vi "TLB Native Dynamic Events ver 0.26f.vi"() -> ()   [LabVIEW 2018]
uses:
  TLB Type Definitions/Intruction Type Definitions.ctl
  TLB Type Definitions/State Type Definitions, for 0.26g versions and later 2.ctl
  <vilib>/Studica/Studica Toolkit/NavX/TypeDefs/Flags/Z900_navX_Flags_OpStatusTypeDef.ctl
  <vilib>/Studica/Studica Toolkit/NavX/TypeDefs/Flags/Z900_navX_Flags_CalibrationStatusTypeDef.ctl
  TLB Type Definitions/Vision cluster.ctl
  TLB Type Definitions/PING CLUSTER.ctl
  TLB Type Definitions/Encoder cluster.ctl
  TLB Type Definitions/Stepper cluster.ctl
  TLB Type Definitions/Yaw Cluster.ctl
  TLB Type Definitions/IR Sensor Type Def.ctl
  TLB Type Definitions/Line Sensor Cluster.ctl
  TLB Type Definitions/Time cluster.ctl
  TLB Type Definitions/Box Colour Detection Cluster (0.26d and above).ctl
  Underlying VI's/FGV's/Box FGV/Box Colour FGV Colours.ctl
  <vilib>/Studica/Studica Toolkit/Background/DIO Channel.ctl
  TLB Type Definitions/Y Stepper cluster.ctl
  TLB Type Definitions/Motor Speed Cluster.ctl
  Labview Training Phase 2/Enum Controls/States for Action Engine.ctl
  Underlying VI's/NavX VI/navX type def.ctl
  <vilib>/Studica/Studica Toolkit/Background/I2C Channel.ctl
  Underlying VI's/I2C Master VI/Arduino_Interfacing.ctl
  Underlying VI's/Motor Control VI with PID/MOTOR CONTROL WITH PID AE DATA MODE TYPE DEF.ctl
  Underlying VI's/Motor Control VI with PID/MOTOR CONTROL WITH PID AE DIRECTION TYPE DEF.ctl
  Experimental VI's/Archived VI's/MOTOR CONTROL NO PID Type Def.ctl
  <vilib>/myRIO/Common/Instrument Driver Framework/myRIO v1.0/AI/typedefs/AI Channels List.ctl
  <vilib>/myRIO/Common/Instrument Driver Framework/myRIO v1.0/AI/typedefs/AI Channels Enum.ctl
  Underlying VI's/Line Sensor AE/Line Sensor AE Type Def.ctl
  Underlying VI's/I2C Master VI/I2C MASTER Type Def.ctl
  Underlying VI's/Elasped Timer/Elapsed timer control.ctl
  Underlying VI's/IMAQ Create Reference AE/IMAQ Reference AE.ctl
  Underlying VI's/FGV's/Box FGV/Box Colour FGV States.ctl
  Underlying VI's/I2C Master VI/I2C_MASTER_WRITE_NEW Type Def.ctl
  Underlying VI's/Modified webcam FGV/Webcam AE.ctl
  <vilib>/userdefined/High Color/IMAQdx.ctl
  <vilib>/Studica/Studica Toolkit/NavX/NavX.lvlib
  <vilib>/NI_Real-Time Target Support.lvlib
panel:
  out "Same colour?":bool
  out "Box Colour Detection":T1
  out "Errors detected":bool
  out "Robot ready":bool
  out "Time cluster":T3
  out "Table IR obstruct":bool
  out "Front IR obstruct":bool
  out "CPU 1 Usage":dbl
  out "CPU 0 Usage":dbl
  out "Line sensors":T4
  out "IR Sensors":T5
  out "NAVX Values":T6
  out "Stepper position values":T7
  out "Encoder values":T8
  out "Ultrasonic sensors":T9
  out "Selected Task":T10=enum."Start Task 9"
  out "Object recognition mode":enum16{"Ball", "Soap", "Gel", "Pipe", "None"}(ring)
  out "Image Processing Error":errorcluster
  out "Object Detection":T11
  out "Status":T14 {"OP Status" items=["INITIALIZING", "SELFTEST_IN_PROGRESS", "ERROR", "IMU_AUTOCAL_IN_PROGRESS", "NORMAL"]; "Calibration Status" items=["IMU_CAL_STATE_MASK"=3, "IMU_CAL_STATE_INPROGRESS"=0, "IMU_CAL_STATE_ACCUMULATE"=1, "IMU_CAL_STATE_COMPLETE"=2]}
  out "General Errors":errorcluster
  in  "Red LED":bool
  out "Front Ultrasonic obstruct":bool
  out "Speed & distance":T15
  out "Task selection":u8
  out "NavX Readings":T16
  out "Arduino Data":T17
  out "TASK ENABLE":bool
  out "Rising Edge":bool
  in  "Green LED":bool
  out "State Logic":T18=enum."Startup"
  out "elements":T10[](array[typedef])
  in  "STOP TASK":bool
  in  "OK Button":bool
  in  "STOP":bool
  out "Queue Errors":errorcluster
  out "Action Queue Items":i32
  out "State Logic Queue Items":i32
  out "Action Queues items":string[](array[string])=["Hardware reset", "Software reset", ""]
  out "Action State":string
  # "VISION"
  # "TLB FRAMEWORK STATUS"
  # "System Health Status Update"
  # "Test Programme written by Calvin Loke    Dated: 28 Aug 2019\nTest Programme revised by Dr Alex See   Dated 30 Aug 2019\n\nRevision date: 20/03/2020\nProgramme version:   TLB Native Dynamic Events ver 0.19a"
  # "0: Task 1\n1: Task 2\n2: Task 3\n3: Task 4\n4: Task 5\n5: Task 6\n6: Task 7\n7: Task 8 Ball\n8: Task 8 Soap\n9: Task 8 Gel\n10: Task 8 Pipe\n11: Task 9 Blue\n12: Task 9 Black\n13: Task 9 Green\n14: Task 9 Red\n15: Task 9 Yellow"
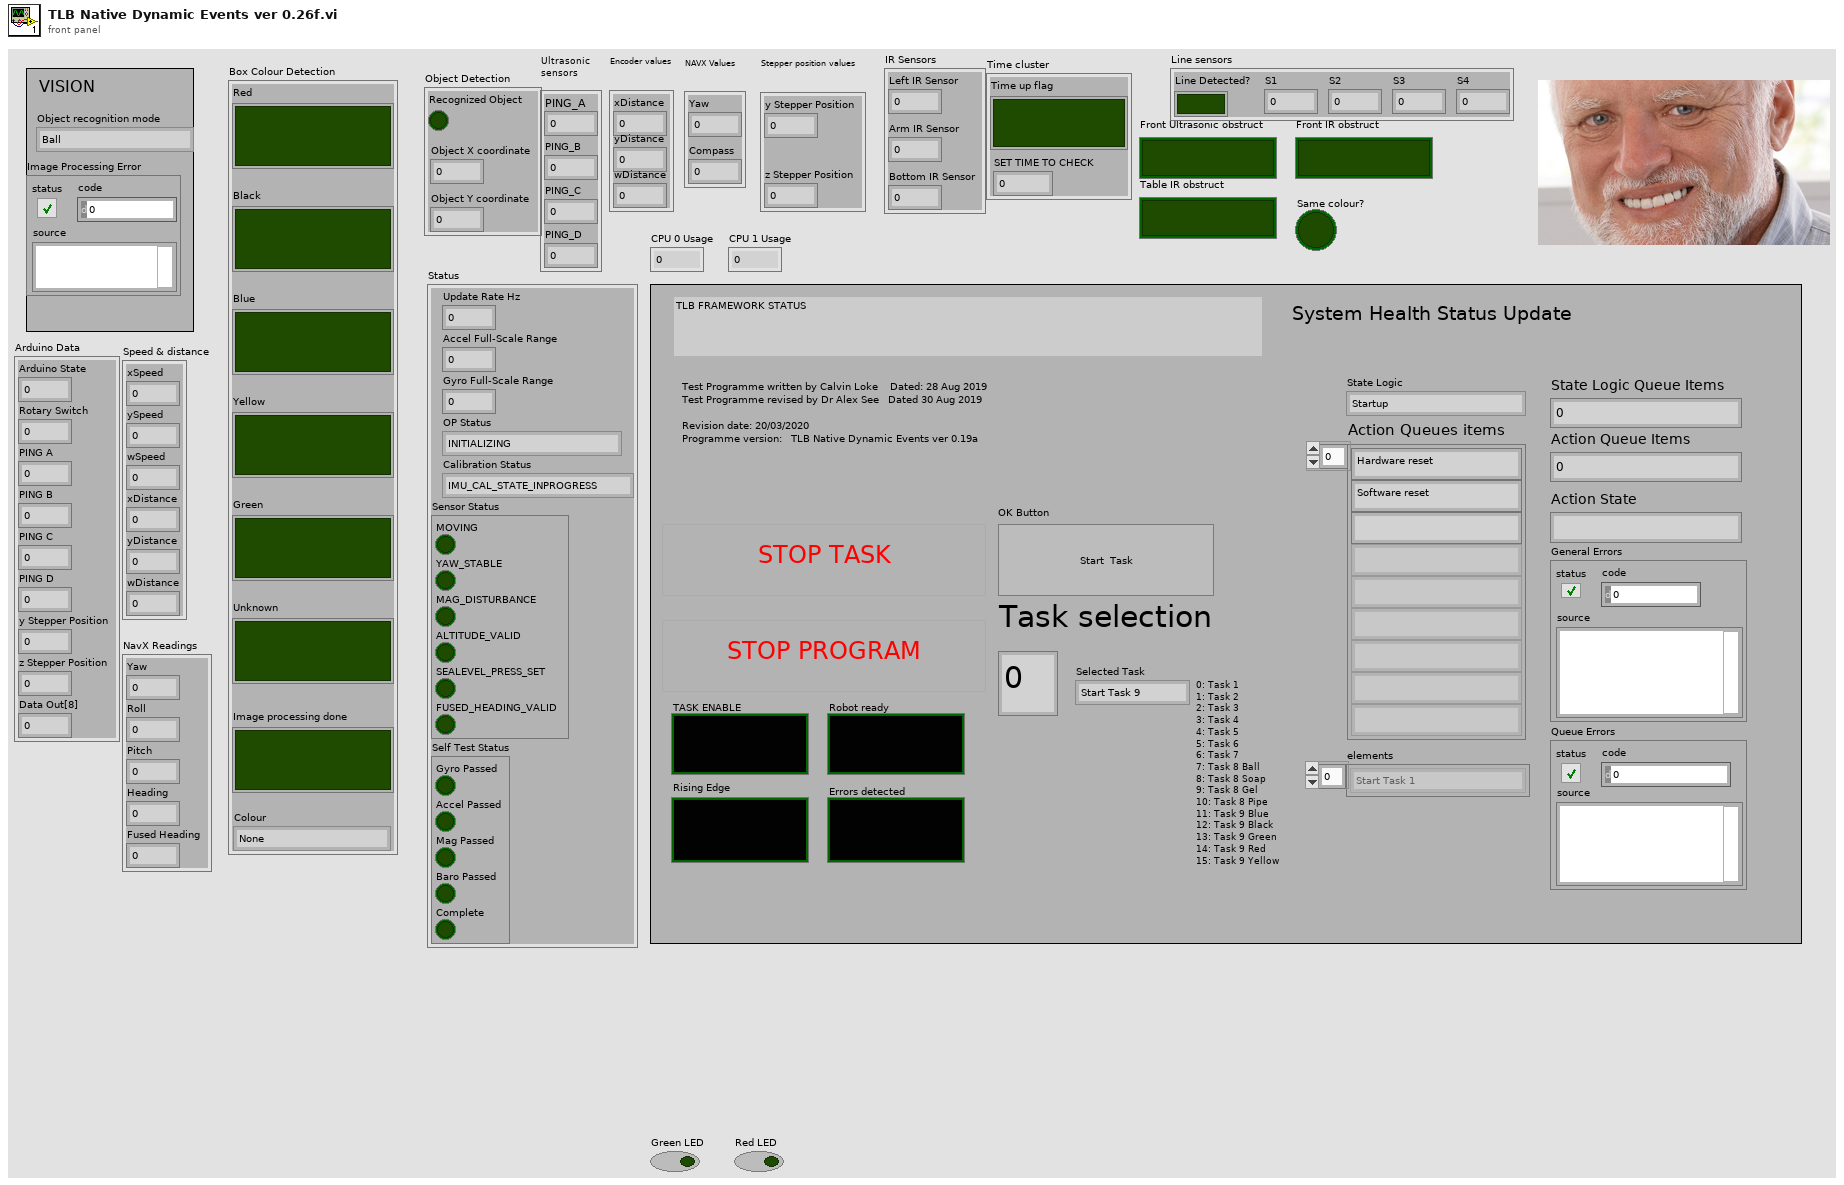
[diagram p1: front panel]
types:
  T1 = typedef "Box Colour Detection Cluster (0.26d and above).ctl" = cluster{"Red":bool, "Black":bool, "Blue":bool, "Yellow":bool, "Green":bool, "Unknown":bool, "Image processing done":bool, "Colour":T2}
  T2 = typedef "Box Colour FGV Colours.ctl" = enum16{"None", "Black", "Blue", "Green", "Red", "Yellow"}
  T3 = typedef "Time cluster.ctl" = cluster{"Time up flag":bool, "SET TIME TO CHECK":dbl}
  T4 = typedef "Line Sensor Cluster.ctl" = cluster{"Line Detected?":bool, "S1":dbl, "S2":dbl, "S3":dbl, "S4":dbl}
  T5 = typedef "IR Sensor Type Def.ctl" = cluster{"Left IR Sensor":dbl, "Arm IR Sensor":dbl, "Bottom IR Sensor":dbl}
  T6 = typedef "Yaw Cluster.ctl" = cluster{"Yaw":dbl, "Compass":dbl}
  T7 = typedef "Stepper cluster.ctl" = cluster{"y Stepper Position":u8, "z Stepper Position":u8}
  T8 = typedef "Encoder cluster.ctl" = cluster{"xDistance":dbl, "yDistance":dbl, "wDistance":dbl}
  T9 = typedef "PING CLUSTER.ctl" = cluster{"PING_A":u8, "PING_B":u8, "PING_C":u8, "PING_D":u8}
  T10 = typedef "Intruction Type Definitions.ctl" = enum16{"None", "Start Task 1", "Start Task 2", "Start Task 3", "Start Task 4", "Start Task 5", "Start Task 6", "Start Task 7", "Start Task 8 - BALL", "Start Task 8 - Gel", "Start Task 8 - Pipe", "Start Task 8 - Soap", "Start Task 9", "Start Task A", "Start Task B", "Exit"}
  T11 = typedef "Vision cluster.ctl" = cluster{"Recognized Object":bool, "Object X coordinate":dbl, "Object Y coordinate":dbl}
  T12 = typedef "NavX.lvlib/Z900_navX_Flags_OpStatusTypeDef.ctl" = u8
  T13 = typedef "NavX.lvlib/Z900_navX_Flags_CalibrationStatusTypeDef.ctl" = u8
  T14 = cluster{"Update Rate Hz":u8, "Accel Full-Scale Range":u8, "Gyro Full-Scale Range":u16, "OP Status":T12, "Calibration Status":T13, "Sensor Status":cluster{"MOVING":bool, "YAW_STABLE":bool, "MAG_DISTURBANCE":bool, "ALTITUDE_VALID":bool, "SEALEVEL_PRESS_SET":bool, "FUSED_HEADING_VALID":bool}, "Self Test Status":cluster{"Gyro Passed":bool, "Accel Passed":bool, "Mag Passed":bool, "Baro Passed":bool, "Complete":bool}}
  T15 = cluster{"xSpeed":dbl, "ySpeed":dbl, "wSpeed":dbl, "xDistance":dbl, "yDistance":dbl, "wDistance":dbl}
  T16 = cluster{"Yaw":dbl, "Roll":dbl, "Pitch":dbl, "Heading":dbl, "Fused Heading":dbl}
  T17 = cluster{"Arduino State":u8, "Rotary Switch":u8, "PING A":u8, "PING B":u8, "PING C":u8, "PING D":u8, "y Stepper Position":u8, "z Stepper Position":u8, "Data Out[8]":u8}
  T18 = typedef "State Type Definitions, for 0.26g versions and later 2.ctl" = enum16{"None", "Startup", "Move to Angle", "True Stop", "Idle", "Shutdown", "Task 1A", "Task 1B", "Task 2:Raise Arm", "Task 2:Sensor Mode", "Task 2:Reverse Mode", "Task 3", "Task 4_A", "Task 4_B", "Task 4_C", "Task 4_D", "Task 5A", "Task 5B", "Task 5C", "Task 5D", "Task 5E: POSITION ARM", "Task 5F: ARM GRAB HEIGHT", "Task 5G: CLOSE CLAW", "Task 5H: RAISE ARM", "Task 6_A", "Task 6_B", "Task 7", "Task 8A: RAISE ARM", "Task 8B: MOVE TO BOX", "Task 8C: CAM BURST", "Task 8D: PROCESS IMAGE", "Task 8E: ROBOT ADJUST", "Task 8F: CAM BURST 2", "Task 8G: PROCESS IMAGE 2", "Task 8H: ARM ADJUST", "Task 8I: ARM GRAB HEIGHT", "Task 8J: CLOSE CLAW", "Task 8K: RAISE MY SWORD", "Task 9A: Raise Arm", "Task 9B: Rotate to Angle", "Task 9C: Detect Box", "Task 9D: MOVE FORWARD", "Task 9E: MOVE LEFT", "Task 9F: SCAN BOX", "Task 9G: MOVE RIGHT", "Task 9H: SCAN BOX 2", "Task 9I: ROTATE 90 CW", "Task 9J: FORWARD", "Task 9K: MOVE RIGHT", "Task 9L: SCAN BOX 3", "Task 9M: MOVE RIGHT", "Task 9N: SCAN BOX 4", "PENIS", "PENIS 2", "PENIS 3", "Task 9R: PROCESS COLOUR", "Task A1: Task 9 Open cam", "Task A2: Task 9 Move Arm", "Task A3: Task 9 Set Timer", "Task A4: Tasl 9 Capture images", "Task A5: Task 9 Close camera", "Task A6: Process Colour", "Task A7: Dispose Camera Buffer"}
  T19 = typedef "Motor Speed Cluster.ctl" = cluster{"ySpeed":dbl, "xSpeed":dbl, "wSpeed":dbl}
  T20 = typedef "Y Stepper cluster.ctl" = cluster{"yStepper desired":u8}
  T21 = typedef "DIO Channel.ctl" = enum16{"Not Connected", "A/DIO1", "A/DIO2", "A/DIO3", "A/DIO4", "A/DIO5", "A/DIO6", "A/DIO7", "A/DIO13", "B/DIO1", "B/DIO2", "B/DIO3", "B/DIO4", "B/DIO5", "B/DIO6", "B/DIO7", "B/DIO13", "C/DIO0", "C/DIO1", "C/DIO2", "C/DIO3", "C/DIO4", "C/DIO5", "C/DIO6", "C/DIO7"}
  T22 = cluster{"DIO Channel":T21, "FPGA VI Reference Out":refnum<k20>}
  T23 = typedef "States for Action Engine.ctl" = enum16{"Initialize", "Write", "Read"}
  T24 = typedef "NI_Real-Time Target Support.lvlib/RT CPU Load.ctl" = cluster{"Total (%)":dbl, "Time Critical (%)":dbl, "Timed Structures (%)":dbl, "High (%)":dbl, "Above Normal (%)":dbl, "Normal (%)":dbl, "Background (%)":dbl, "Idle (%)":dbl, "ISR (%)":dbl}
  T25 = cluster{"CPU loads[0]":T24, "CPU loads[1]":T24, "CPU loads[2]":T24, "CPU loads[3]":T24, "CPU loads[4]":T24, "CPU loads[5]":T24, "CPU loads[6]":T24, "CPU loads[7]":T24, "CPU loads[8]":T24}
  T26 = typedef "navX type def.ctl" = enum16{"Get i2C reference", "Read Values", "Zero Yaw"}
  T27 = typedef "Arduino_Interfacing.ctl" = enum16{"Initialize", "Write to Arduino", "Read From Arduino"}
  T28 = typedef "I2C Channel.ctl" = enum16{"Not Connected", "A", "B"}
  T29 = cluster{"I2C Ref Out":cluster{"I2C Channel":T28, "FPGA VI Reference Out":refnum<k20>}, "Connected":bool, "Slave Address (7-bit)":u8, "Registry":u8[]}
  T30 = typedef "Box Colour FGV States.ctl" = enum16{"Initialize", "Read", "Write"}
  T31 = typedef "MOTOR CONTROL WITH PID AE DIRECTION TYPE DEF.ctl" = enum16{"y-axis movement", "x-axis movement", "rotation", "stop", "reset encoders"}
  T32 = typedef "MOTOR CONTROL WITH PID AE DATA MODE TYPE DEF.ctl" = enum16{"Init AE", "Write to AE", "Read from AE"}
  T33 = typedef "Line Sensor AE Type Def.ctl" = enum16{"INIT AE", "READ FROM LINE SENSORS"}
  T34 = typedef "IMAQ Reference AE.ctl" = enum16{"Initialize AE", "Get IMAQ Reference", "Dispose Processing Buffer"}
  T35 = typedef "Elapsed timer control.ctl" = enum16{"Start", "Pause", "Initialize"}
  T36 = typedef "I2C_MASTER_WRITE_NEW Type Def.ctl" = enum16{"Ultrasonic sensors", "Stepper origin", "zStepper 13.3k", "zStepper 13k", "zStepper 12k", "zStepper 11k", "zStepper 10k", "zStepper 9k", "zStepper 8k", "zStepper 7k", "zStepper 6k", "zStepper 5k", "zStepper 4k", "zStepper 3k", "zStepper 2k", "zStepper 1k", "zStepper 900", "zStepper 800", "zStepper 700", "zStepper 600", "zStepper 500", "zStepper 400", "zStepper 300", "zStepper 200", "zStepper 100", "zStepper 0", "yStepper control", "Open Claw", "Close Claw", "Soft Reset"}
  T37 = typedef "Webcam AE.ctl" = enum16{"Initialize Camera", "Open Camera", "Continuous Acquisition", "Close Camera", "Retrieve Image", "Dispose Camera Image Buffer"}
  T38 = typedef "IMAQdx.ctl" = refnum<k21>
  T39 = typedef "MOTOR CONTROL NO PID Type Def.ctl" = enum16{"Init", "Front Back", "Left Right", "Rotate", "Stop", "Latch"}
  T40 = typedef "AI Channels List.ctl" = T41[]
  T41 = typedef "AI Channels Enum.ctl" = enum16{"Not Connected", "AudioIn/Left", "AudioIn/Right", "C/AI0", "C/AI1", "A/AI0", "A/AI1", "A/AI2", "A/AI3", "A/AI4", "A/AI5", "A/AI6", "A/AI7", "B/AI0", "B/AI1", "B/AI2", "B/AI3", "B/AI4", "B/AI5", "B/AI6", "B/AI7", "AI/AI0", "AI/AI1", "AI/AI2", "AI/AI3", "A/AI0 (DIFF)", "A/AI1 (DIFF)", "A/AI2 (DIFF)", "A/AI3 (DIFF)", "B/AI0 (DIFF)", "B/AI1 (DIFF)", "B/AI2 (DIFF)", "B/AI3 (DIFF)"}
  T42 = cluster{"S1":dbl, "S2":dbl, "S3":dbl, "S4":dbl, "Array[4]":dbl, "Array[5]":dbl, "Array[6]":dbl, "Array[7]":dbl, "Array[8]":dbl}
  T43 = typedef "I2C MASTER Type Def.ctl" = enum16{"Last State", "Mode 0", "Mode 1", "Mode 2", "Mode 3", "Mode 4", "Mode 5", "Mode 6", "Mode 7", "Mode 8", "Mode 9", "Mode 10"}
  T44 = typedef "IMAQ Image.ctl" = refnum<image>
  T45 = cluster{"Number of Matches":i32, "Object detected?":bool}
  T46 = cluster{"Red":bool, "Black":bool, "Blue":bool, "Yellow":bool, "Green":bool, "No recognizable coolour":bool}
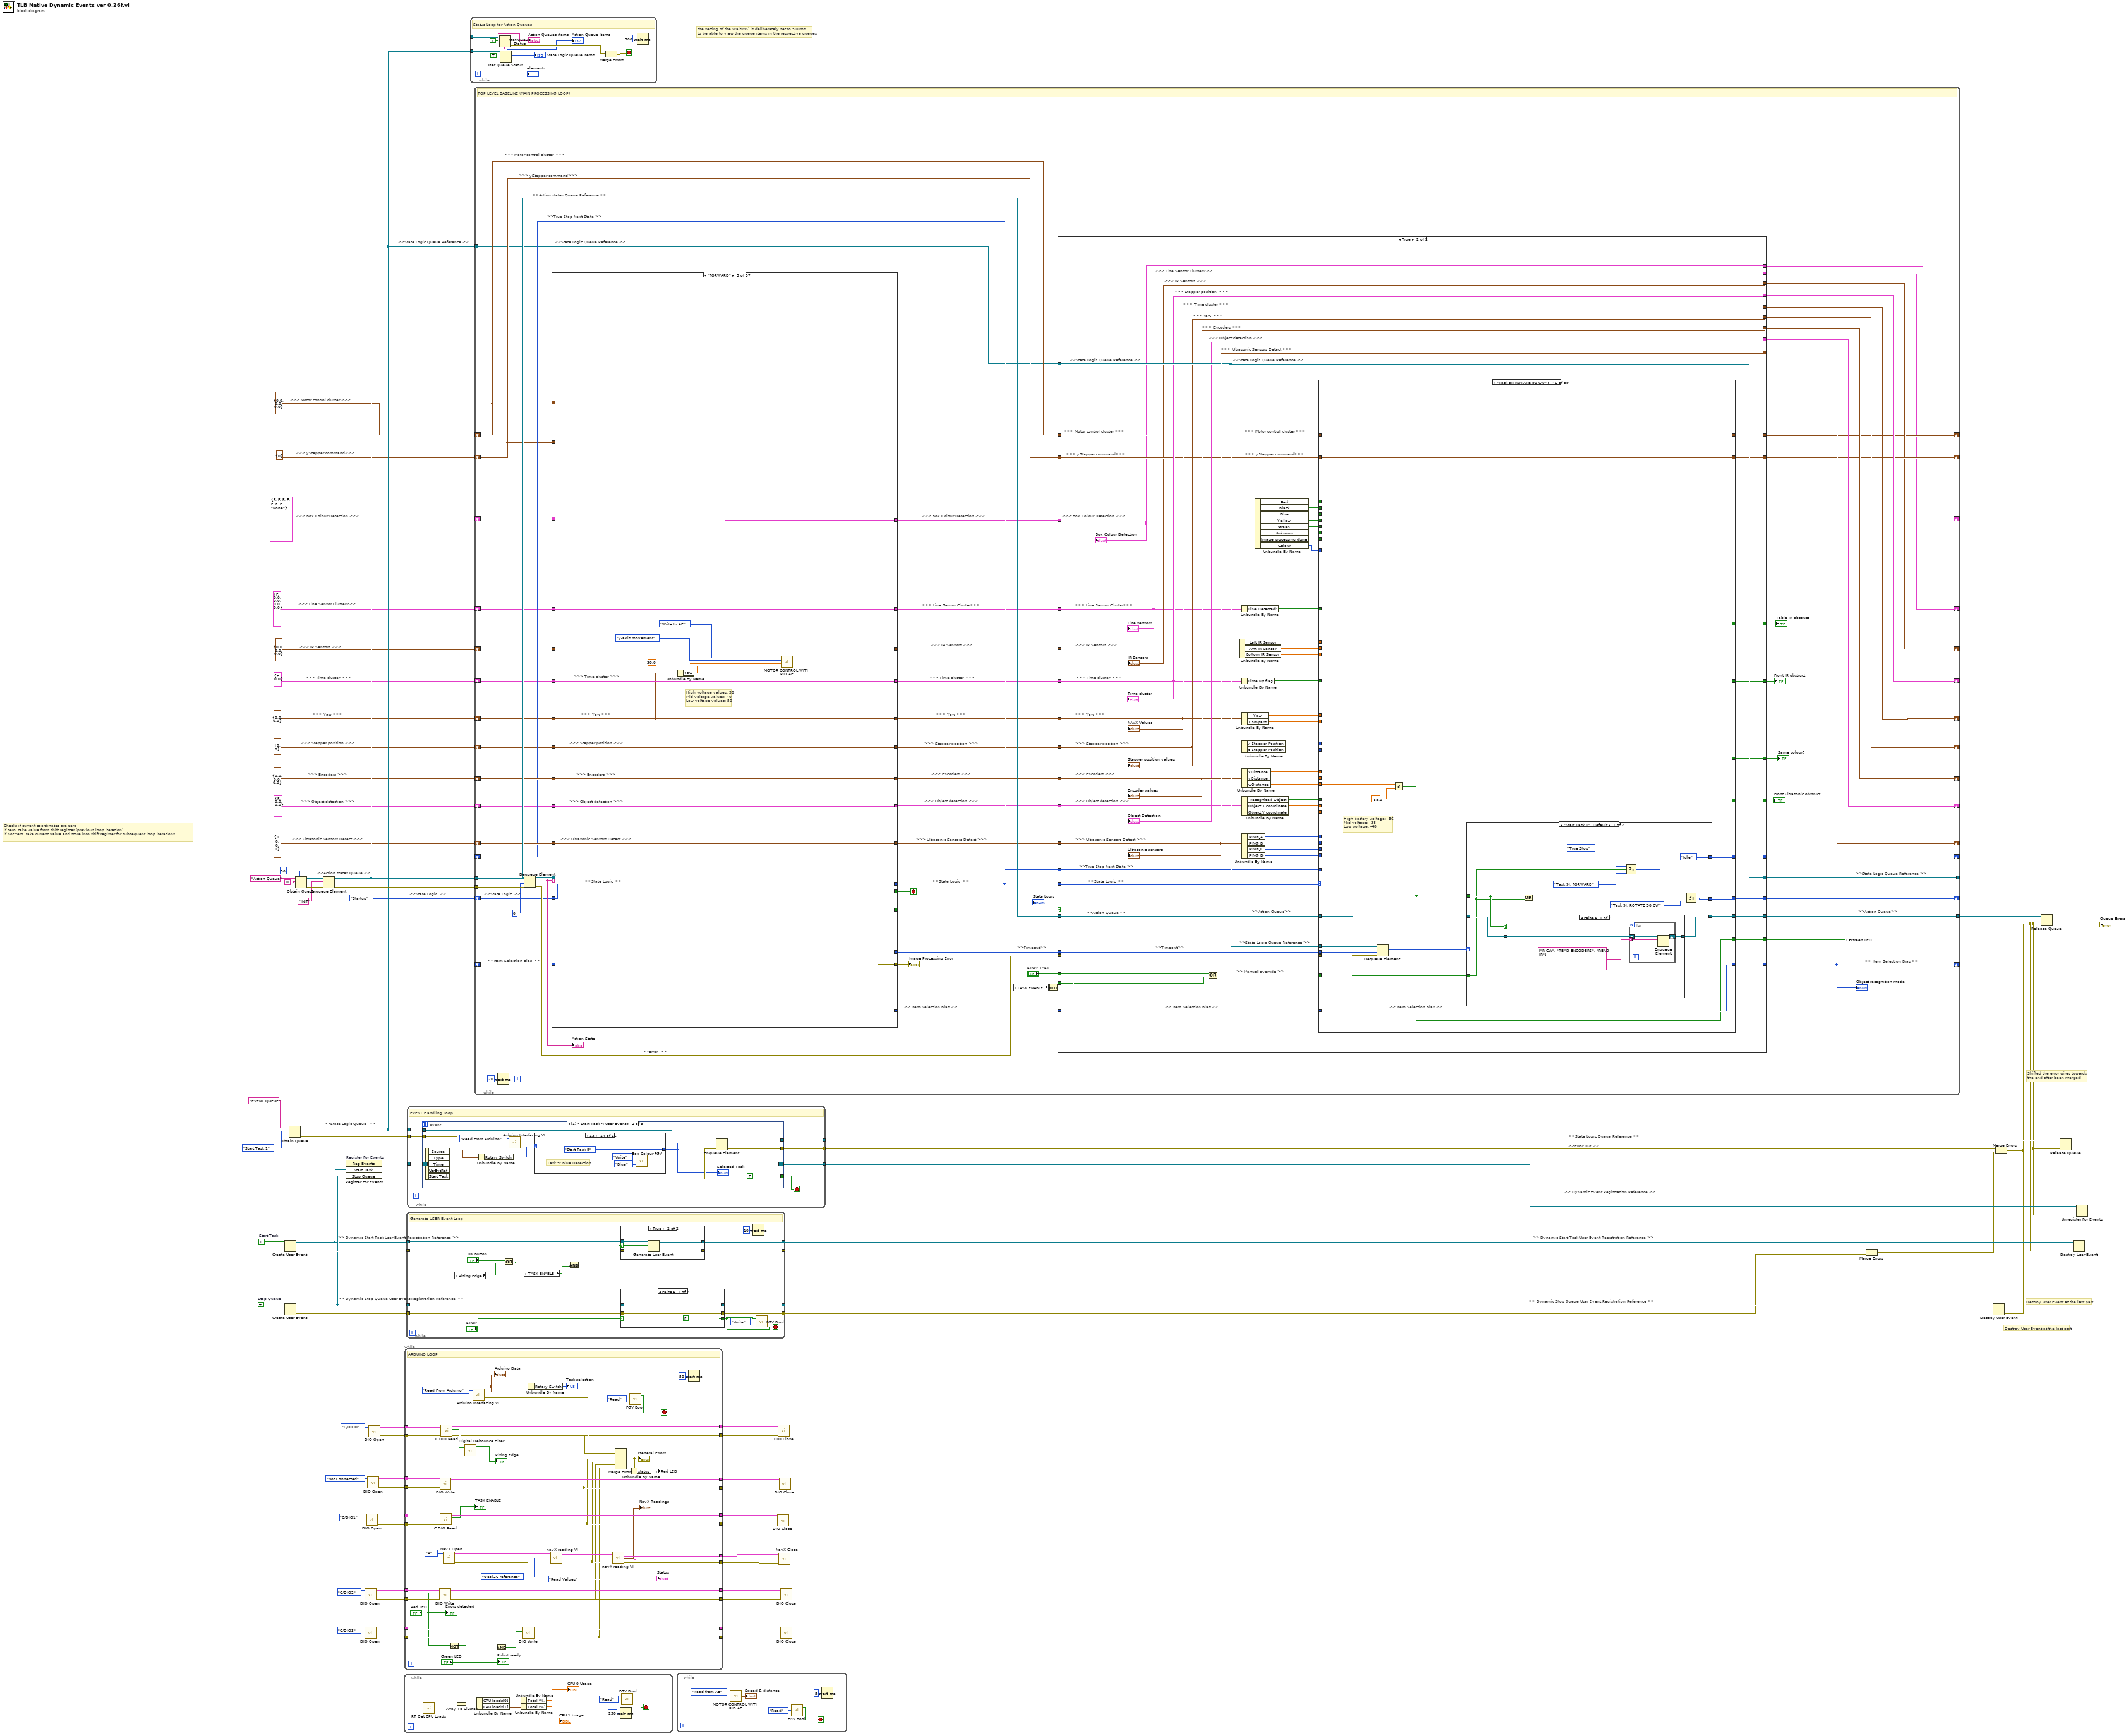
[diagram p0: block diagram]
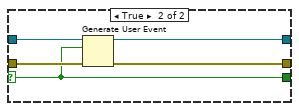
[diagram p2: hidden frame]
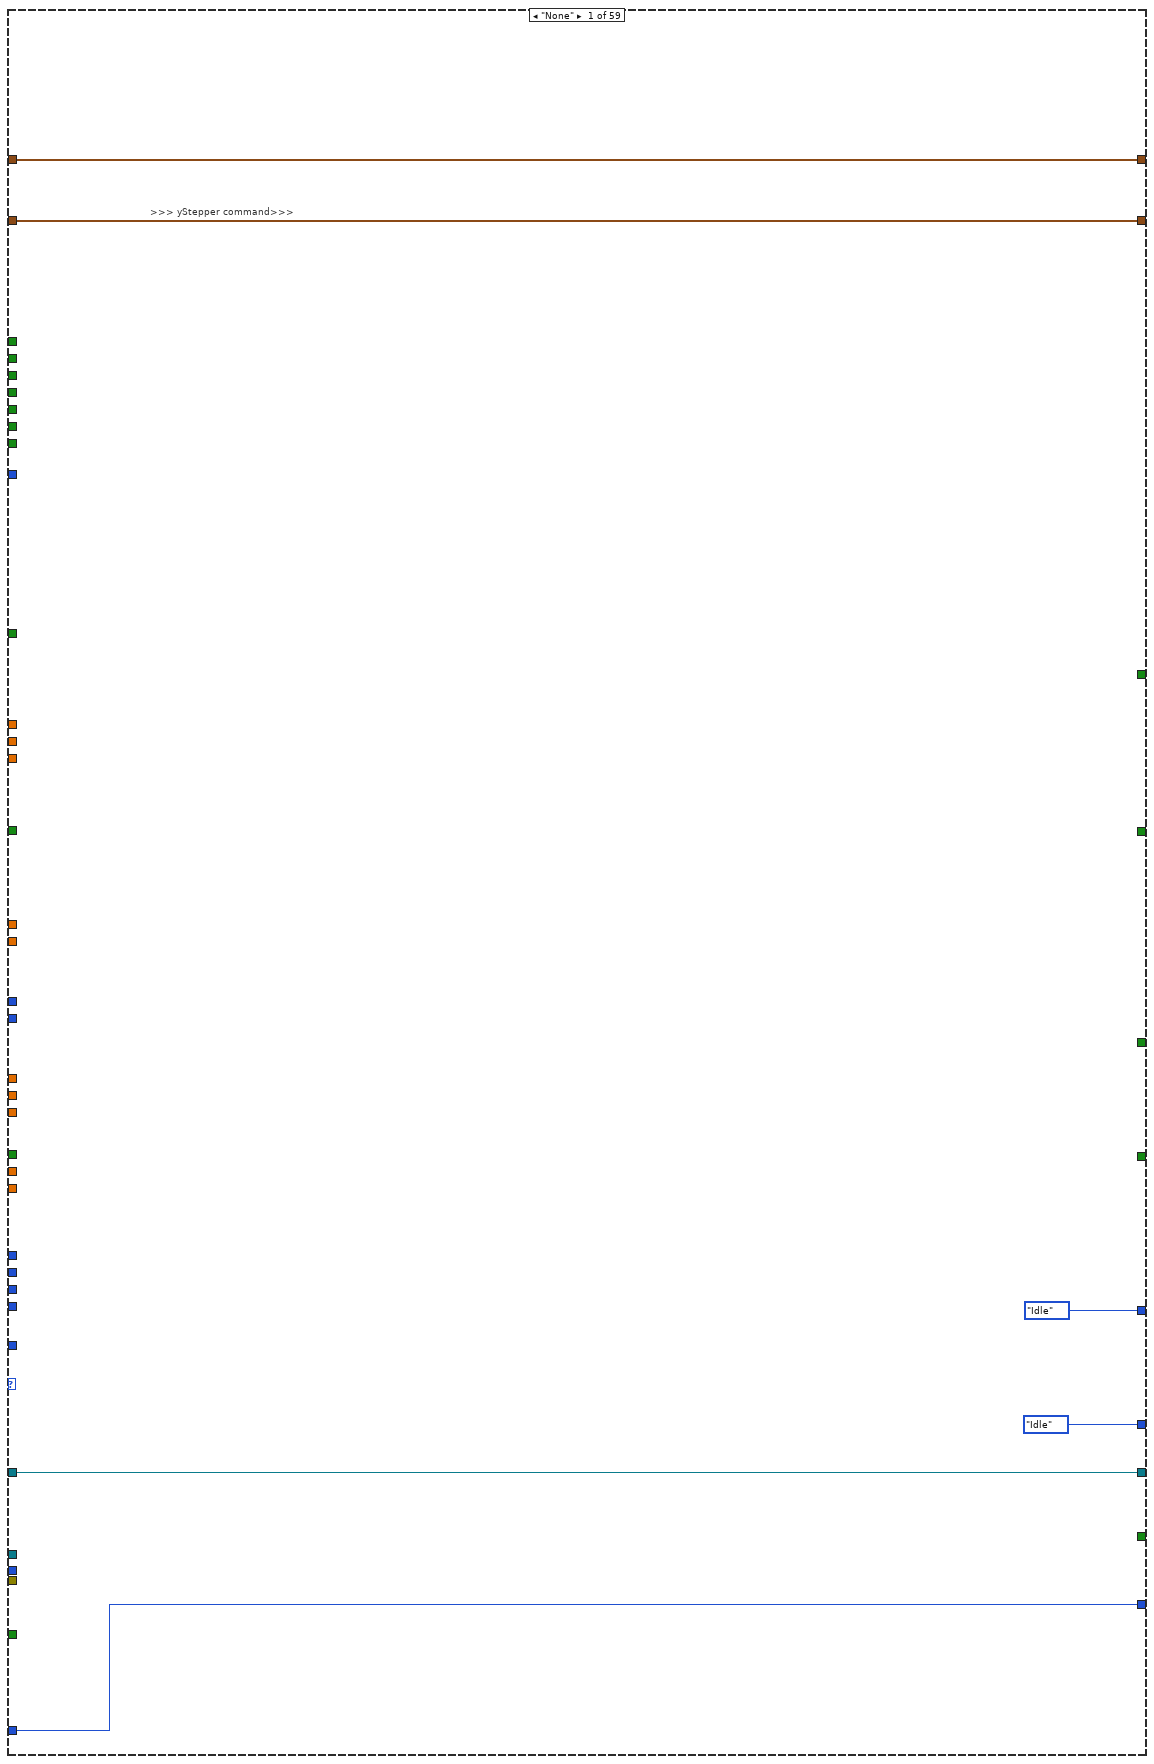
[diagram p5: hidden frame]
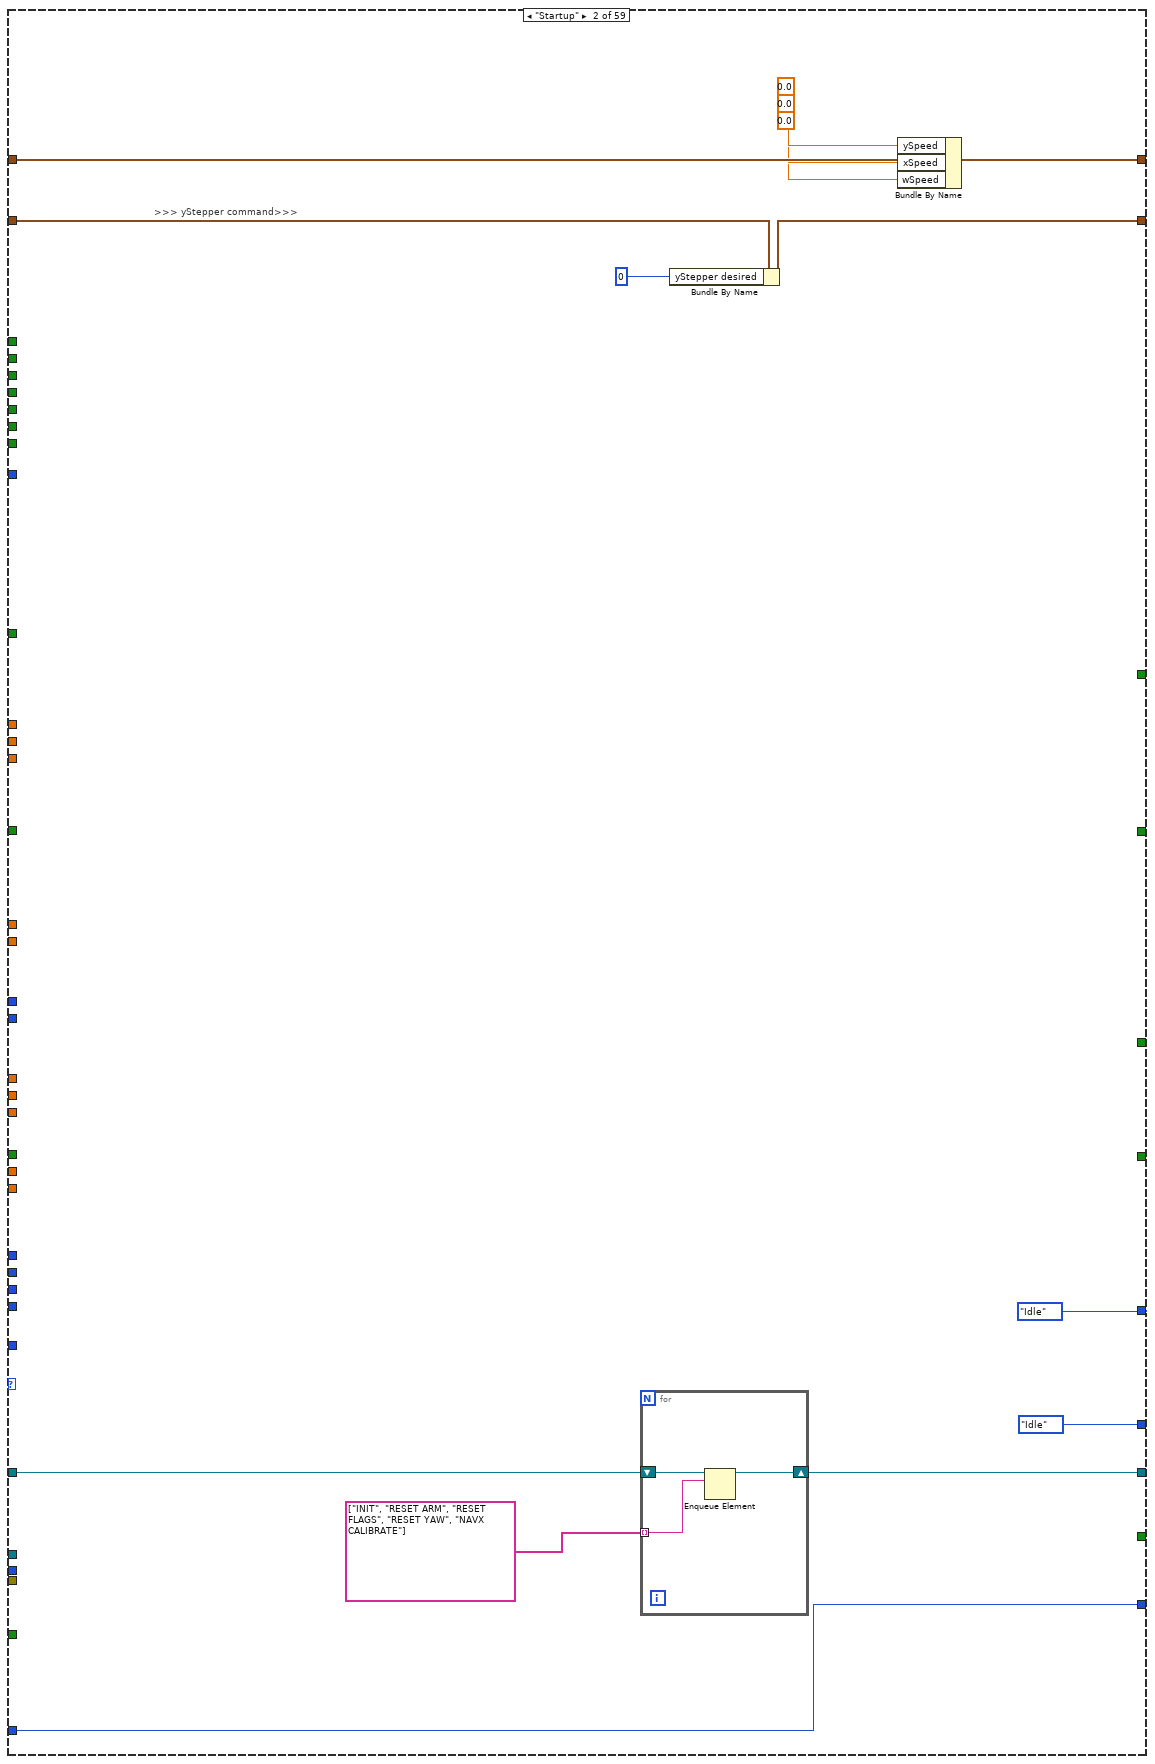
[diagram p6: hidden frame]
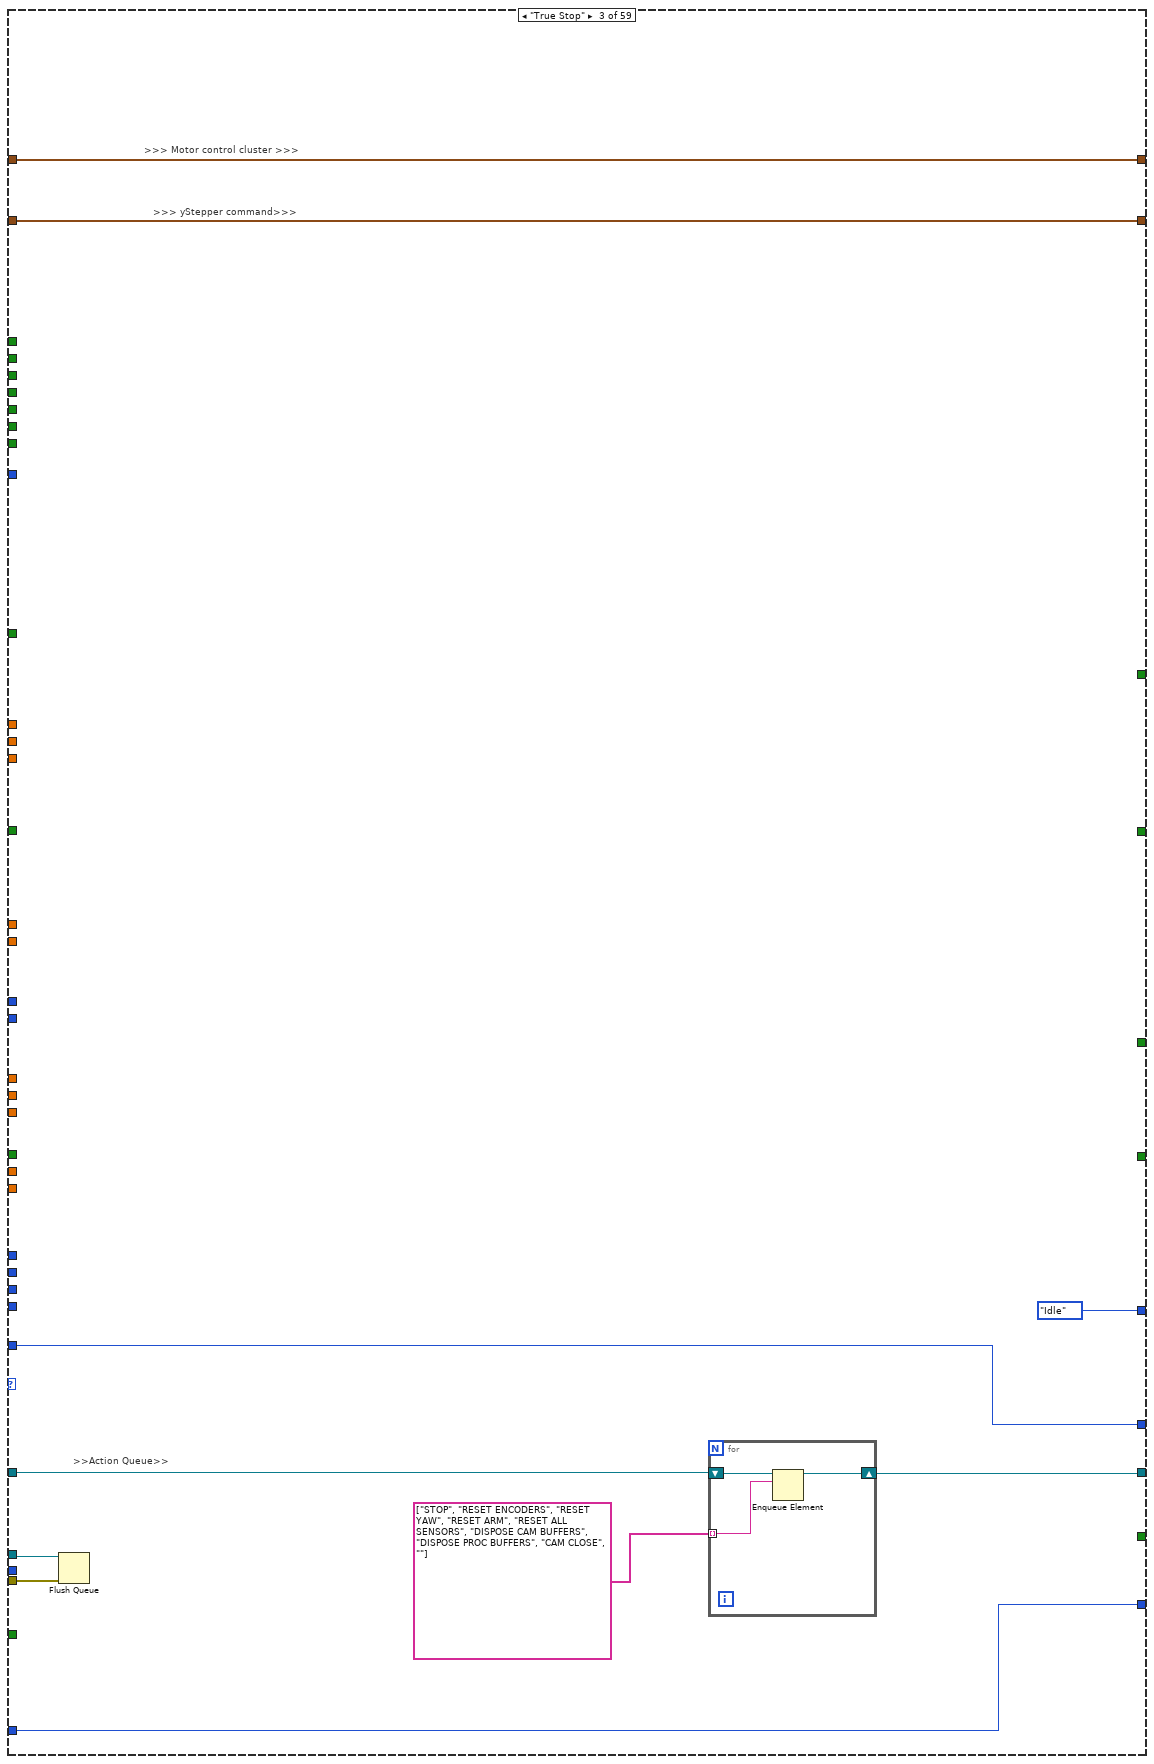
[diagram p7: hidden frame]
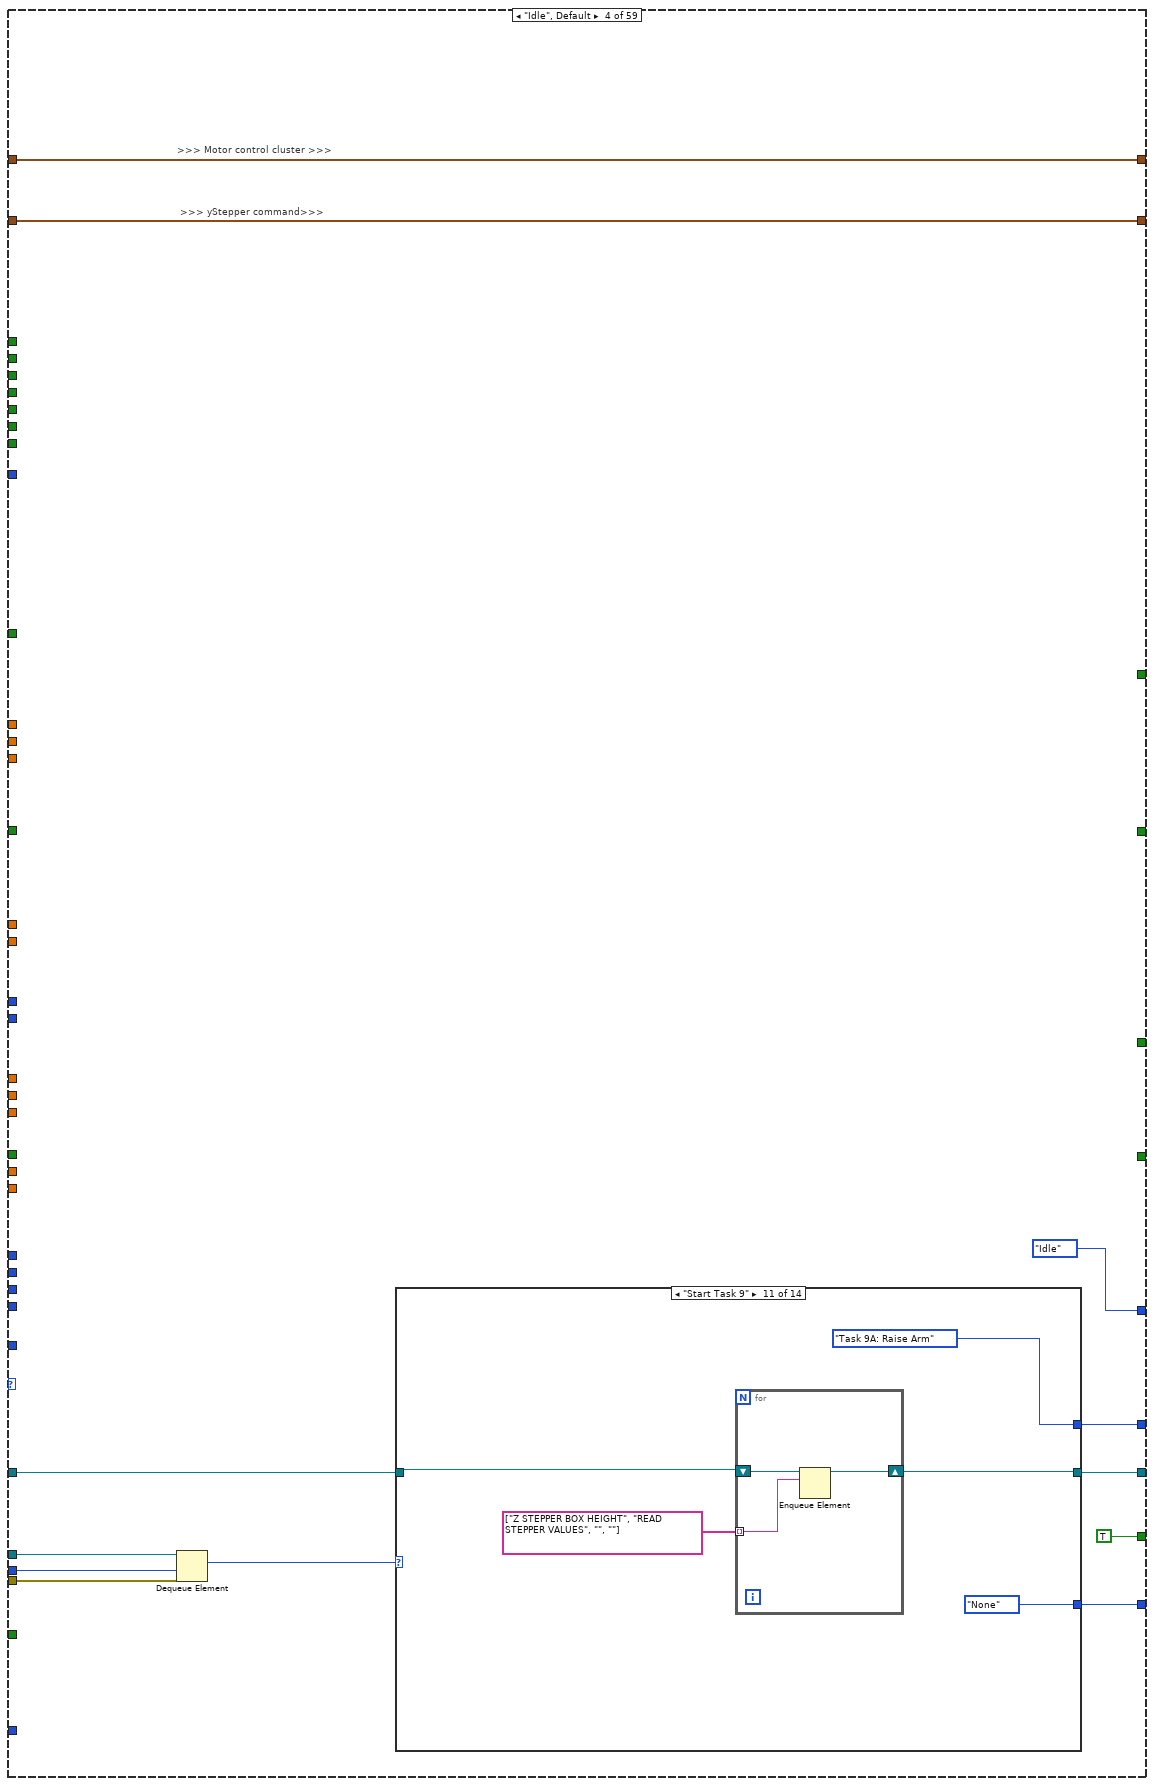
[diagram p8: hidden frame]
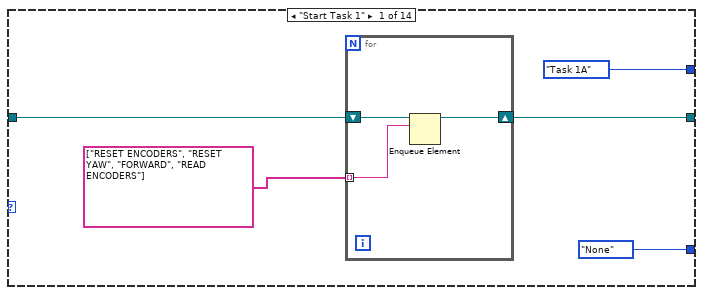
[diagram p9: hidden frame]
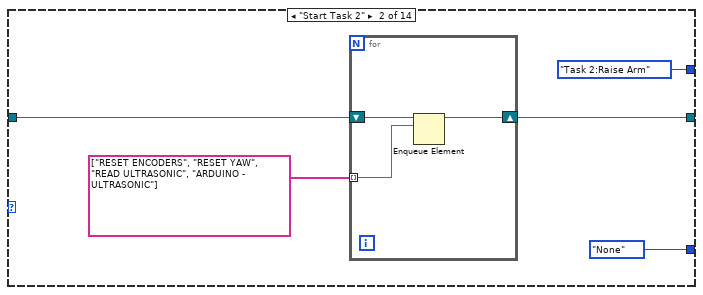
[diagram p10: hidden frame]
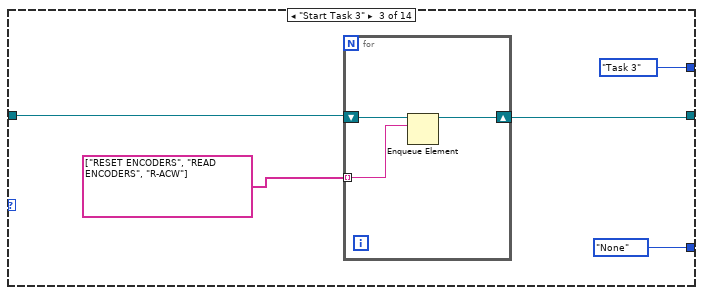
[diagram p11: hidden frame]
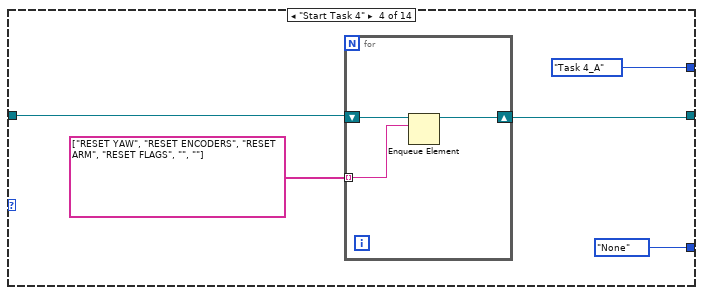
[diagram p12: hidden frame]
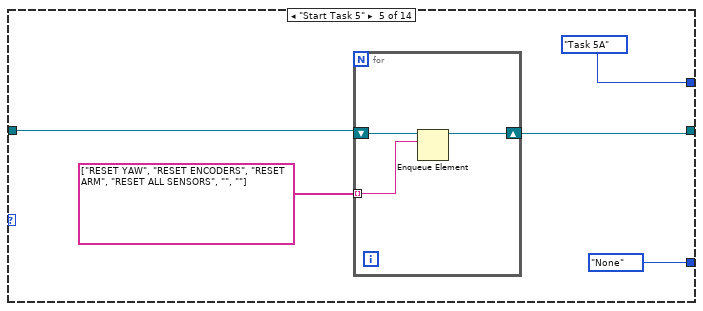
[diagram p13: hidden frame]
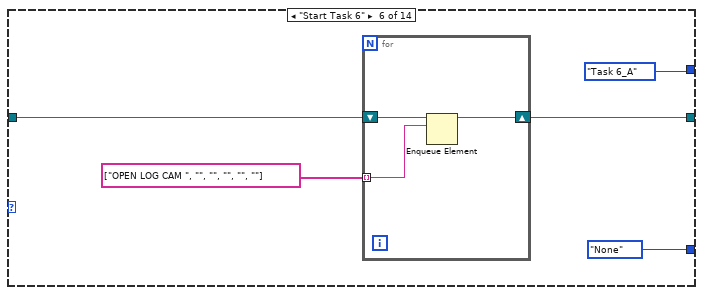
[diagram p14: hidden frame]
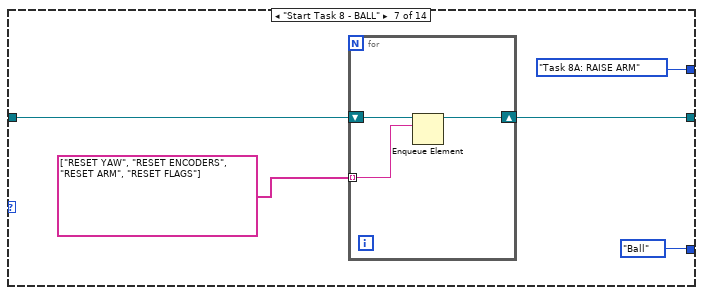
[diagram p15: hidden frame]
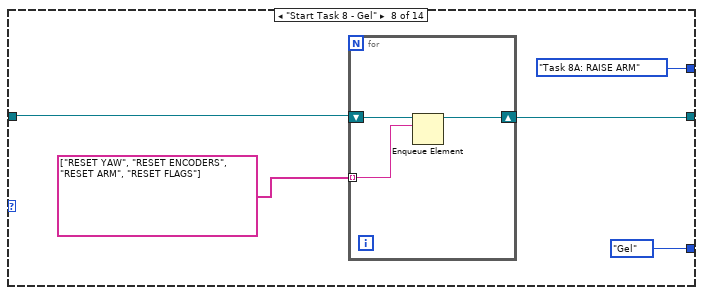
[diagram p16: hidden frame]
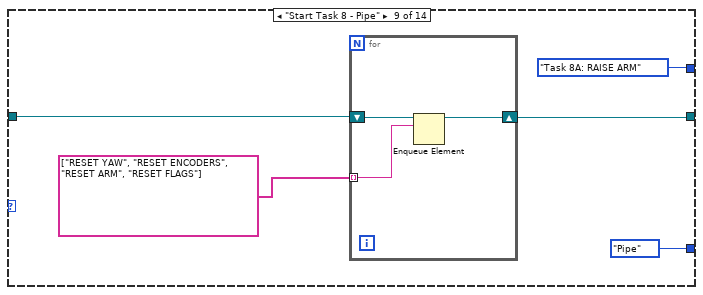
[diagram p17: hidden frame]
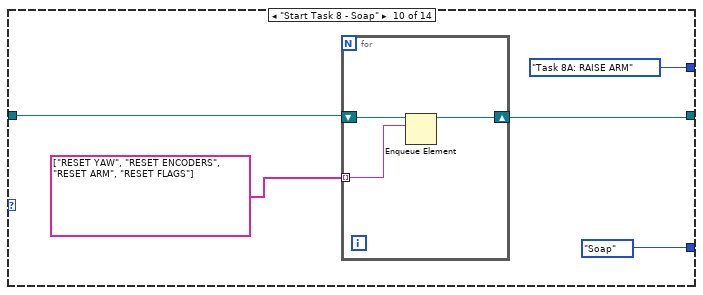
[diagram p18: hidden frame]
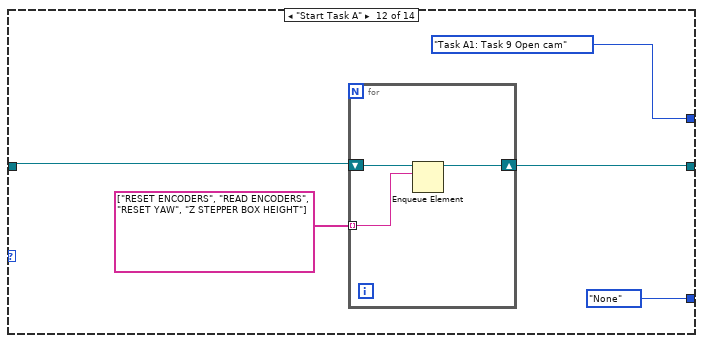
[diagram p19: hidden frame]
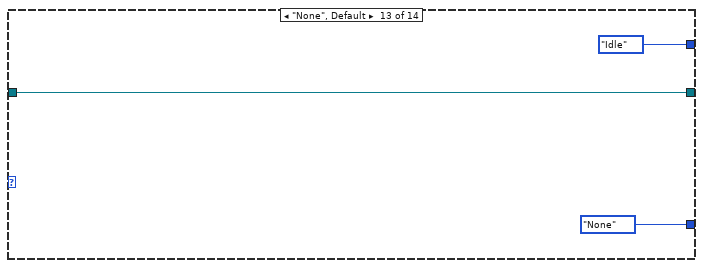
[diagram p20: hidden frame]
diagram:
  w69 = TRUE  # Stop Queue
  w68 = TRUE  # Start Task
  # ">>> Box Colour Detection >>>"
  # ">>State Logic Queue Reference >>"
  # ">>State Logic  >>"
  # ">>> Line Sensor Cluster>>>"
  # ">>> Motor control cluster >>>"
  # ">>> IR Sensors >>>"
  # "Checks if current coordinates are zero\nif zero, take value from shift register (previous loop iteration)\nif not zero, take current value and store into shift register for subsequent loop iterations"
  # ">>> yStepper command>>>"
  # ">>> Time cluster >>>"
  # ">>> Yaw >>>"
  # ">>> Stepper position >>>"
  # ">>> Encoders >>>"
  # ">>> Object detection >>>"
  # ">>> Ultrasonic Sensors Detect >>>"
  # "the setting of the Wait(MS) is deliberately set to 500ms\nto be able to view the queue items in the respective queues"
  # ">>Error Out >>"
  # ">> Dynamic Stop Queue User Event Registration Reference >>"
  # ">> Dynamic Start Task User Event Registration Reference >>"
  # ">> Dynamic Stop Queue User Event Registration Reference >>"
  # ">> Dynamic Start Task User Event Registration Reference >>"
  # ">> Dynamic Event Registration Reference >>"
  # ">>Action states Queue >>"
  # ">>State Logic Queue  >>"
  # ">>State Logic Queue Reference >>"
  # "Destroy User Event at the last part"
  # "Destroy User Event at the last part"
  # "Shifted the error wires towards\nthe end after been merged"
  n1 = Create User Event(user event datatype=w68) -> (user event=w60:refnum<user-event>, error out=w65:errorcluster)  [unwired: 1 in]
  n2 = Create User Event(user event datatype=w69) -> (user event=w61:refnum<user-event>, error out=w64:errorcluster)  [unwired: 1 in]
  n3 = Obtain Queue(name (unnamed)="EVENT QUEUE", element data type=Intruction_Type_Definitions."Start Task 1" ("Enum")) -> (queue out=w46:refnum<queue>, error out=w52:errorcluster)  [unwired: 3 in, 1 out]
  n4 = Obtain Queue(max queue size (-1, unlimited)=50, name (unnamed)="Action Queue", element data type="") -> (queue out=w55:refnum<queue>, error out=w51:errorcluster)  [unwired: 2 in, 1 out]
  n5 = Enqueue Element(queue=w55, element="INIT", error in (no error)=w51) -> (queue out=w47:refnum<queue>, error out=w50:errorcluster)  [unwired: 1 in, 1 out]
  n6 = register-events "Register For Events"(w60, w61) -> (reference out=w59:refnum<event-registration>)  [unwired: 2 in, 1 out]
  n7 = call <vilib>:"DIO Open.vi"("DIO Channel"=DIO_Channel."C/DIO2") -> ("error out"=w19:errorcluster, "DIO Info Out"=w20:T22)  [unwired: 9 in]
  n8 = call <vilib>:"DIO Open.vi"("DIO Channel"=DIO_Channel."C/DIO3") -> ("error out"=w14:errorcluster, "DIO Info Out"=w15:T22)  [unwired: 9 in]
  n9 = call <vilib>:"DIO Open.vi"("DIO Channel"=DIO_Channel."C/DIO1") -> ("error out"=w24:errorcluster, "DIO Info Out"=w25:T22)  [unwired: 9 in]
  n10 = call <vilib>:"DIO Open.vi"("DIO Channel"=DIO_Channel."Not Connected") -> ("error out"=w29:errorcluster, "DIO Info Out"=w31:T22)  [unwired: 9 in]
  n11 = call <vilib>:"DIO Open.vi"("DIO Channel"=DIO_Channel."C/DIO0") -> ("error out"=w34:errorcluster, "DIO Info Out"=w37:T22)  [unwired: 9 in]
  n12 = while {
    stop <- w76 stop-if-true
    n13 = call <vilib>:"RT Get CPU Loads.vi"() -> ("CPU loads"=w75:T24[])  [unwired: 10 in, 1 out]
    n14 = Array To Cluster(array=w75) -> (cluster=w74:T25)
    n15 = Unbundle By Name(w74) -> ("CPU loads[0]"=w73:T24, "CPU loads[1]"=w72:T24)
    n16 = Unbundle By Name(w73) -> ("Total (%)"=→"CPU 0 Usage":dbl)
    n17 = Unbundle By Name(w72) -> ("Total (%)"=→"CPU 1 Usage":dbl)
    n18 = Wait (ms)(milliseconds to wait=u32 250) -> ()  [unwired: 1 out]
    n19 = call "FGV Bool.vi"("Init/Read/Write State"=States_for_Action_Engine."Read") -> ("Output node"=w76:bool)  [unwired: 2 in, 1 out]
  }
  n20 = while {
    tunnel: w37 -> [w122]
    tunnel: [w121] -> w35
    tunnel: w34 -> [w120]
    tunnel: [w91] -> w33
    tunnel: w31 -> [w117]
    tunnel: [w116] -> w30
    tunnel: w29 -> [w115]
    tunnel: [w90] -> w28
    tunnel: [w114] -> w26
    tunnel: w25 -> [w113]
    tunnel: w24 -> [w112]
    tunnel: [w89] -> w23
    tunnel: w20 -> [w106]
    tunnel: w19 -> [w105]
    tunnel: [w104] -> w18
    tunnel: [w87] -> w17
    tunnel: w15 -> [w103]
    tunnel: w14 -> [w102]
    tunnel: [w101] -> w13
    tunnel: [w86] -> w12
    tunnel: [w98] -> w9
    tunnel: [w97] -> w10
    stop <- w124 stop-if-true
    # "ARDUINO LOOP"
    n21 = call <vilib>:"DIO Write.vi"("error in (no error)"=w105, "Input"="Red LED", "DIO Info In"=w106) -> ("error out"=w87:errorcluster, "DIO Info Out"=w104:T22)  [unwired: 7 in]
    n22 = call <vilib>:"DIO Write.vi"("error in (no error)"=w115, "DIO Info In"=w117) -> ("error out"=w90:errorcluster, "DIO Info Out"=w116:T22)  [unwired: 8 in]
    n23 = call <vilib>:"C DIO Read.vi"("error in (no error)"=w112, "DIO Info In in"=w113) -> ("error out"=w89:errorcluster, "IN"=→"TASK ENABLE":bool, "DIO Info In out"=w114:T22)  [unwired: 7 in]
    n24 = call <vilib>:"C DIO Read.vi"("error in (no error)"=w120, "DIO Info In in"=w122) -> ("error out"=w91:errorcluster, "IN"=w119:bool, "DIO Info In out"=w121:T22)  [unwired: 7 in]
    n25 = call <vilib>:"NavX Open.vi"("I2C Channel"=I2C_Channel."A") -> ("error out"=w108:errorcluster, "NavX Info"=w110:T29)  [unwired: 9 in]
    n26 = Not(x="Red LED") -> (.not. x?=w81:bool)
    n27 = call "Digital Debounce Filter.vi"("Boolean input"=w119) -> ("Rising Edge"=→"Rising Edge":bool)  [unwired: 1 in, 2 out]
    n28 = call "Arduino Interfacing VI.vi"("AE Mode"=Arduino_Interfacing."Read From Arduino") -> ("error out"=w92:errorcluster, "Arduino Data"=w94:T17)  [unwired: 3 in]
    "Arduino Data" <- w94
    n29 = And(x=w81, y="Green LED") -> (x .and. y?=w83:bool)
    n30 = call <vilib>:"DIO Write.vi"("error in (no error)"=w102, "Input"=w83, "DIO Info In"=w103) -> ("error out"=w86:errorcluster, "DIO Info Out"=w101:T22)  [unwired: 7 in]
    n31 = Unbundle By Name(w94) -> ("Rotary Switch"=→"Task selection":u8)
    n32 = call "navX reading VI.vi"("NavX Info In"=w110, "Mode"=navX_type_def."Get i2C reference", "error in (no error)"=w108) -> ("NavX Info Out"=w99:T29, "Error Out"=w88:errorcluster)  [unwired: 2 out]
    n33 = call "navX reading VI.vi"("NavX Info In"=w99, "Mode"=navX_type_def."Read Values", "error in (no error)"=w88) -> ("NavX Info Out"=w98:T29, "NavX Readings"=→"NavX Readings":T16, "Status"=→"Status":T14, "Error Out"=w97:errorcluster)
    n34 = Merge Errors(w92, w91, w90, w89, w88, w87, w86) -> (w84:errorcluster)
    "General Errors" <- w84
    n35 = call "FGV Bool.vi"("Init/Read/Write State"=States_for_Action_Engine."Read") -> ("Output node"=w124:bool)  [unwired: 2 in, 1 out]
    n36 = Unbundle By Name(w84) -> ("status"=w82:bool)
    n37 = local write "Red LED"(w82) -> ()
    n38 = Wait (ms)(milliseconds to wait=u32 50) -> ()  [unwired: 1 out]
    "Robot ready" <- "Green LED"
    "Errors detected" <- "Red LED"
  }
  n39 = while {
    tunnel: w60 -> [w142]
    tunnel: w61 -> [w141]
    tunnel: [w140] -> w67
    tunnel: [w139] -> w66
    tunnel: w65 -> [w138]
    tunnel: [w137] -> w63
    tunnel: w64 -> [w136]
    tunnel: [w135] -> w62
    stop <- w133 stop-if-true
    # "Generate USER Event Loop"
    n40 = local read "Rising Edge"() -> (w130:bool)
    n41 = Or(x="OK Button", y=w130) -> (x .or. y?=w129:bool)
    n42 = local read "TASK ENABLE"() -> (w128:bool)
    n43 = And(x=w129, y=w128) -> (x .and. y?=w127:bool)
    n44 = case shown="True" w127 {
      selector: w127 -> [_ w153]
      tunnel: w142 -> [w152 w157]
      tunnel: [w152 w156] -> w139
      tunnel: w138 -> [w151 w155]
      tunnel: [w151 w154] -> w137
      frame False {
      }
      frame True {
        n45 = Generate User Event(user event=w157, event data cluster=w153, error in=w155) -> (user event out=w156:refnum<user-event>, error out=w154:errorcluster)  [unwired: 1 in]
      }
    }
    n46 = case shown="False" "STOP" {
      selector: "STOP" -> [_ w146]
      tunnel: w141 -> [w145 w150]
      tunnel: [w145 w149] -> w140
      tunnel: w136 -> [w144 w148]
      tunnel: [w144 w147] -> w135
      tunnel: [FALSE w146] -> w133
      frame False {
      }
      frame True {
        n47 = Generate User Event(user event=w150, event data cluster=w146, error in=w148) -> (user event out=w149:refnum<user-event>, error out=w147:errorcluster)  [unwired: 1 in]
      }
    }
    n48 = Wait (ms)(milliseconds to wait=u32 10) -> ()  [unwired: 1 out]
    n49 = call "FGV Bool.vi"("Init/Read/Write State"=States_for_Action_Engine."Write", "Input Node"=w133) -> ()  [unwired: 1 in, 2 out]
  }
  n50 = while {
    tunnel: w59 -> [w164]
    tunnel: [w163] -> w58
    tunnel: w46 -> [w161]
    tunnel: [w160] -> w57
    tunnel: w52 -> [w159]
    tunnel: [w158] -> w49
    stop <- w162 stop-if-true
    # "EVENT Handling Loop"
    n51 = event shown="[1] <Start Task>: User Event" {
      selector: w164 -> [_ _ _]
      dyn-events: [_ _ _] -> w163
      timeout: _ -> [_ _ _]
      tunnel: [FALSE FALSE w211] -> w162
      tunnel: w161 -> [w169 w178 w209]
      tunnel: [w168 w177 w210] -> w160
      tunnel: w159 -> [w167 w176 w208]
      tunnel: [w166 w175 w207] -> w158
      event Timeout {
        n52 = event-data() -> ()  [unwired: 1 in, 3 out]
        n53 = Enqueue Element(queue=w169, element=Intruction_Type_Definitions."Start Task 1" ("Enum"), error in (no error)=w167) -> (queue out=w168:refnum<queue>, error out=w166:errorcluster)  [unwired: 1 in, 1 out]
      }
      event User Event {
        n54 = event-data() -> ()  [unwired: 1 in, 5 out]
        n55 = call "Arduino Interfacing VI.vi"("AE Mode"=Arduino_Interfacing."Read From Arduino") -> ("Arduino Data"=w172:T17)  [unwired: 3 in, 1 out]
        n56 = Unbundle By Name(w172) -> ("Rotary Switch"=w171:u8)
        n57 = case shown="13" w171 {
          tunnel: [Intruction_Type_Definitions."Start Task 1" ("Enum") Intruction_Type_Definitions."Start Task 2" ("Enum") Intruction_Type_Definitions."Start Task 3" ("Enum") Intruction_Type_Definitions."Start Task 4" ("Enum") Intruction_Type_Definitions."Start Task 5" ("Enum") Intruction_Type_Definitions."Start Task 6" ("Enum") Intruction_Type_Definitions."Start Task 7" ("Enum") Intruction_Type_Definitions."Start Task 8 - BALL" ("Enum") Intruction_Type_Definitions."Start Task 8 - Soap" ("Enum") Intruction_Type_Definitions."Start Task 8 - Gel" ("Enum") Intruction_Type_Definitions."Start Task 8 - Pipe" ("Enum") Intruction_Type_Definitions."Start Task 9" ("Enum") Intruction_Type_Definitions."Start Task 9" ("Enum") Intruction_Type_Definitions."Start Task 9" ("Enum") Intruction_Type_Definitions."Start Task 9" ("Enum") Intruction_Type_Definitions."Start Task 9" ("Enum")] -> w174
          frame 0, Default {
          }
          frame 1 {
          }
          frame 2 {
          }
          frame 3 {
          }
          frame 4 {
          }
          frame 5 {
          }
          frame 6 {
          }
          frame 7 {
          }
          frame 8 {
          }
          frame 9 {
          }
          frame 10 {
          }
          frame 11 {
            # "Task 9: Red Detection"
            n58 = call "Box Colour FGV.vi"("Colour to detect"=Box_Colour_FGV_Colours."Red", "Init/R/W State"=Box_Colour_FGV_States."Write") -> ()  [unwired: 8 in, 2 out]
          }
          frame 12 {
            # "Task 9: Black Detection"
            n59 = call "Box Colour FGV.vi"("Colour to detect"=Box_Colour_FGV_Colours."Black", "Init/R/W State"=Box_Colour_FGV_States."Write") -> ()  [unwired: 8 in, 2 out]
          }
          frame 13 {
            # "Task 9: Blue Detection"
            n60 = call "Box Colour FGV.vi"("Colour to detect"=Box_Colour_FGV_Colours."Blue", "Init/R/W State"=Box_Colour_FGV_States."Write") -> ()  [unwired: 8 in, 2 out]
          }
          frame 14 {
            # "Task 9: Yellow Detection"
            n61 = call "Box Colour FGV.vi"("Colour to detect"=Box_Colour_FGV_Colours."Yellow", "Init/R/W State"=Box_Colour_FGV_States."Write") -> ()  [unwired: 8 in, 2 out]
          }
          frame 15 {
            # "Task 9: Green Detection"
            n62 = call "Box Colour FGV.vi"("Colour to detect"=Box_Colour_FGV_Colours."Green", "Init/R/W State"=Box_Colour_FGV_States."Write") -> ()  [unwired: 8 in, 2 out]
          }
        }
        "Selected Task" <- w174
        n63 = Enqueue Element(queue=w178, element=w174, error in (no error)=w176) -> (queue out=w177:refnum<queue>, error out=w175:errorcluster)  [unwired: 1 in, 1 out]
      }
      event User Event {
        n64 = event-data() -> ("Stop Queue"=w211:bool)  [unwired: 1 in, 4 out]
        n65 = Enqueue Element At Opposite End(queue=w209, element=Intruction_Type_Definitions."Exit" ("Enum"), error in (no error)=w208) -> (queue out=w210:refnum<queue>, error out=w207:errorcluster)  [unwired: 1 in, 1 out]
      }
    }
  }
  n66 = while {
    tunnel: w47 -> [w221]
    tunnel: w46 -> [w218]
    stop <- w215 stop-if-true
    # "Status Loop for Action Queues"
    n67 = Get Queue Status(queue=w221, return elements? (F)=TRUE) -> (error out=w217:errorcluster, # elements in queue=→"Action Queue Items":i32, elements=→"Action Queues items":string[])  [unwired: 1 in, 5 out]
    n68 = Get Queue Status(queue=w218, return elements? (F)=TRUE) -> (# pending remove=→"State Logic Queue Items":i32, error out=w216:errorcluster, elements=→"elements":T10[])  [unwired: 1 in, 5 out]
    n69 = Merge Errors(w217, w216) -> (w215:errorcluster)
    n70 = Wait (ms)(milliseconds to wait=u32 500) -> ()  [unwired: 1 out]
  }
  n71 = while {
    tunnel: w46 -> [w226]
    tunnel: w47 -> [w284]
    tunnel: w50 -> [w282]
    tunnel: [w281] -> _
    tunnel: [w280] -> w40
    shift-right: [w273] -> _
    shift-left: T9 {"PING_A"=0, "PING_B"=0, "PING_C"=0, "PING_D"=0} -> [w275]
    shift-right: [w267] -> _
    shift-left: State_Type_Definitions,_for_0.26g_versions_and_later_2."Startup" ("Enum") -> [w270]
    shift-right: [w263] -> _
    shift-left: T8 {"xDistance"=0.0, "yDistance"=0.0, "wDistance"=0.0} -> [w265]
    shift-right: [w260] -> _
    shift-left: _ -> [w259]
    shift-right: [w256] -> _
    shift-left: T11 {"Recognized Object"=FALSE, "Object X coordinate"=0.0, "Object Y coordinate"=0.0} -> [w258]
    shift-right: [w253] -> _
    shift-left: T7 {"y Stepper Position"=0, "z Stepper Position"=0} -> [w255]
    shift-right: [w250] -> _
    shift-left: T6 {"Yaw"=0.0, "Compass"=0.0} -> [w252]
    shift-right: [w247] -> _
    shift-left: T3 {"Time up flag"=FALSE, "SET TIME TO CHECK"=0.0} -> [w249]
    shift-right: [w245] -> _
    shift-left: T20 {"yStepper desired"=0} -> [w246]
    shift-right: [w241] -> _
    shift-left: T5 {"Left IR Sensor"=0.0, "Arm IR Sensor"=0.0, "Bottom IR Sensor"=0.0} -> [w243]
    shift-right: [w239] -> _
    shift-left: T19 {"ySpeed"=0.0, "xSpeed"=0.0, "wSpeed"=0.0} -> [w240]
    shift-right: [w236] -> _
    shift-left: T4 {"Line Detected?"=FALSE, "S1"=0.0, "S2"=0.0, "S3"=0.0, "S4"=0.0} -> [w238]
    shift-right: [w234] -> _
    shift-left: _ -> [w233]
    shift-right: [w225] -> _
    shift-left: T1 {"Red"=FALSE, "Black"=FALSE, "Blue"=FALSE, "Yellow"=FALSE, "Green"=FALSE, "Unknown"=FALSE, "Image processing done"=FALSE, "Colour"=enum."None"} -> [w228]
    stop <- w272 stop-if-true
    # ">>> Box Colour Detection >>>"
    # ">>State Logic Queue Reference >>"
    # ">>Action Queue>>"
    # ">>State Logic Queue Reference >>"
    # ">>> Line Sensor Cluster>>>"
    # ">>> IR Sensors >>>"
    # ">>> Time cluster >>>"
    # ">>> Object detection >>>"
    # ">>> Yaw >>>"
    # ">>> Ultrasonic Sensors Detect >>>"
    # ">>> Encoders >>>"
    # ">>> Stepper position >>>"
    # ">>State Logic  >>"
    # ">> Item Selection Bias >>"
    # ">> Item Selection Bias >>"
    # ">> Item Selection Bias >>"
    # ">>State Logic  >>"
    # ">>> Motor control cluster >>>"
    # ">>> yStepper command>>>"
    # ">>True Stop Next State >>"
    # ">>Error  >>"
    # ">>Timeout>>"
    # ">>Action states Queue Reference >>"
    # "TOP LEVEL BASELINE (MAIN PROCESSING LOOP)"
    n72 = Wait (ms)(milliseconds to wait=u32 20) -> ()  [unwired: 1 out]
    n73 = Dequeue Element(queue=w284, timeout in ms (-1)=0, error in (no error)=w282) -> (queue out=w276:refnum<queue>, element=w283:string, error out=w277:errorcluster)  [unwired: 1 out]
    "Action State" <- w283
    n74 = case shown="\"FORWARD\"" w283 {
      tunnel: [_ _ _ _ _ _ _ _ _ _ _ _ _ _ _ _ _ _ _ _ 0 w3331 _ _ _ _ _ _ _ _ _ _ _ _ _ _ _ _ _ _ _ _ _ _ _ _ _ _ _ _ _ _ _ _ _ _ _] -> w279
      tunnel: w276 -> [_ _ _ _ _ _ _ _ _ _ _ _ _ _ _ _ _ _ _ _ _ _ _ _ _ _ _ _ _ _ _ _ _ _ _ _ _ _ _ _ _ _ _ _ _ _ _ _ _ _ _ _ _ _ _ _ _]
      tunnel: w275 -> [w3003 w3015 w3030 w3044 w3064 w3079 w3093 w3107 w3123 w3138 w3152 w3162 w3180 w3197 w3212 w3227 w3251 w3261 w3292 w3305 w3319 w3332 w3344 w3357 w3377 w3412 w3449 w3463 w3474 w3486 w3499 w3514 w3530 w3542 w3554 w3574 w3597 w3608 w3624 w3655 w3665 w3678 w3691 w3704 w3714 w3732 w3742 w3761 w3770 w3786 w3802 w3818 w3834 w3850 w3864 w3879 w3899]
      tunnel: [w3003 w3015 w3030 w3044 w3064 w3079 w3093 w3107 w3123 w3138 w3152 w3162 w3180 w3198 w3212 w3227 w3251 w3261 w3293 w3305 w3319 w3332 w3344 w3357 w3377 w3411 w3448 w3463 w3474 w3486 w3499 w3514 w3530 w3542 w3554 w3574 w3597 w3608 w3624 w3655 w3665 w3678 w3691 w3704 w3714 w3732 w3742 w3761 w3770 w3786 w3802 w3818 w3834 w3850 w3864 w3879 w3899] -> w274
      tunnel: [TRUE TRUE _ _ _ _ _ _ _ _ _ _ _ _ _ _ _ _ _ _ _ _ _ _ _ _ _ _ _ _ _ _ _ _ _ _ _ _ _ _ _ _ _ _ _ _ _ _ _ _ _ _ _ _ _ _ _] -> w272
      tunnel: w270 -> [w3001 w3013 w3029 w3043 w3063 w3078 w3092 w3106 w3122 w3137 w3151 w3161 w3179 w3196 w3211 w3225 w3244 w3260 w3291 w3304 w3316 w3329 w3343 w3356 w3376 w3410 w3447 w3462 w3473 w3485 w3491 w3513 w3529 w3541 w3553 w3573 w3596 w3607 w3618 w3649 w3664 w3677 w3690 w3703 w3713 w3723 w3741 w3760 w3769 w3785 w3801 w3817 w3833 w3849 w3863 w3869 w3887]
      tunnel: [_ _ _ _ _ _ _ _ _ _ _ _ _ _ _ _ _ _ _ _ _ TRUE _ _ _ _ _ _ _ _ _ _ _ _ _ _ _ _ _ _ _ _ _ _ _ _ _ _ _ _ _ _ _ _ _ _ _] -> w269
      tunnel: [w3001 w3013 w3029 w3043 w3063 w3078 w3092 w3106 w3122 w3137 w3151 w3161 w3179 w3196 w3211 w3225 w3244 w3260 w3291 w3304 w3316 w3329 w3343 w3356 w3376 w3410 w3447 w3462 w3473 w3485 w3491 w3513 w3529 w3541 w3553 w3573 w3596 w3607 w3618 w3649 w3664 w3677 w3690 w3703 w3713 w3723 w3741 w3760 w3769 w3785 w3801 w3817 w3833 w3849 w3863 w3869 w3887] -> w268
      tunnel: w265 -> [w3000 w3012 w3028 w3046 w3062 w3077 w3091 w3105 w3121 w3136 w3150 w3163 w3178 w3195 w3213 w3229 w3246 w3262 w3290 w3306 w3315 w3328 w3345 w3358 w3372 w3401 w3437 w3461 w3476 w3487 w3496 w3515 w3531 w3543 w3555 w3575 w3598 w3610 w3622 w3653 w3667 w3680 w3693 w3706 w3716 w3727 w3744 w3763 w3772 w3788 w3804 w3820 w3836 w3852 w3866 w3871 w3892]
      tunnel: [w3000 w3012 w3028 w3046 w3062 w3077 w3091 w3105 w3121 w3136 w3150 w3163 w3177 w3195 w3213 w3229 w3246 w3262 w3289 w3306 w3315 w3328 w3345 w3358 w3372 w3400 w3436 w3461 w3476 w3487 w3496 w3515 w3531 w3543 w3555 w3575 w3598 w3610 w3622 w3653 w3667 w3680 w3693 w3706 w3716 w3727 w3744 w3763 w3772 w3788 w3804 w3820 w3836 w3852 w3866 w3871 w3892] -> w264
      tunnel: w258 -> [w2999 w3011 w3027 w3045 w3061 w3076 w3090 w3104 w3120 w3135 w3148 w3160 w3176 w3194 w3206 w3228 w3245 w3259 w3281 w3303 w3314 w3327 w3342 w3355 w3375 w3405 w3442 w3459 w3475 w3484 w3497 w3512 w3528 w3537 w3552 w3571 w3591 w3609 w3623 w3654 w3666 w3679 w3692 w3705 w3715 w3726 w3743 w3762 w3771 w3787 w3803 w3819 w3835 w3851 w3865 w3870 w3891]
      tunnel: [w2999 w3011 w3027 w3045 w3061 w3076 w3090 w3104 w3120 w3135 w3148 w3160 w3176 w3194 w3206 w3228 w3245 w3259 w3280 w3303 w3314 w3327 w3342 w3355 w3374 w3404 w3441 w3459 w3475 w3484 w3497 w3512 w3528 w3537 w3552 w3570 w3591 w3609 w3623 w3654 w3666 w3679 w3692 w3705 w3715 w3726 w3743 w3762 w3771 w3787 w3803 w3819 w3835 w3851 w3865 w3870 w3891] -> w257
      tunnel: w255 -> [w2998 w3010 w3026 w3047 w3060 w3075 w3089 w3103 w3119 w3134 w3147 w3159 w3175 w3193 w3214 w3230 w3247 w3258 w3286 w3302 w3313 w3326 w3341 w3354 w3371 w3396 w3432 w3458 w3472 w3483 w3495 w3511 w3527 w3540 w3551 w3576 w3599 w3611 w3621 w3652 w3663 w3676 w3689 w3702 w3717 w3728 w3745 w3759 w3773 w3789 w3805 w3821 w3837 w3853 w3867 w3872 w3893]
      tunnel: [w2998 w3010 w3026 w3047 w3060 w3075 w3089 w3103 w3119 w3134 w3147 w3159 w3175 w3193 w3214 w3230 w3247 w3258 w3285 w3302 w3313 w3326 w3341 w3354 w3371 w3395 w3431 w3458 w3472 w3483 w3495 w3511 w3527 w3540 w3551 w3576 w3599 w3611 w3621 w3652 w3663 w3676 w3689 w3702 w3717 w3728 w3745 w3758 w3773 w3789 w3805 w3821 w3837 w3853 w3867 w3872 w3893] -> w254
      tunnel: w252 -> [w2997 w3009 w3024 w3048 w3058 w3073 w3087 w3102 w3117 w3132 w3146 w3158 w3174 w3186 w3209 w3231 w3248 w3257 w3276 w3301 w3312 w3325 w3340 w3353 w3370 w3392 w3428 w3457 w3469 w3482 w3494 w3510 w3526 w3539 w3550 w3577 w3600 w3612 w3620 w3651 w3662 w3673 w3686 w3699 w3718 w3729 w3746 w3753 w3774 w3790 w3806 w3822 w3838 w3854 w3868 w3873 w3894]
      tunnel: [w2997 w3009 w3024 w3048 w3058 w3073 w3087 w3102 w3117 w3132 w3146 w3158 w3174 w3186 w3208 w3231 w3248 w3257 w3275 w3301 w3312 w3325 w3340 w3353 w3370 w3391 w3427 w3457 w3469 w3482 w3494 w3510 w3526 w3539 w3550 w3577 w3600 w3612 w3620 w3651 w3662 w3673 w3686 w3699 w3718 w3729 w3746 w3753 w3774 w3790 w3806 w3822 w3838 w3854 w3868 w3873 w3894] -> w251
      tunnel: w249 -> [w2995 w3008 w3025 w3049 w3059 w3074 w3088 w3101 w3118 w3133 w3145 w3157 w3173 w3185 w3205 w3232 w3249 w3256 w3272 w3298 w3311 w3324 w3339 w3352 w3369 w3389 w3425 w3455 w3468 w3481 w3493 w3509 w3525 w3538 w3549 w3578 w3601 w3613 w3619 w3650 w3661 w3672 w3685 w3698 w3719 w3730 w3747 w3752 w3768 w3784 w3800 w3816 w3832 w3848 w3862 w3874 w3895]
      tunnel: [w2995 w3008 w3025 w3049 w3059 w3074 w3088 w3101 w3118 w3133 w3145 w3157 w3173 w3185 w3205 w3232 w3249 w3256 w3272 w3298 w3311 w3324 w3339 w3352 w3368 w3388 w3424 w3455 w3468 w3481 w3493 w3509 w3525 w3538 w3549 w3578 w3601 w3613 w3619 w3650 w3661 w3672 w3685 w3698 w3719 w3730 w3747 w3752 w3768 w3782 w3798 w3814 w3830 w3847 w3861 w3874 w3895] -> w248
      tunnel: w246 -> [_ _ _ _ _ _ _ _ _ _ _ _ _ _ _ _ _ _ _ _ _ _ _ _ _ _ _ _ _ _ _ _ _ _ _ _ _ _ _ _ _ _ _ _ _ _ w3738 _ _ _ _ _ _ _ _ _ _]
      tunnel: [w2994 w3007 w3019 w3039 w3053 w3068 w3083 w3097 w3113 w3127 w3142 w3156 w3167 w3184 w3202 w3223 w3250 w3255 w3269 w3297 w3310 w3323 w3338 w3349 w3362 w3382 w3416 w3454 w3467 w3480 w3498 w3503 w3519 w3535 w3547 w3566 w3594 w3605 w3625 w3656 w3660 w3671 w3684 w3697 w3710 w3731 w3736 w3751 w3767 w3780 w3796 w3812 w3828 w3845 w3858 w3878 w3898] -> w242
      tunnel: w243 -> [w2994 w3007 w3019 w3039 w3053 w3068 w3083 w3097 w3113 w3127 w3142 w3156 w3167 w3184 w3202 w3224 w3250 w3255 w3269 w3297 w3310 w3323 w3338 w3349 w3362 w3383 w3417 w3454 w3467 w3480 w3498 w3503 w3519 w3535 w3547 w3566 w3594 w3605 w3625 w3656 w3660 w3671 w3684 w3697 w3710 w3731 w3736 w3751 w3767 w3780 w3796 w3812 w3828 w3845 w3858 w3878 w3898]
      tunnel: w240 -> [_ _ _ _ _ _ _ _ w3112 _ _ _ _ _ _ _ _ _ _ _ _ _ _ _ _ _ _ _ _ _ _ _ _ _ _ _ _ _ _ _ _ _ _ _ _ _ _ _ _ _ _ _ _ _ _ _ _]
      tunnel: w238 -> [w2993 w3006 w3018 w3033 w3052 w3067 w3082 w3096 w3110 w3126 w3141 w3155 w3166 w3183 w3201 w3219 w3243 w3254 w3267 w3296 w3309 w3322 w3337 w3348 w3365 w3385 w3420 w3453 w3466 w3479 w3490 w3502 w3518 w3534 w3546 w3564 w3593 w3604 w3616 w3648 w3659 w3670 w3683 w3696 w3709 w3722 w3735 w3750 w3766 w3779 w3795 w3811 w3827 w3844 w3857 w3877 w3897]
      tunnel: [w2993 w3006 w3018 w3033 w3052 w3067 w3082 w3096 w3110 w3126 w3141 w3155 w3166 w3183 w3201 w3219 w3242 w3254 w3267 w3296 w3309 w3322 w3337 w3348 w3364 w3384 w3419 w3453 w3466 w3479 w3490 w3502 w3518 w3534 w3546 w3564 w3593 w3604 w3616 w3648 w3659 w3670 w3683 w3696 w3709 w3722 w3735 w3750 w3766 w3779 w3795 w3811 w3827 w3844 w3857 w3877 w3897] -> w237
      tunnel: [_ _ _ _ _ _ _ _ _ _ _ _ _ _ _ _ _ _ _ _ _ _ _ _ _ _ _ _ _ _ _ _ _ _ _ w3558 w3588 _ _ _ _ _ _ _ _ _ _ _ _ _ _ _ _ _ _ _ _] -> w235
      tunnel: w233 -> [w2992 w3005 w3017 w3032 w3051 w3066 w3081 w3095 w3109 w3125 w3140 w3154 w3165 w3182 w3200 w3218 w3234 w3253 w3265 w3295 w3308 w3321 w3336 w3347 w3366 w3386 w3421 w3452 w3465 w3478 w3489 w3501 w3517 w3533 w3545 w3560 w3592 w3603 w3615 w3647 w3658 w3669 w3682 w3695 w3708 w3721 w3734 w3749 w3765 w3778 w3794 w3810 w3826 w3843 w3856 w3876 w3896]
      tunnel: [w2992 w3005 w3017 w3032 w3051 w3066 w3081 w3095 w3109 w3125 w3140 w3154 w3165 w3182 w3200 w3218 w3234 w3253 w3265 w3295 w3308 w3321 w3336 w3347 w3366 w3386 w3421 w3452 w3465 w3478 w3489 w3501 w3517 w3533 w3545 w3560 w3592 w3603 w3615 w3647 w3658 w3669 w3682 w3695 w3708 w3721 w3734 w3749 w3765 w3778 w3794 w3810 w3826 w3843 w3856 w3876 w3896] -> w232
      tunnel: w228 -> [w2991 w3004 w3016 w3031 w3050 w3065 w3080 w3094 w3108 w3124 w3139 w3153 w3164 w3181 w3199 w3215 w3233 w3252 w3264 w3294 w3307 w3320 w3335 w3346 w3361 w3379 w3415 w3451 w3464 w3477 w3488 w3500 w3516 w3532 w3544 w3563 w3586 w3602 w3614 w3646 w3657 w3668 w3681 w3694 w3707 w3720 w3733 w3748 w3764 w3777 w3793 w3809 w3825 w3842 w3855 w3875 w3890]
      tunnel: [w2991 w3004 w3016 w3031 w3050 w3065 w3080 w3094 w3108 w3124 w3139 w3153 w3164 w3181 w3199 w3215 w3233 w3252 w3264 w3294 w3307 w3320 w3335 w3346 w3360 w3379 w3415 w3451 w3464 w3477 w3488 w3500 w3516 w3532 w3544 w3563 w3579 w3602 w3614 w3645 w3657 w3668 w3681 w3694 w3707 w3720 w3733 w3748 w3764 w3777 w3793 w3809 w3825 w3842 w3855 w3875 w3889] -> w227
      frame "Exit" {
        # ">>State Logic  >>"
        # ">>> Time cluster >>>"
        # ">>> Yaw >>>"
        # ">>> Stepper position >>>"
        # ">>> Encoders >>>"
        # ">>> Object detection >>>"
        # ">>> Ultrasonic Sensors Detect >>>"
        n75 = call "Imaq Dispose"("All Images? (No)"=TRUE) -> ()  [unwired: 5 in, 1 out]
      }
      frame "----Movement States----" {
        # ">>State Logic  >>"
        # ">>> Time cluster >>>"
        # ">>> Yaw >>>"
        # ">>> Stepper position >>>"
        # ">>> Encoders >>>"
        # ">>> Object detection >>>"
        # ">>> Ultrasonic Sensors Detect >>>"
      }
      frame "FORWARD" {
        # "High voltage values: 30\nMid voltage values: 40\nLow voltage values: 50"
        # ">>State Logic  >>"
        # ">>> Time cluster >>>"
        # ">>> Yaw >>>"
        # ">>> Stepper position >>>"
        # ">>> Encoders >>>"
        # ">>> Object detection >>>"
        # ">>> Ultrasonic Sensors Detect >>>"
        n76 = Unbundle By Name(w3024) -> ("Yaw"=w3020:dbl)
        n77 = call "MOTOR CONTROL WITH PID AE.vi"("Yaw"=w3020, "Speed"=30.0, "Direction"=MOTOR_CONTROL_WITH_PID_AE_DIRECTION_TYPE_DEF."y-axis movement", "AE Mode"=MOTOR_CONTROL_WITH_PID_AE_DATA_MODE_TYPE_DEF."Write to AE") -> ()  [unwired: 1 out]
      }
      frame "FORWARD - IR ASSIST" {
        # "Algorithm sensitivity"
        # "Distance to maintain from wall"
        # ">>State Logic  >>"
        # ">>> Time cluster >>>"
        # ">>> Yaw >>>"
        # ">>> Stepper position >>>"
        # ">>> Encoders >>>"
        # ">>> Object detection >>>"
        # ">>> Ultrasonic Sensors Detect >>>"
        n78 = Unbundle By Name(w3039) -> ("Left IR Sensor"=w3038:dbl)
        n79 = Subtract(x=w3038, y=10.0) -> (x-y=w3036:dbl)
        n80 = Multiply(x=w3036, y=0.2) -> (x*y=w3034:dbl)
        n81 = call "MOTOR CONTROL WITH PID AE.vi"("Yaw"=w3034, "Speed"=35.0, "Direction"=MOTOR_CONTROL_WITH_PID_AE_DIRECTION_TYPE_DEF."y-axis movement", "AE Mode"=MOTOR_CONTROL_WITH_PID_AE_DATA_MODE_TYPE_DEF."Write to AE") -> ()  [unwired: 1 out]
      }
      frame "LEFT" {
        # ">>State Logic  >>"
        # ">>> Time cluster >>>"
        # ">>> Yaw >>>"
        # ">>> Stepper position >>>"
        # ">>> Encoders >>>"
        # ">>> Object detection >>>"
        # ">>> Ultrasonic Sensors Detect >>>"
        n82 = Unbundle By Name(w3058) -> ("Yaw"=w3055:dbl)
        n83 = call "MOTOR CONTROL WITH PID AE.vi"("Yaw"=w3055, "Speed"=-20.0, "Direction"=MOTOR_CONTROL_WITH_PID_AE_DIRECTION_TYPE_DEF."x-axis movement", "AE Mode"=MOTOR_CONTROL_WITH_PID_AE_DATA_MODE_TYPE_DEF."Write to AE") -> ()  [unwired: 1 out]
      }
      frame "RIGHT" {
        # ">>> Time cluster >>>"
        # ">>> Yaw >>>"
        # ">>> Stepper position >>>"
        # ">>> Encoders >>>"
        # ">>> Object detection >>>"
        # ">>> Ultrasonic Sensors Detect >>>"
        n84 = Unbundle By Name(w3073) -> ("Yaw"=w3069:dbl)
        n85 = call "MOTOR CONTROL WITH PID AE.vi"("Yaw"=w3069, "Speed"=30.0, "Direction"=MOTOR_CONTROL_WITH_PID_AE_DIRECTION_TYPE_DEF."x-axis movement", "AE Mode"=MOTOR_CONTROL_WITH_PID_AE_DATA_MODE_TYPE_DEF."Write to AE") -> ()  [unwired: 1 out]
      }
      frame "R-ACW" {
        # ">>> IR Sensors >>>"
        # ">>> Time cluster >>>"
        # ">>> Yaw >>>"
        # ">>> Stepper position >>>"
        # ">>> Encoders >>>"
        # ">>> Object detection >>>"
        # ">>> Ultrasonic Sensors Detect >>>"
        n86 = call "MOTOR CONTROL WITH PID AE.vi"("Speed"=10.0, "Direction"=MOTOR_CONTROL_WITH_PID_AE_DIRECTION_TYPE_DEF."rotation", "AE Mode"=MOTOR_CONTROL_WITH_PID_AE_DATA_MODE_TYPE_DEF."Write to AE") -> ()  [unwired: 1 in, 1 out]
      }
      frame "R-CW" {
        (unwired) -0.2 ("Speed")
        # ">>> Time cluster >>>"
        # ">>> Yaw >>>"
        # ">>> Stepper position >>>"
        # ">>> Encoders >>>"
        # ">>> Object detection >>>"
        # ">>> Ultrasonic Sensors Detect >>>"
        n87 = call "MOTOR CONTROL WITH PID AE.vi"("Speed"=-10.0, "Direction"=MOTOR_CONTROL_WITH_PID_AE_DIRECTION_TYPE_DEF."rotation", "AE Mode"=MOTOR_CONTROL_WITH_PID_AE_DATA_MODE_TYPE_DEF."Write to AE") -> ()  [unwired: 1 in, 1 out]
      }
      frame "X AXIS - SLOW" {
        # ">>> Line Sensor Cluster>>>"
        # ">>> IR Sensors >>>"
        # ">>> Time cluster >>>"
        # ">>> Yaw >>>"
        # ">>> Stepper position >>>"
        # ">>> Encoders >>>"
        # ">>> Object detection >>>"
        # ">>> Ultrasonic Sensors Detect >>>"
        n88 = Unbundle By Name(w3112) -> ("xSpeed"=w3111:dbl)
        n89 = Unbundle By Name(w3117) -> ("Yaw"=w3114:dbl)
        n90 = call "MOTOR CONTROL WITH PID AE.vi"("Yaw"=w3114, "Speed"=w3111, "Direction"=MOTOR_CONTROL_WITH_PID_AE_DIRECTION_TYPE_DEF."x-axis movement", "AE Mode"=MOTOR_CONTROL_WITH_PID_AE_DATA_MODE_TYPE_DEF."Write to AE") -> ()  [unwired: 1 out]
      }
      frame "REVERSE" {
        # ">>> Time cluster >>>"
        # ">>> Yaw >>>"
        # ">>> Stepper position >>>"
        # ">>> Encoders >>>"
        # ">>> Object detection >>>"
        # ">>> Ultrasonic Sensors Detect >>>"
        n91 = Unbundle By Name(w3132) -> ("Yaw"=w3128:dbl)
        n92 = call "MOTOR CONTROL WITH PID AE.vi"("Yaw"=w3128, "Speed"=-40.0, "Direction"=MOTOR_CONTROL_WITH_PID_AE_DIRECTION_TYPE_DEF."y-axis movement", "AE Mode"=MOTOR_CONTROL_WITH_PID_AE_DATA_MODE_TYPE_DEF."Write to AE") -> ()  [unwired: 1 out]
      }
      frame "STOP" {
        n93 = Wait (ms)(milliseconds to wait=u32 100) -> ()  [unwired: 1 out]
        n94 = call "MOTOR CONTROL WITH PID AE.vi"("Direction"=MOTOR_CONTROL_WITH_PID_AE_DIRECTION_TYPE_DEF."stop", "AE Mode"=MOTOR_CONTROL_WITH_PID_AE_DATA_MODE_TYPE_DEF."Write to AE") -> ()  [unwired: 2 in, 1 out]
      }
      frame "----SENSOR READING---- " {
      }
      frame "READ ENCODERS" {
        # ">>> Time cluster >>>"
        # ">>> Yaw >>>"
        # ">>> Stepper position >>>"
        # ">>> Object detection >>>"
        # ">>> Current encoder distance >>>"
        # ">>> Ultrasonic Sensors Detect >>>"
        n95 = call "MOTOR CONTROL WITH PID AE.vi"("AE Mode"=MOTOR_CONTROL_WITH_PID_AE_DATA_MODE_TYPE_DEF."Read from AE") -> ("Speed & distance"=w3171:T15)  [unwired: 3 in]
        n96 = Unbundle By Name(w3171) -> ("xDistance"=w3170:dbl, "yDistance"=w3169:dbl, "wDistance"=w3168:dbl)
        n97 = Bundle By Name(cluster=w3178, "xDistance"=w3170, "yDistance"=w3169, "wDistance"=w3168) -> (w3177:T8)
      }
      frame "READ ULTRASONIC" {
        (unwired) navX_type_def."Read Values" ("Mode")
        (unwired) MOTOR_CONTROL_NO_PID_Type_Def."Latch" ("Direction")
        # ">>> Line Sensor Cluster>>>"
        # ">>> IR Sensors >>>"
        # ">>State Logic  >>"
        # ">>> Time cluster >>>"
        # ">>> Ultrasonic Sensors Detect >>>"
        # ">>> Object detection >>>"
        # ">>> Encoders >>>"
        # ">>> Stepper position >>>"
        # ">>> Yaw >>>"
        n98 = call "Arduino Interfacing VI.vi"("AE Mode"=Arduino_Interfacing."Read From Arduino") -> ("Arduino Data"=w3191:T17)  [unwired: 3 in, 1 out]
        n99 = Unbundle By Name(w3191) -> ("PING A"=w3190:u8, "PING B"=w3189:u8, "PING C"=w3188:u8, "PING D"=w3187:u8)
        n100 = Bundle By Name(cluster=w3197, "PING_A"=w3190, "PING_B"=w3189, "PING_C"=w3188, "PING_D"=w3187) -> (w3198:T9)
      }
      frame "READ NAVX" {
        # ">> Item Selection Bias >>"
        # ">>State Logic  >>"
        # ">>> Line Sensor Cluster>>>"
        # ">>> IR Sensors >>>"
        # ">>> Time cluster >>>"
        # ">>> Yaw >>>"
        # ">>> Ultrasonic Sensors Detect >>>"
        # ">>> Object detection >>>"
        # ">>> Encoders >>>"
        # ">>> Stepper position >>>"
        n101 = call "navX reading VI.vi"("Mode"=navX_type_def."Read Values") -> ("NavX Readings"=w3204:T16)  [unwired: 2 in, 3 out]
        n102 = Unbundle By Name(w3204) -> ("Heading"=w3203:dbl)
        n103 = Unbundle By Name(w3204) -> ("Yaw"=w3207:dbl)
        n104 = Bundle By Name(cluster=w3209, "Yaw"=w3207, "Compass"=w3203) -> (w3208:T6)
      }
      frame "READ IR" {
        w3217 = T40 [enum."B/AI2"] items=["Not Connected", "AudioIn/Left", "AudioIn/Right", "C/AI0", "C/AI1", "A/AI0", "A/AI1", "A/AI2", "A/AI3", "A/AI4", "A/AI5", "A/AI6", "A/AI7", "B/AI0", "B/AI1", "B/AI2", "B/AI3", "B/AI4", "B/AI5", "B/AI6", "B/AI7", "AI/AI0", "AI/AI1", "AI/AI2", "AI/AI3", "A/AI0 (DIFF)", "A/AI1 (DIFF)", "A/AI2 (DIFF)", "A/AI3 (DIFF)", "B/AI0 (DIFF)", "B/AI1 (DIFF)", "B/AI2 (DIFF)", "B/AI3 (DIFF)"] ("AI Channel")
        w3221 = T40 [enum."B/AI1"] items=["Not Connected", "AudioIn/Left", "AudioIn/Right", "C/AI0", "C/AI1", "A/AI0", "A/AI1", "A/AI2", "A/AI3", "A/AI4", "A/AI5", "A/AI6", "A/AI7", "B/AI0", "B/AI1", "B/AI2", "B/AI3", "B/AI4", "B/AI5", "B/AI6", "B/AI7", "AI/AI0", "AI/AI1", "AI/AI2", "AI/AI3", "A/AI0 (DIFF)", "A/AI1 (DIFF)", "A/AI2 (DIFF)", "A/AI3 (DIFF)", "B/AI0 (DIFF)", "B/AI1 (DIFF)", "B/AI2 (DIFF)", "B/AI3 (DIFF)"] ("AI Channel")
        w3226 = T40 [enum."B/AI0"] items=["Not Connected", "AudioIn/Left", "AudioIn/Right", "C/AI0", "C/AI1", "A/AI0", "A/AI1", "A/AI2", "A/AI3", "A/AI4", "A/AI5", "A/AI6", "A/AI7", "B/AI0", "B/AI1", "B/AI2", "B/AI3", "B/AI4", "B/AI5", "B/AI6", "B/AI7", "AI/AI0", "AI/AI1", "AI/AI2", "AI/AI3", "A/AI0 (DIFF)", "A/AI1 (DIFF)", "A/AI2 (DIFF)", "A/AI3 (DIFF)", "B/AI0 (DIFF)", "B/AI1 (DIFF)", "B/AI2 (DIFF)", "B/AI3 (DIFF)"] ("AI Channel")
        # ">>> Line Sensor Cluster>>>"
        # ">>> IR Sensors >>>"
        # ">>State Logic  >>"
        # ">>> Time cluster >>>"
        # ">>> Ultrasonic Sensors Detect >>>"
        # ">>> Object detection >>>"
        # ">>> Encoders >>>"
        # ">>> Stepper position >>>"
        # ">>> Yaw >>>"
        n105 = call <vilib>:"Sharp IR.vi"("AI Channel"=w3226) -> ("Sharp IR Distance"=w3222:dbl)  [unwired: 8 in, 2 out]
        n106 = call <vilib>:"Sharp IR.vi"("AI Channel"=w3221) -> ("Sharp IR Distance"=w3220:dbl)  [unwired: 8 in, 2 out]
        n107 = call <vilib>:"Sharp IR.vi"("AI Channel"=w3217) -> ("Sharp IR Distance"=w3216:dbl)  [unwired: 8 in, 2 out]
        n108 = Bundle By Name(cluster=w3224, "Left IR Sensor"=w3222, "Arm IR Sensor"=w3220, "Bottom IR Sensor"=w3216) -> (w3223:T5)
      }
      frame "READ LINE SENSOR" {
        # ">>> IR Sensors >>>"
        # ">>> Line Sensor Cluster>>>"
        # ">>State Logic  >>"
        # ">>> Time cluster >>>"
        # ">>> Object detection >>>"
        # ">>> Yaw >>>"
        # ">>> Ultrasonic Sensors Detect >>>"
        # ">>> Encoders >>>"
        # ">>> Stepper position >>>"
        n109 = call "Line Sensor AE.vi"("AE State"=Line_Sensor_AE_Type_Def."READ FROM LINE SENSORS") -> ("Line Detected?"=w3240:bool, "Line Sensor Raw Values"=w3239:T42)
        n110 = Unbundle By Name(w3239) -> ("S1"=w3238:dbl, "S2"=w3237:dbl, "S3"=w3236:dbl, "S4"=w3235:dbl)
        n111 = Bundle By Name(cluster=w3243, "Line Detected?"=w3240, "S1"=w3238, "S2"=w3237, "S3"=w3236, "S4"=w3235) -> (w3242:T4)
      }
      frame "----SYSTEM MODES----" {
        (unwired) I2C_MASTER_Type_Def."Last State" ("Arduino Mode")
        # ">>> Object detection >>>"
        # ">>> Yaw >>>"
        # ">>> Ultrasonic Sensors Detect >>>"
        # ">>> Encoders >>>"
        # ">>> Stepper position >>>"
      }
      frame "INIT" {
        w3287 = u8 0
        w3288 = 0.0
        # ">>> IR Sensors >>>"
        # ">>> IR Sensors >>>"
        # ">>> Line Sensor Cluster>>>"
        # ">>> Time cluster >>>"
        # ">>> Object detection >>>"
        # ">>> Yaw >>>"
        # ">>> Ultrasonic Sensors Detect >>>"
        # ">>> Encoders >>>"
        # ">>> Stepper position >>>"
        # ">>State Logic  >>"
        n112 = call "Arduino Interfacing VI.vi"("AE Mode"=Arduino_Interfacing."Initialize") -> ()  [unwired: 3 in, 2 out]
        n113 = call "FGV Bool.vi"("Init/Read/Write State"=States_for_Action_Engine."Initialize") -> ()  [unwired: 2 in, 2 out]
        n114 = call "Elasped Timer.vi"("Action"=Elapsed_timer_control."Initialize") -> ()  [unwired: 7 in, 4 out]
        n115 = call "MOTOR CONTROL WITH PID AE.vi"("AE Mode"=MOTOR_CONTROL_WITH_PID_AE_DATA_MODE_TYPE_DEF."Init AE") -> ()  [unwired: 3 in, 1 out]
        n116 = call "IMAQ Reference AE.vi"("IMAQ AE States"=IMAQ_Reference_AE."Initialize AE") -> ()  [unwired: 1 in, 2 out]
        n117 = call "Line Sensor AE.vi"("AE State"=Line_Sensor_AE_Type_Def."INIT AE") -> ()  [unwired: 2 out]
        n118 = Bundle By Name(cluster=w3281, "Recognized Object"=FALSE, "Object X coordinate"=0.0, "Object Y coordinate"=0.0) -> (w3280:T11)
        n119 = Bundle By Name(cluster=w3286, "y Stepper Position"=u8 0, "z Stepper Position"=u8 0) -> (w3285:T7)
        n120 = Bundle By Name(cluster=w3290, "xDistance"=w3288, "yDistance"=w3288, "wDistance"=w3288) -> (w3289:T8)
        n121 = Bundle By Name(cluster=w3292, "PING_A"=w3287, "PING_B"=w3287, "PING_C"=w3287, "PING_D"=w3287) -> (w3293:T9)
        n122 = invoke class="VI" method="Default Vals.Reinit All"() -> ()  [unwired: 3 in, 3 out]
        n123 = Bundle By Name(cluster=w3276, "Yaw"=0.0) -> (w3275:T6)
        n124 = call "Box Colour FGV.vi"("Init/R/W State"=Box_Colour_FGV_States."Initialize") -> ()  [unwired: 9 in, 2 out]
      }
      frame "ARDUINO - ULTRASONIC" {
        # ">>> Time cluster >>>"
        # ">>> Line Sensor Cluster>>>"
        # ">>> Object detection >>>"
        # ">>> Yaw >>>"
        # ">>> Ultrasonic Sensors Detect >>>"
        # ">>> Encoders >>>"
        # ">>> Stepper position >>>"
        # ">>State Logic  >>"
        n125 = call "Arduino Interfacing VI.vi"("Data to Write"=I2C_MASTER_WRITE_NEW_Type_Def."Ultrasonic sensors", "AE Mode"=Arduino_Interfacing."Write to Arduino") -> ()  [unwired: 2 in, 2 out]
      }
      frame "NAVX CALIBRATE" {
        # ">>> Object detection >>>"
        # ">>> Yaw >>>"
        # ">>> Ultrasonic Sensors Detect >>>"
        # ">>> Encoders >>>"
        # ">>> Stepper position >>>"
        # ">>State Logic  >>"
        # "Adds a 15 second delay to the startup process \nfor the NavX to calibrate"
        n126 = Wait (ms)(milliseconds to wait=u32 1000) -> ()  [unwired: 1 out]
      }
      frame "NO ACTION", Default {
        (unwired) u8 0 ("y Stepper value")
        (unwired) TRUE ("Latch")
        (unwired) navX_type_def."Read Values" ("Mode")
        (unwired) MOTOR_CONTROL_NO_PID_Type_Def."Latch" ("Direction")
        # ">>> Object detection >>>"
        # ">>> Yaw >>>"
        # ">>> Ultrasonic Sensors Detect >>>"
        # ">>> Encoders >>>"
        # ">>> Stepper position >>>"
        # ">>State Logic  >>"
        n127 = case shown="\"Idle\"" w3329 {
          tunnel: [0 100] -> w3331
          frame "Startup", Default {
          }
          frame "Idle" {
          }
        }
      }
      frame "----RESET CASES----" {
        (unwired) I2C_MASTER_Type_Def."Last State" ("Arduino Mode")
        # ">>> Object detection >>>"
        # ">>> Yaw >>>"
        # ">>> Ultrasonic Sensors Detect >>>"
        # ">>> Encoders >>>"
        # ">>> Stepper position >>>"
        # ">>State Logic  >>"
      }
      frame "RESET ENCODERS" {
        # ">>> Object detection >>>"
        # ">>> Yaw >>>"
        # ">>> Ultrasonic Sensors Detect >>>"
        # ">>> Encoders >>>"
        # ">>> Stepper position >>>"
        # ">>State Logic  >>"
        n128 = call "MOTOR CONTROL WITH PID AE.vi"("Direction"=MOTOR_CONTROL_WITH_PID_AE_DIRECTION_TYPE_DEF."reset encoders", "AE Mode"=MOTOR_CONTROL_WITH_PID_AE_DATA_MODE_TYPE_DEF."Write to AE") -> ()  [unwired: 2 in, 1 out]
      }
      frame "RESET FLAGS" {
        w3359 = FALSE ("Line Detected?")
        # ">>> Line Sensor Cluster>>>"
        # ">>> IR Sensors >>>"
        # ">>> Time cluster >>>"
        # ">>> Object detection >>>"
        # ">>> Yaw >>>"
        # ">>> Ultrasonic Sensors Detect >>>"
        # ">>> Encoders >>>"
        # ">>> Stepper position >>>"
        # ">>> Line Sensor Cluster>>>"
        # ">>> IR Sensors >>>"
        # ">>> Time cluster >>>"
        # ">>> Object detection >>>"
        # ">>> Yaw >>>"
        # ">>> Ultrasonic Sensors Detect >>>"
        # ">>> Encoders >>>"
        # ">>> Stepper position >>>"
        # "Resets BOOLEAN FLAGS only"
        n129 = Wait (ms)(milliseconds to wait=u32 20) -> ()  [unwired: 1 out]
        n130 = Bundle By Name(cluster=w3375, "Recognized Object"=FALSE) -> (w3374:T11)
        n131 = Bundle By Name(cluster=w3365, "Line Detected?"=FALSE) -> (w3364:T4)
        n132 = Bundle By Name(cluster=w3369, "Time up flag"=FALSE) -> (w3368:T3)
        n133 = Bundle By Name(cluster=w3361, "Red"=w3359, "Black"=w3359, "Blue"=w3359, "Yellow"=w3359, "Green"=w3359, "Unknown"=w3359, "Image processing done"=w3359) -> (w3360:T1)
      }
      frame "RESET SENSOR VALUES" {
        w3380 = 0.0 ("S4")
        w3381 = 0.0 ("S4")
        # "Resets SENSOR VALUES only"
        # ">>> Line Sensor Cluster>>>"
        # ">>> IR Sensors >>>"
        # ">>> Time cluster >>>"
        # ">>> Object detection >>>"
        # ">>> Yaw >>>"
        # ">>> Ultrasonic Sensors Detect >>>"
        # ">>> Encoders >>>"
        # ">>> Stepper position >>>"
        # ">>> Line Sensor Cluster>>>"
        # ">>> IR Sensors >>>"
        # ">>> Time cluster >>>"
        # ">>> Object detection >>>"
        # ">>> Yaw >>>"
        # ">>> Ultrasonic Sensors Detect >>>"
        # ">>> Encoders >>>"
        # ">>> Stepper position >>>"
        # "Resets any software variables\nand/or non-critical states"
        n134 = Wait (ms)(milliseconds to wait=u32 20) -> ()  [unwired: 1 out]
        n135 = Bundle By Name(cluster=w3389, "SET TIME TO CHECK"=0.0) -> (w3388:T3)
        n136 = Bundle By Name(cluster=w3405, "Object X coordinate"=0.0, "Object Y coordinate"=0.0) -> (w3404:T11)
        n137 = Bundle By Name(cluster=w3396, "y Stepper Position"=u8 0, "z Stepper Position"=u8 0) -> (w3395:T7)
        n138 = Bundle By Name(cluster=w3383, "Left IR Sensor"=w3380, "Arm IR Sensor"=w3380) -> (w3382:T5)
        n139 = Bundle By Name(cluster=w3401, "xDistance"=0.0, "yDistance"=0.0, "wDistance"=0.0) -> (w3400:T8)
        n140 = Bundle By Name(cluster=w3412, "PING_A"=u8 0, "PING_B"=u8 0, "PING_C"=u8 0, "PING_D"=u8 0) -> (w3411:T9)
        n141 = Bundle By Name(cluster=w3392, "Yaw"=0.0) -> (w3391:T6)
        n142 = Bundle By Name(cluster=w3385, "S1"=w3381, "S2"=w3381, "S3"=w3381, "S4"=w3381) -> (w3384:T4)
      }
      frame "RESET ALL SENSORS" {
        w3414 = 0.0 ("SET TIME TO CHECK")
        # ">>> Line Sensor Cluster>>>"
        # ">>> IR Sensors >>>"
        # ">>> Time cluster >>>"
        # ">>> Object detection >>>"
        # ">>> Yaw >>>"
        # ">>> Ultrasonic Sensors Detect >>>"
        # ">>> Encoders >>>"
        # ">>> Stepper position >>>"
        # ">>> Line Sensor Cluster>>>"
        # ">>> IR Sensors >>>"
        # ">>> Time cluster >>>"
        # ">>> Object detection >>>"
        # ">>> Yaw >>>"
        # ">>> Ultrasonic Sensors Detect >>>"
        # ">>> Encoders >>>"
        # ">>> Stepper position >>>"
        # "Resets ALL SENSOR PARAMTERS"
        n143 = Wait (ms)(milliseconds to wait=u32 20) -> ()  [unwired: 1 out]
        n144 = Bundle By Name(cluster=w3425, "Time up flag"=FALSE, "SET TIME TO CHECK"=0.0) -> (w3424:T3)
        n145 = Bundle By Name(cluster=w3442, "Recognized Object"=FALSE, "Object X coordinate"=0.0, "Object Y coordinate"=0.0) -> (w3441:T11)
        n146 = Bundle By Name(cluster=w3432, "y Stepper Position"=u8 0, "z Stepper Position"=u8 0) -> (w3431:T7)
        n147 = Bundle By Name(cluster=w3417, "Left IR Sensor"=w3414, "Arm IR Sensor"=w3414, "Bottom IR Sensor"=w3414) -> (w3416:T5)
        n148 = Bundle By Name(cluster=w3420, "Line Detected?"=FALSE) -> (w3419:T4)
        n149 = Bundle By Name(cluster=w3437, "xDistance"=0.0, "yDistance"=0.0, "wDistance"=0.0) -> (w3436:T8)
        n150 = Bundle By Name(cluster=w3449, "PING_A"=u8 0, "PING_B"=u8 0, "PING_C"=u8 0, "PING_D"=u8 0) -> (w3448:T9)
        n151 = Bundle By Name(cluster=w3428, "Yaw"=0.0) -> (w3427:T6)
      }
      frame "RESET YAW" {
        n152 = Wait (ms)(milliseconds to wait=u32 100) -> ()  [unwired: 1 out]
        n153 = call "navX reading VI.vi"("Mode"=navX_type_def."Zero Yaw") -> ()  [unwired: 2 in, 4 out]
      }
      frame "RESET ARM" {
        n154 = call "Arduino Interfacing VI.vi"("Data to Write"=I2C_MASTER_WRITE_NEW_Type_Def."Soft Reset", "AE Mode"=Arduino_Interfacing."Write to Arduino") -> ()  [unwired: 2 in, 2 out]
      }
      frame "--------CAM STATES-------" {
      }
      frame "OPEN IMAQ REF" {
        # ">>> Line Sensor Cluster>>>"
        # ">>State Logic  >>"
        # ">>> Time cluster >>>"
        # ">>> Object detection >>>"
        # ">>> Yaw >>>"
        # ">>> Ultrasonic Sensors Detect >>>"
        # ">>> Encoders >>>"
        # ">>> Stepper position >>>"
        # ">>> IR Sensors >>>"
        n155 = call "IMAQ Reference AE.vi"("IMAQ AE States"=IMAQ_Reference_AE."Initialize AE") -> ()  [unwired: 1 in, 2 out]
      }
      frame "OPEN LOG CAM" {
        n156 = call "Webcam AE.vi"("Session In"=T38 "cam0", "Camera states"=Webcam_AE."Initialize Camera") -> ("error out"=w3506:errorcluster, "Session Out"=w3505:T38)  [unwired: 1 in, 1 out]
        n157 = call "Webcam AE.vi"("error in (no error)"=w3506, "Session In"=w3505, "Camera states"=Webcam_AE."Open Camera") -> ()  [unwired: 3 out]
      }
      frame "OPEN LIFE CAM" {
        n158 = call "Webcam AE.vi"("Session In"=T38 "cam1", "Camera states"=Webcam_AE."Initialize Camera") -> ("error out"=w3522:errorcluster, "Session Out"=w3521:T38)  [unwired: 1 in, 1 out]
        n159 = call "Webcam AE.vi"("error in (no error)"=w3522, "Session In"=w3521, "Camera states"=Webcam_AE."Open Camera") -> ()  [unwired: 3 out]
      }
      frame "CAM ACQ" {
        # ">>State Logic  >>"
        # ">>> Time cluster >>>"
        # ">>> Yaw >>>"
        # ">>> Stepper position >>>"
        # ">>> Encoders >>>"
        # ">>> Object detection >>>"
        # ">>> Ultrasonic Sensors Detect >>>"
        n160 = call "Webcam AE.vi"("Camera states"=Webcam_AE."Continuous Acquisition") -> ()  [unwired: 2 in, 3 out]
      }
      frame "CAM CLOSE" {
        # ">>> Box Colour Detection >>>"
        # ">>> Line Sensor Cluster>>>"
        # ">>> IR Sensors >>>"
        # ">>State Logic  >>"
        # ">>> Time cluster >>>"
        # ">>> Yaw >>>"
        # ">>> Stepper position >>>"
        # ">>> Encoders >>>"
        # ">>> Object detection >>>"
        # ">>> Ultrasonic Sensors Detect >>>"
        n161 = call "Webcam AE.vi"("Camera states"=Webcam_AE."Close Camera") -> ()  [unwired: 2 in, 3 out]
      }
      frame "PROCESS IMAGE" {
        # ">>> Line Sensor Cluster>>>"
        # ">>> IR Sensors >>>"
        # ">> Item Selection Bias >>"
        # ">> Item Selection Bias >>"
        # ">>State Logic  >>"
        # ">>> Time cluster >>>"
        # ">>> Yaw >>>"
        # ">>> Stepper position >>>"
        # ">>> Encoders >>>"
        # ">>> Object detection >>>"
        # ">>> Ultrasonic Sensors Detect >>>"
        n162 = call "Webcam AE.vi"("Camera states"=Webcam_AE."Retrieve Image") -> ("error out"=w3559:errorcluster, "Image Out"=w3562:T44)  [unwired: 2 in, 1 out]
        n163 = call "IMAQ Reference AE.vi"("IMAQ AE States"=IMAQ_Reference_AE."Get IMAQ Reference") -> ("Image Out"=w3561:T44)  [unwired: 1 in, 1 out]
        n164 = call "Object Detection SubVI experimental.vi"("Error In"=w3559, "Mode"=w3560, "Image Dest"=w3561, "Image in"=w3562) -> ("Error out"=w3558:errorcluster, "Object Center Coordinates"=w3557:cluster{"x":sgl, "y":sgl}, "Object detection cluster"=w3556:T45)  [unwired: 1 out]
        n165 = Unbundle By Name(w3556) -> ("Object detected?"=w3567:bool)
        n166 = Unbundle By Name(w3557) -> ("x"=w3569:sgl, "y"=w3568:sgl)
        n167 = Bundle By Name(cluster=w3571, "Recognized Object"=w3567, "Object X coordinate"=w3569, "Object Y coordinate"=w3568) -> (w3570:T11)
      }
      frame "COLOUR PROCESSING" {
        # ">>> Box Colour Detection >>>"
        # ">>> Box Colour Detection >>>"
        # ">>> Line Sensor Cluster>>>"
        # ">>> IR Sensors >>>"
        # ">> Item Selection Bias >>"
        # ">> Item Selection Bias >>"
        # ">>State Logic  >>"
        # ">>> Time cluster >>>"
        # ">>> Yaw >>>"
        # ">>> Stepper position >>>"
        # ">>> Encoders >>>"
        # ">>> Object detection >>>"
        # ">>> Ultrasonic Sensors Detect >>>"
        n168 = call "Webcam AE.vi"("Camera states"=Webcam_AE."Retrieve Image") -> ("error out"=w3589:errorcluster, "Image Out"=w3590:T44)  [unwired: 2 in, 1 out]
        n169 = call "Box Colour Detection SubVI.vi"("Image In"=w3590, "Error In"=w3589) -> ("Colour output boolean cluster"=w3587:T46, "Error out"=w3588:errorcluster)  [unwired: 1 out]
        n170 = Unbundle By Name(w3587) -> ("Red"=w3585:bool, "Black"=w3584:bool, "Blue"=w3583:bool, "Yellow"=w3582:bool, "Green"=w3581:bool, "No recognizable coolour"=w3580:bool)
        n171 = Bundle By Name(cluster=w3586, "Red"=w3585, "Black"=w3584, "Blue"=w3583, "Yellow"=w3582, "Green"=w3581, "Unknown"=w3580) -> (w3579:T1)
      }
      frame "DISPOSE CAM BUFFERS" {
        # ">> Item Selection Bias >>"
        # ">>> Line Sensor Cluster>>>"
        # ">>> IR Sensors >>>"
        # ">>State Logic  >>"
        # ">>> Time cluster >>>"
        # ">>> Yaw >>>"
        # ">>> Stepper position >>>"
        # ">>> Encoders >>>"
        # ">>> Object detection >>>"
        # ">>> Ultrasonic Sensors Detect >>>"
        n172 = call "Webcam AE.vi"("Camera states"=Webcam_AE."Dispose Camera Image Buffer") -> ()  [unwired: 2 in, 3 out]
      }
      frame "DISPOSE PROC BUFFERS" {
        # ">>> Box Colour Detection >>>"
        # ">>> Line Sensor Cluster>>>"
        # ">>State Logic  >>"
        # ">>> IR Sensors >>>"
        # ">>> Time cluster >>>"
        # ">>> Object detection >>>"
        # ">>> Yaw >>>"
        # ">>> Ultrasonic Sensors Detect >>>"
        # ">>> Encoders >>>"
        # ">>> Stepper position >>>"
        n173 = call "IMAQ Reference AE.vi"("IMAQ AE States"=IMAQ_Reference_AE."Dispose Processing Buffer") -> ()  [unwired: 1 in, 2 out]
      }
      frame "BOX COLOUR" {
        # ">>> Box Colour Detection >>>"
        # ">>> Line Sensor Cluster>>>"
        # ">>State Logic  >>"
        # ">>> IR Sensors >>>"
        # ">>> Time cluster >>>"
        # ">>> Object detection >>>"
        # ">>> Yaw >>>"
        # ">>> Ultrasonic Sensors Detect >>>"
        # ">>> Encoders >>>"
        # ">>> Stepper position >>>"
        n174 = call "Box Colour Detection Sequence.vi"() -> ("Colour scan time out?"=w3642:bool, "Colour output boolean cluster"=w3644:T46)  [unwired: 9 in, 1 out]
        n175 = Unbundle By Name(w3644) -> ("Red"=w3641:bool, "Black"=w3637:bool, "Blue"=w3634:bool, "Yellow"=w3633:bool, "Green"=w3630:bool, "No recognizable coolour"=w3643:bool)
        n176 = Select(t=Box_Colour_FGV_Colours."Green" ("Colour"), s=w3630, f=Box_Colour_FGV_Colours."None" ("Colour")) -> (s? t:f=w3628:T2)
        n177 = Select(t=Box_Colour_FGV_Colours."Yellow" ("Colour"), s=w3633, f=w3628) -> (s? t:f=w3627:T2)
        n178 = Select(t=Box_Colour_FGV_Colours."Blue" ("Colour"), s=w3634, f=w3627) -> (s? t:f=w3636:T2)
        n179 = Select(t=Box_Colour_FGV_Colours."Black" ("Colour"), s=w3637, f=w3636) -> (s? t:f=w3639:T2)
        n180 = Select(t=Box_Colour_FGV_Colours."Red" ("Colour"), s=w3641, f=w3639) -> (s? t:f=w3626:T2)
        n181 = Bundle By Name(cluster=w3646, "Red"=w3641, "Black"=w3637, "Blue"=w3634, "Yellow"=w3633, "Green"=w3630, "Unknown"=w3643, "Image processing done"=w3642, "Colour"=w3626) -> (w3645:T1)
      }
      frame "-----ARM ACTIONS-----" {
      }
      frame "CLOSE CLAW" {
        n182 = call "Arduino Interfacing VI.vi"("Data to Write"=I2C_MASTER_WRITE_NEW_Type_Def."Close Claw", "AE Mode"=Arduino_Interfacing."Write to Arduino") -> ()  [unwired: 2 in, 2 out]
      }
      frame "OPEN CLAW" {
        n183 = call "Arduino Interfacing VI.vi"("Data to Write"=I2C_MASTER_WRITE_NEW_Type_Def."Open Claw", "AE Mode"=Arduino_Interfacing."Write to Arduino") -> ()  [unwired: 2 in, 2 out]
      }
      frame "Z STEPPER CAM HEIGHT" {
        n184 = call "Arduino Interfacing VI.vi"("Data to Write"=I2C_MASTER_WRITE_NEW_Type_Def."zStepper 6k", "AE Mode"=Arduino_Interfacing."Write to Arduino") -> ()  [unwired: 2 in, 2 out]
      }
      frame "Z STEPPER GRAB HEIGHT" {
        # ">>State Logic  >>"
        # ">>> Time cluster >>>"
        # ">>> Yaw >>>"
        # ">>> Stepper position >>>"
        # ">>> Encoders >>>"
        # ">>> Object detection >>>"
        # ">>> Ultrasonic Sensors Detect >>>"
        n185 = call "Arduino Interfacing VI.vi"("Data to Write"=I2C_MASTER_WRITE_NEW_Type_Def."zStepper 100", "AE Mode"=Arduino_Interfacing."Write to Arduino") -> ()  [unwired: 2 in, 2 out]
      }
      frame "Z STEPPER BOX HEIGHT" {
        # ">>> IR Sensors >>>"
        # ">>> Time cluster >>>"
        # ">>> Yaw >>>"
        # ">>> Stepper position >>>"
        # ">>> Encoders >>>"
        # ">>> Object detection >>>"
        # ">>> Ultrasonic Sensors Detect >>>"
        n186 = call "Arduino Interfacing VI.vi"("Data to Write"=I2C_MASTER_WRITE_NEW_Type_Def."zStepper 5k", "AE Mode"=Arduino_Interfacing."Write to Arduino") -> ()  [unwired: 2 in, 2 out]
      }
      frame "Y STEPPER CONTROL" {
        # ">>State Logic  >>"
        # ">>> yStepper command>>>"
        # ">>> Time cluster >>>"
        # ">>> Yaw >>>"
        # ">>> Stepper position >>>"
        # ">>> Encoders >>>"
        # ">>> Object detection >>>"
        # ">>> Ultrasonic Sensors Detect >>>"
        n187 = Unbundle By Name(w3738) -> ("yStepper desired"=w3737:u8)
        n188 = call "Arduino Interfacing VI.vi"("y Stepper value"=w3737, "Data to Write"=I2C_MASTER_WRITE_NEW_Type_Def."yStepper control", "AE Mode"=Arduino_Interfacing."Write to Arduino") -> ()  [unwired: 1 in, 2 out]
      }
      frame "READ STEPPER VALUES" {
        # ">>State Logic  >>"
        # ">>> Time cluster >>>"
        # ">>> Yaw >>>"
        # ">>> Stepper position >>>"
        # ">>> Encoders >>>"
        # ">>> Object detection >>>"
        # ">>> Ultrasonic Sensors Detect >>>"
        n189 = call "Arduino Interfacing VI.vi"("AE Mode"=Arduino_Interfacing."Read From Arduino") -> ("Arduino Data"=w3756:T17)  [unwired: 3 in, 1 out]
        n190 = Unbundle By Name(w3756) -> ("y Stepper Position"=w3755:u8, "z Stepper Position"=w3754:u8)
        n191 = Bundle By Name(cluster=w3759, "y Stepper Position"=w3755, "z Stepper Position"=w3754) -> (w3758:T7)
      }
      frame " -----TIMING-----" {
        # ">>State Logic  >>"
        # ">>> Time cluster >>>"
        # ">>> Yaw >>>"
        # ">>> Stepper position >>>"
        # ">>> Encoders >>>"
        # ">>> Object detection >>>"
        # ">>> Ultrasonic Sensors Detect >>>"
      }
      frame "SET TIMER 1" {
        w3775 = 1.0 ("Time Setting")
        # ">>State Logic  >>"
        # ">>> Time cluster >>>"
        # ">>> Yaw >>>"
        # ">>> Stepper position >>>"
        # ">>> Encoders >>>"
        # ">>> Object detection >>>"
        # ">>> Ultrasonic Sensors Detect >>>"
        n192 = Wait (ms)(milliseconds to wait=u32 250) -> ()  [unwired: 1 out]
        n193 = call "Elasped Timer.vi"("Time Setting"=w3775, "Action"=Elapsed_timer_control."Initialize") -> ()  [unwired: 6 in, 4 out]
        n194 = Bundle By Name(cluster=w3784, "Time up flag"=FALSE, "SET TIME TO CHECK"=w3775) -> (w3782:T3)
      }
      frame "SET TIMER 2" {
        w3791 = 2.0 ("Time Setting")
        # ">>State Logic  >>"
        # ">>> Time cluster >>>"
        # ">>> Yaw >>>"
        # ">>> Stepper position >>>"
        # ">>> Encoders >>>"
        # ">>> Object detection >>>"
        # ">>> Ultrasonic Sensors Detect >>>"
        n195 = Wait (ms)(milliseconds to wait=u32 250) -> ()  [unwired: 1 out]
        n196 = call "Elasped Timer.vi"("Time Setting"=w3791, "Action"=Elapsed_timer_control."Initialize") -> ()  [unwired: 6 in, 4 out]
        n197 = Bundle By Name(cluster=w3800, "Time up flag"=FALSE, "SET TIME TO CHECK"=w3791) -> (w3798:T3)
      }
      frame "SET TIMER 3" {
        w3807 = 3.0 ("Time Setting")
        # ">>State Logic  >>"
        # ">>> Time cluster >>>"
        # ">>> Yaw >>>"
        # ">>> Stepper position >>>"
        # ">>> Encoders >>>"
        # ">>> Object detection >>>"
        # ">>> Ultrasonic Sensors Detect >>>"
        n198 = Wait (ms)(milliseconds to wait=u32 250) -> ()  [unwired: 1 out]
        n199 = call "Elasped Timer.vi"("Time Setting"=w3807, "Action"=Elapsed_timer_control."Initialize") -> ()  [unwired: 6 in, 4 out]
        n200 = Bundle By Name(cluster=w3816, "Time up flag"=FALSE, "SET TIME TO CHECK"=w3807) -> (w3814:T3)
      }
      frame "SET TIMER 4" {
        w3823 = 4.0 ("Time Setting")
        # ">>State Logic  >>"
        # ">>> Time cluster >>>"
        # ">>> Yaw >>>"
        # ">>> Stepper position >>>"
        # ">>> Encoders >>>"
        # ">>> Object detection >>>"
        # ">>> Ultrasonic Sensors Detect >>>"
        n201 = call "Elasped Timer.vi"("Time Setting"=w3823, "Action"=Elapsed_timer_control."Initialize") -> ()  [unwired: 6 in, 4 out]
        n202 = Wait (ms)(milliseconds to wait=u32 250) -> ()  [unwired: 1 out]
        n203 = Bundle By Name(cluster=w3832, "Time up flag"=FALSE, "SET TIME TO CHECK"=w3823) -> (w3830:T3)
      }
      frame "SET TIMER 5" {
        w3840 = 5.0 ("Time Setting")
        # ">>State Logic  >>"
        # ">>> Time cluster >>>"
        # ">>> Yaw >>>"
        # ">>> Stepper position >>>"
        # ">>> Encoders >>>"
        # ">>> Object detection >>>"
        # ">>> Ultrasonic Sensors Detect >>>"
        n204 = call "Elasped Timer.vi"("Time Setting"=w3840, "Action"=Elapsed_timer_control."Initialize") -> ("Time Out?!"=w3839:bool)  [unwired: 6 in, 3 out]
        n205 = Wait (ms)(milliseconds to wait=u32 250) -> ()  [unwired: 1 out]
        n206 = Bundle By Name(cluster=w3848, "Time up flag"=w3839, "SET TIME TO CHECK"=w3840) -> (w3847:T3)
      }
      frame "START TIMER" {
        # ">>State Logic  >>"
        # ">>> Time cluster >>>"
        # ">>> Yaw >>>"
        # ">>> Stepper position >>>"
        # ">>> Encoders >>>"
        # ">>> Object detection >>>"
        # ">>> Ultrasonic Sensors Detect >>>"
        n207 = call "Elasped Timer.vi"("Action"=Elapsed_timer_control."Start") -> ("Time Out?!"=w3859:bool)  [unwired: 7 in, 3 out]
        n208 = Bundle By Name(cluster=w3862, "Time up flag"=w3859) -> (w3861:T3)
      }
      frame "-----MISC-----" {
        # ">>> Box Colour Detection >>>"
        # ">>> Line Sensor Cluster>>>"
        # ">>> IR Sensors >>>"
        # ">>> Time cluster >>>"
        # ">>> Object detection >>>"
        # ">>> Yaw >>>"
        # ">>> Ultrasonic Sensors Detect >>>"
        # ">>> Encoders >>>"
        # ">>> Stepper position >>>"
      }
      frame "Task 9" {
        # ">>> Box Colour Detection >>>"
        # ">>> Line Sensor Cluster>>>"
        # ">>> IR Sensors >>>"
        # ">>> Time cluster >>>"
        # ">>> Object detection >>>"
        # ">>> Yaw >>>"
        # ">>> Ultrasonic Sensors Detect >>>"
        # ">>> Encoders >>>"
        # ">>> Stepper position >>>"
        n209 = call "Colour Processing Test Env.vi"() -> ("Colour scan time out?"=w3888:bool, "Colour output boolean cluster"=w3886:T46)  [unwired: 10 in]
        n210 = Unbundle By Name(w3886) -> ("Red"=w3880:bool, "Black"=w3881:bool, "Blue"=w3882:bool, "Yellow"=w3883:bool, "Green"=w3884:bool, "No recognizable coolour"=w3885:bool)
        n211 = Bundle By Name(cluster=w3890, "Red"=w3880, "Black"=w3881, "Blue"=w3882, "Yellow"=w3883, "Green"=w3884, "Unknown"=w3885, "Image processing done"=w3888) -> (w3889:T1)
      }
    }
    "State Logic" <- w268
    "Image Processing Error" <- w235
    n212 = local read "TASK ENABLE"() -> (w262:bool)
    n213 = Not(x=w262) -> (.not. x?=w261:bool)
    n214 = case shown="True" w269 {
      tunnel: w226 -> [w300 w354]
      tunnel: w276 -> [w296 w356]
      tunnel: [w300 w354] -> w281
      tunnel: [w296 w357] -> w280
      tunnel: w277 -> [_ w352]
      tunnel: w279 -> [_ w353]
      tunnel: w274 -> [w299 w359]
      tunnel: [w299 w359] -> w273
      tunnel: "STOP TASK" -> [_ w342]
      tunnel: w268 -> [w298 w358]
      tunnel: [w298 w355] -> w267
      tunnel: w264 -> [w297 w348]
      tunnel: [w297 w348] -> w263
      tunnel: w261 -> [_ w343]
      tunnel: [w295 w340] -> w260
      tunnel: w259 -> [w295 w339]
      tunnel: w257 -> [w294 w336]
      tunnel: [w294 w336] -> w256
      tunnel: w254 -> [w293 w332]
      tunnel: [w293 w332] -> w253
      tunnel: w251 -> [w292 w330]
      tunnel: [w292 w330] -> w250
      tunnel: w248 -> [w291 w328]
      tunnel: [w291 w328] -> w247
      tunnel: w246 -> [w290 w327]
      tunnel: [w290 w326] -> w245
      tunnel: [_ w324] -> w244
      tunnel: w242 -> [w289 w322]
      tunnel: [w289 w322] -> w241
      tunnel: w240 -> [w288 w321]
      tunnel: [w288 w320] -> w239
      tunnel: w237 -> [w287 w317]
      tunnel: [w287 w317] -> w236
      tunnel: [w286 w316] -> w234
      tunnel: w232 -> [w286 w315]
      tunnel: [_ w313] -> w231
      tunnel: [_ w312] -> w230
      tunnel: [_ w311] -> w229
      tunnel: w227 -> [w285 w310]
      tunnel: [w285 w310] -> w225
      tunnel: [_ w301] -> w224
      frame False {
        # ">>> Box Colour Detection >>>"
        # ">>> Line Sensor Cluster>>>"
        # ">> Item Selection Bias >>"
        # ">>State Logic Queue Reference >>"
        # ">>Action states Queue Reference >>"
        # ">>True Stop Next State >>"
        # ">>State Logic  >>"
        # ">>> IR Sensors >>>"
        # ">>> Line Sensor Cluster>>>"
        # ">>> Line Sensor Cluster>>>"
        # ">>> Motor control cluster >>>"
        # ">>> yStepper command>>>"
        # ">>> Motor control cluster >>>"
        # ">>> yStepper command>>>"
        # ">>> Motor control cluster >>>"
        # ">>> IR Sensors >>>"
        # ">>> IR Sensors >>>"
        # ">>> yStepper command>>>"
        # ">>> Time cluster >>>"
        # ">>> Yaw >>>"
        # ">>> Stepper position >>>"
        # ">>> Encoders >>>"
        # ">>> Object detection >>>"
        # ">>> Ultrasonic Sensors Detect >>>"
        # ">>> Time cluster >>>"
        # ">>> Yaw >>>"
        # ">>> Stepper position >>>"
        # ">>> Encoders >>>"
        # ">>> Object detection >>>"
        # ">>> Ultrasonic Sensors Detect >>>"
      }
      frame True {
        # ">>State Logic Queue Reference >>"
        # ">>> Box Colour Detection >>>"
        # ">> Item Selection Bias >>"
        # ">>> IR Sensors >>>"
        # ">>> Line Sensor Cluster>>>"
        # ">>> Line Sensor Cluster>>>"
        # ">>> Motor control cluster >>>"
        # ">>> yStepper command>>>"
        # ">>> IR Sensors >>>"
        # ">>> Motor control cluster >>>"
        # ">>State Logic Queue Reference >>"
        # ">>Timeout>>"
        # ">>> yStepper command>>>"
        # ">>> Time cluster >>>"
        # ">>> Object detection >>>"
        # ">>> Yaw >>>"
        # ">>> Ultrasonic Sensors Detect >>>"
        # ">>> Encoders >>>"
        # ">>> Stepper position >>>"
        # ">>State Logic  >>"
        # ">>True Stop Next State >>"
        # ">>Action Queue>>"
        # ">> Manual override >>"
        # ">>> Time cluster >>>"
        # ">>> Yaw >>>"
        # ">>> Stepper position >>>"
        # ">>> Encoders >>>"
        # ">>> Object detection >>>"
        # ">>> Ultrasonic Sensors Detect >>>"
        # ">>Action Queue>>"
        # ">>State Logic Queue Reference >>"
        n215 = Or(x=w342, y=w343) -> (x .or. y?=w341:bool)
        n216 = Unbundle By Name(w322) -> ("Left IR Sensor"=w323:dbl, "Arm IR Sensor"=w319:dbl, "Bottom IR Sensor"=w314:dbl)
        n217 = Unbundle By Name(w317) -> ("Line Detected?"=w318:bool)
        n218 = Unbundle By Name(w328) -> ("Time up flag"=w329:bool)
        n219 = Unbundle By Name(w330) -> ("Yaw"=w331:dbl, "Compass"=w325:dbl)
        n220 = Unbundle By Name(w332) -> ("y Stepper Position"=w334:u8, "z Stepper Position"=w333:u8)
        n221 = Unbundle By Name(w348) -> ("xDistance"=w345:dbl, "yDistance"=w346:dbl, "wDistance"=w347:dbl)
        n222 = Unbundle By Name(w336) -> ("Recognized Object"=w335:bool, "Object X coordinate"=w338:dbl, "Object Y coordinate"=w337:dbl)
        n223 = Unbundle By Name(w359) -> ("PING_A"=w351:u8, "PING_B"=w350:u8, "PING_C"=w349:u8, "PING_D"=w344:u8)
        n224 = Unbundle By Name(w310) -> ("Red"=w309:bool, "Black"=w308:bool, "Blue"=w307:bool, "Yellow"=w306:bool, "Green"=w305:bool, "Unknown"=w304:bool, "Image processing done"=w303:bool, "Colour"=w302:T2)
        n225 = case shown="\"Task 9I: ROTATE 90 CW\"" w358 {
          tunnel: [w364 w376 w390 w401 w519 w536 w582 w619 w674 w716 w764 w808 w863 w911 w955 w1015 w1056 w1099 w1148 w1191 w1244 w1282 w1334 w1378 w1422 w1452 w1470 w1518 w1559 w1608 w1661 w1700 w1749 w1792 w1845 w1883 w1935 w1972 w2020 w2063 w2113 w2157 w2205 w2261 w2302 w2354 w2403 w2446 w2494 w2545 w2583 w2629 w2678 w2719 w2763 w2811 w2857 w2904 w2945] -> w357
          tunnel: w356 -> [w364 w379 w391 w404 w521 w537 w583 w628 w672 w720 w765 w814 w856 w914 w962 w1005 w1059 w1105 w1147 w1194 w1234 w1288 w1324 w1373 w1413 w1452 w1460 w1521 w1565 w1607 w1660 w1706 w1748 w1795 w1835 w1889 w1925 w1976 w2027 w2068 w2118 w2162 w2206 w2259 w2303 w2355 w2405 w2453 w2499 w2544 w2587 w2635 w2677 w2723 w2767 w2815 w2864 w2909 w2955]
          tunnel: [State_Type_Definitions,_for_0.26g_versions_and_later_2."Idle" ("Enum") State_Type_Definitions,_for_0.26g_versions_and_later_2."Idle" ("Enum") w386 w403 State_Type_Definitions,_for_0.26g_versions_and_later_2."Shutdown" ("Enum") w538 w584 w626 w675 w717 w763 w809 w862 w912 w957 w1014 w1057 w1106 w1149 w1193 w1243 w1289 w1333 w1379 w1414 State_Type_Definitions,_for_0.26g_versions_and_later_2."Idle" ("Enum") w1469 w1519 w1566 w1609 w1662 w1707 w1750 w1794 w1844 w1890 w1934 w1973 w2021 w2064 w2114 w2158 w2204 w2262 w2301 w2353 w2404 w2448 w2500 w2546 w2584 w2630 w2679 w2720 w2764 w2812 w2858 w2905 w2950] -> w355
          tunnel: w354 -> [_ _ w389 w407 _ w542 w589 w622 w671 w721 w772 w813 w860 w915 w961 w1012 w1054 w1104 w1145 w1195 w1241 w1287 w1331 w1376 w1421 _ w1467 w1516 w1564 w1605 w1658 w1705 w1746 w1796 w1842 w1888 w1932 w1980 w2026 w2071 w2121 w2165 w2214 w2258 w2304 w2348 w2406 w2452 w2498 w2543 w2591 w2634 w2676 w2727 w2768 w2818 w2863 w2912 w2954]
          tunnel: w353 -> [_ _ _ w406 _ w541 w588 w621 w670 w722 w771 w812 w859 w908 w960 w1011 w1053 w1103 w1144 w1196 w1240 w1286 w1330 w1375 w1419 _ w1466 w1515 w1563 w1604 w1657 w1704 w1745 w1797 w1841 w1887 w1931 w1975 w2025 w2070 w2120 w2164 w2212 w2257 w2305 w2349 w2407 w2451 w2497 w2542 w2590 w2633 w2675 w2726 w2769 w2814 w2862 w2911 w2953]
          tunnel: w352 -> [_ _ w388 w402 _ w540 w587 w620 w669 w723 w770 w811 w858 w907 w959 w1013 w1055 w1102 w1143 w1197 w1242 w1285 w1332 w1374 w1420 _ w1468 w1517 w1562 w1603 w1656 w1703 w1744 w1798 w1843 w1886 w1933 w1979 w2024 w2069 w2119 w2163 w2213 w2256 w2306 w2350 w2408 w2450 w2496 w2541 w2589 w2632 w2674 w2725 w2770 w2817 w2861 w2910 w2952]
          tunnel: w341 -> [_ _ _ _ _ w527 w581 w627 w668 w724 w767 w807 w861 w913 w963 w1006 w1060 w1100 w1146 w1198 w1235 w1283 w1325 w1377 w1417 _ w1461 w1522 w1560 w1606 w1659 w1701 w1747 w1799 w1836 w1884 w1926 w1978 w2019 w2067 w2117 w2161 w2208 w2255 w2307 w2351 w2409 w2449 w2495 w2540 w2588 w2631 w2673 w2724 w2771 w2816 w2856 w2908 w2951]
          tunnel: w351 -> [_ _ _ _ _ _ _ _ _ _ _ _ _ _ _ _ _ _ _ _ _ _ _ _ _ _ _ _ _ _ _ _ _ _ _ _ _ _ _ _ _ _ _ _ _ _ _ _ _ _ _ _ _ _ _ _ _ _ _]
          tunnel: w350 -> [_ _ _ _ _ _ _ _ w667 _ _ _ w852 w896 w953 _ _ _ _ _ _ _ _ _ _ _ _ w1508 _ _ _ _ _ _ _ _ _ _ _ _ _ _ _ _ _ _ _ _ _ _ _ _ _ _ _ _ _ _ _]
          tunnel: w349 -> [_ _ _ _ _ _ _ _ w666 _ _ _ w853 w897 w954 _ _ _ _ _ _ _ _ _ _ _ _ w1509 _ _ _ _ _ _ _ _ _ _ _ _ _ _ _ _ _ _ _ _ _ _ _ _ _ _ _ _ _ _ _]
          tunnel: w347 -> [_ _ _ _ _ _ _ _ _ _ w769 _ _ _ _ _ _ _ _ _ _ _ _ _ _ _ _ _ _ _ _ _ _ _ _ _ _ _ _ _ _ _ _ _ _ w2346 _ _ _ _ _ _ _ _ _ _ _ _ w2948]
          tunnel: w346 -> [_ _ _ _ _ w535 w580 _ _ w715 _ _ _ _ w958 _ _ _ _ _ _ _ _ _ _ _ _ _ _ _ _ _ _ _ _ _ _ _ _ _ _ _ _ _ _ _ _ _ _ _ _ _ _ _ _ _ _ _ _]
          tunnel: w345 -> [_ _ _ _ _ _ _ _ _ _ _ _ _ w902 _ _ _ _ _ _ _ _ _ _ _ _ _ _ _ _ w1647 _ _ _ _ _ _ _ _ _ _ _ _ w2248 _ _ _ _ _ _ _ _ w2672 _ _ _ _ _ _]
          tunnel: w344 -> [_ _ _ _ _ _ _ _ _ _ _ _ _ _ _ _ _ _ _ _ _ _ _ _ _ _ _ _ _ _ _ _ _ _ _ _ _ _ _ _ _ _ _ _ _ _ _ _ _ _ _ _ _ _ _ _ _ _ _]
          tunnel: [State_Type_Definitions,_for_0.26g_versions_and_later_2."Idle" ("Enum") State_Type_Definitions,_for_0.26g_versions_and_later_2."Idle" ("Enum") State_Type_Definitions,_for_0.26g_versions_and_later_2."Idle" ("Enum") State_Type_Definitions,_for_0.26g_versions_and_later_2."Idle" ("Enum") State_Type_Definitions,_for_0.26g_versions_and_later_2."Shutdown" ("Enum") w533 w578 w625 w673 w718 w760 w806 w855 w910 w956 w1016 w1058 w1098 w1150 w1192 w1245 w1281 w1335 w1380 w1415 w1454 w1471 w1520 w1558 w1610 w1663 w1699 w1751 w1793 w1846 w1882 w1936 w1974 w2022 w2066 w2116 w2160 w2203 w2260 w2300 w2352 w2402 w2447 w2501 w2547 w2585 w2628 w2680 w2721 w2765 w2813 w2859 w2907 w2949] -> w340
          tunnel: w339 -> [_ _ w386 _ _ _ _ _ _ _ _ _ _ _ _ _ _ _ _ _ _ _ _ _ _ w1454 _ _ _ _ _ _ _ _ _ _ _ _ _ _ _ _ _ _ _ _ _ _ _ _ _ _ _ _ _ _ _ _ _]
          tunnel: w335 -> [_ _ _ _ _ _ _ _ _ _ _ _ _ _ _ _ _ _ _ _ _ _ _ _ w1416 _ _ _ _ _ _ _ _ _ _ _ _ _ _ _ _ _ _ _ _ _ _ _ _ _ _ _ _ _ _ _ _ _ _]
          tunnel: w338 -> [_ _ _ _ _ _ _ _ _ _ _ _ _ _ _ _ _ _ _ _ _ _ _ _ _ _ _ _ _ _ w1653 _ _ _ _ _ _ _ _ _ _ _ _ _ _ _ _ _ _ _ _ _ _ _ _ _ _ _ _]
          tunnel: w337 -> [_ _ _ _ _ _ _ _ _ _ _ _ _ _ _ _ _ _ _ w1187 _ _ _ _ _ _ _ _ _ _ _ _ _ w1788 _ _ _ _ _ _ _ _ _ _ _ _ _ _ _ _ _ _ _ _ _ _ _ _ _]
          tunnel: w334 -> [_ _ _ _ _ _ _ _ _ _ _ _ _ _ _ _ _ _ _ w1186 _ _ _ _ _ _ _ _ _ _ _ _ _ w1787 _ _ _ _ _ _ _ _ _ _ _ _ _ _ _ _ _ _ _ _ _ _ _ _ _]
          tunnel: w333 -> [_ _ _ _ _ _ _ w624 _ _ _ w804 _ _ _ w1009 _ w1094 _ _ w1238 _ w1328 w1372 _ _ w1464 _ _ _ _ _ _ _ w1839 _ w1929 w1977 _ _ _ _ _ _ _ _ _ _ _ _ _ _ _ _ _ _ _ _ _]
          tunnel: w331 -> [_ _ _ _ _ _ _ _ _ _ _ _ _ _ _ _ _ _ _ _ _ _ _ _ _ _ _ _ _ _ _ _ _ _ _ _ _ _ _ _ _ _ _ _ _ _ _ _ _ _ _ _ _ _ _ _ _ _ _]
          tunnel: w329 -> [_ _ _ _ _ _ _ _ _ _ _ _ _ _ _ _ w1048 _ w1140 _ _ w1279 _ _ _ _ _ _ w1556 w1600 _ w1697 w1741 _ _ w1880 _ _ _ _ _ _ _ _ _ _ _ _ _ _ w2586 w2627 _ w2722 w2766 _ _ _ _]
          tunnel: w327 -> [w362 w374 w385 w399 w517 w532 w577 w623 w665 w719 w759 w805 w854 w906 w952 w1004 w1051 w1097 w1141 w1189 w1233 w1280 w1323 w1369 w1412 w1455 w1459 w1513 w1557 w1601 w1654 w1698 w1742 w1790 w1834 w1881 w1924 w1971 w2023 w2065 w2115 w2159 w2211 w2254 w2309 w2357 w2411 w2455 w2503 w2549 w2593 w2637 w2685 w2729 w2773 w2810 w2860 w2906 w2957]
          tunnel: [w362 w373 w385 w399 w517 w532 w577 w623 w665 w719 w759 w805 w854 w906 w952 w1004 w1051 w1097 w1141 w1188 w1233 w1280 w1323 w1369 w1412 w1455 w1459 w1513 w1557 w1601 w1654 w1698 w1742 w1789 w1834 w1881 w1924 w1971 w2023 w2065 w2115 w2159 w2211 w2254 w2309 w2357 w2411 w2455 w2503 w2549 w2593 w2637 w2685 w2729 w2773 w2810 w2860 w2906 w2957] -> w326
          tunnel: w325 -> [_ _ _ _ _ _ _ _ _ _ _ _ _ _ _ _ _ _ _ _ _ _ _ _ _ _ _ _ _ _ _ _ _ _ _ _ _ _ w2018 _ _ _ _ _ _ _ _ _ _ _ _ _ _ _ _ _ w2855 _ _]
          tunnel: [_ _ _ TRUE _ _ _ _ _ _ _ _ _ _ _ _ _ _ _ _ _ _ _ _ _ _ _ _ _ _ _ _ _ _ _ _ _ w1968 w2013 w2060 w2104 w2154 w2198 w2247 w2295 w2345 w2391 _ _ _ _ _ _ _ _ _ _ _ _] -> w324
          tunnel: w323 -> [_ _ _ _ _ _ _ _ _ _ _ _ _ _ _ _ _ _ _ _ _ _ _ _ _ _ _ _ _ _ _ _ _ _ _ _ _ _ _ _ _ _ _ _ _ _ _ _ _ _ _ _ _ _ _ _ _ _ _]
          tunnel: w321 -> [w361 w371 w384 w397 w516 w531 w576 w618 w664 w712 w758 w801 w847 w895 w951 w1003 w1050 w1096 w1139 w1183 w1232 w1278 w1322 w1368 w1411 w1456 w1458 w1507 w1555 w1599 w1650 w1696 w1740 w1784 w1833 w1879 w1923 w1970 w2015 w2062 w2112 w2156 w2210 w2253 w2311 w2359 w2413 w2457 w2505 w2551 w2595 w2639 w2687 w2731 w2775 w2809 w2851 w2903 w2959]
          tunnel: [w361 w370 w384 w397 w516 w531 w576 w618 w664 w712 w758 w801 w847 w895 w951 w1003 w1050 w1096 w1139 w1183 w1232 w1278 w1322 w1368 w1411 w1456 w1458 w1507 w1555 w1599 w1649 w1696 w1740 w1784 w1833 w1879 w1923 w1970 w2015 w2062 w2112 w2156 w2210 w2253 w2311 w2359 w2413 w2457 w2505 w2551 w2595 w2639 w2687 w2731 w2775 w2809 w2851 w2903 w2959] -> w320
          tunnel: w319 -> [_ _ _ _ _ _ _ _ _ _ _ _ _ _ _ _ _ _ _ _ _ _ _ _ _ _ _ _ _ _ _ _ _ _ _ _ _ _ _ _ w2110 _ _ _ _ _ w2400 _ _ _ _ _ _ _ _ _ _ _ _]
          tunnel: w318 -> [_ _ _ _ _ w528 _ _ _ _ _ _ _ _ w949 _ _ _ _ _ _ _ _ _ _ _ _ _ _ _ _ _ _ _ _ _ _ _ _ w2060 _ w2154 _ w2249 _ _ _ w2445 _ w2539 _ _ w2671 _ _ _ _ _ _]
          tunnel: [w360 w366 w383 w396 w515 w530 w575 w617 w663 w711 w757 w800 w846 w894 w950 w1002 w1049 w1095 w1138 w1182 w1231 w1277 w1321 w1367 w1410 w1451 w1457 w1506 w1554 w1598 w1642 w1695 w1739 w1783 w1832 w1878 w1922 w1969 w2014 w2061 w2109 w2155 w2209 w2252 w2310 w2358 w2412 w2456 w2504 w2550 w2594 w2638 w2686 w2730 w2774 w2808 w2850 w2902 w2958] -> w316
          tunnel: w315 -> [w360 w366 w383 _ w515 w530 w575 w617 w663 w711 w757 w800 w846 w894 w950 w1002 w1049 w1095 w1138 w1182 w1231 w1277 w1321 w1367 w1410 w1451 w1457 w1506 w1554 w1598 w1642 w1695 w1739 w1783 w1832 w1878 w1922 w1969 w2014 w2061 w2109 w2155 w2209 w2252 w2310 w2358 w2412 w2456 w2504 w2550 w2594 w2638 w2686 w2730 w2774 w2808 w2850 w2902 w2958]
          tunnel: w314 -> [_ _ _ _ _ _ _ _ _ _ _ _ _ _ _ _ _ _ _ _ _ _ _ _ _ _ _ w1505 _ _ _ _ _ _ _ _ _ _ _ _ w2108 _ _ _ _ _ w2394 _ _ _ _ _ _ _ _ _ _ w2899 _]
          tunnel: [_ _ _ _ _ _ _ _ w662 _ _ _ _ _ _ _ _ _ _ _ _ _ _ _ _ _ _ _ _ _ _ _ _ _ _ _ _ _ _ _ _ _ _ _ _ _ _ _ _ _ _ _ _ _ _ _ _ _ _] -> w313
          tunnel: [_ _ _ _ _ _ _ _ _ _ _ _ _ _ _ _ _ _ _ _ _ _ _ _ _ _ _ _ _ _ _ _ _ _ _ _ _ _ _ _ w2106 _ _ _ _ _ w2393 _ _ _ _ _ _ _ _ _ _ w2897 _] -> w312
          tunnel: [_ _ _ _ _ _ _ _ _ _ _ _ _ _ _ _ _ _ _ _ _ _ _ _ _ _ _ _ _ _ _ _ _ _ _ _ _ _ _ _ w2105 _ _ _ _ _ w2392 _ _ _ _ _ _ _ _ _ _ _ _] -> w311
          tunnel: w309 -> [_ _ _ _ _ _ _ _ _ _ _ _ _ _ _ _ _ _ _ _ _ _ _ _ _ _ _ _ _ _ _ _ _ _ _ _ _ _ _ _ _ _ _ _ _ _ _ _ _ _ _ _ _ _ _ _ _ _ _]
          tunnel: w308 -> [_ _ _ _ _ _ _ _ _ _ _ _ _ _ _ _ _ _ _ _ _ _ _ _ _ _ _ _ _ _ _ _ _ _ _ _ _ _ _ _ _ _ _ _ _ _ _ _ _ _ _ _ _ _ _ _ _ _ _]
          tunnel: w307 -> [_ _ _ _ _ _ _ _ _ _ _ _ _ _ _ _ _ _ _ _ _ _ _ _ _ _ _ _ _ _ _ _ _ _ _ _ _ _ _ _ _ _ _ _ _ _ _ _ _ _ _ _ _ _ _ _ _ _ _]
          tunnel: w306 -> [_ _ _ _ _ _ _ _ _ _ _ _ _ _ _ _ _ _ _ _ _ _ _ _ _ _ _ _ _ _ _ _ _ _ _ _ _ _ _ _ _ _ _ _ _ _ _ _ _ _ _ _ _ _ _ _ _ _ _]
          tunnel: w305 -> [_ _ _ _ _ _ _ _ _ _ _ _ _ _ _ _ _ _ _ _ _ _ _ _ _ _ _ _ _ _ _ _ _ _ _ _ _ _ _ _ _ _ _ _ _ _ _ _ _ _ _ _ _ _ _ _ _ _ _]
          tunnel: w304 -> [_ _ _ _ _ _ _ _ _ _ _ _ _ _ _ _ _ _ _ _ _ _ _ _ _ _ _ _ _ _ _ _ _ _ _ _ _ _ _ _ _ _ _ _ _ _ _ _ _ _ _ _ _ _ _ _ _ _ _]
          tunnel: w303 -> [_ _ _ _ _ _ _ _ _ _ _ _ _ _ _ _ _ _ _ _ _ _ _ _ _ _ _ _ _ _ _ _ _ _ _ _ _ _ _ _ _ _ w2198 _ w2295 _ _ _ w2489 _ _ _ _ _ _ w2807 _ _ _]
          tunnel: w302 -> [_ _ _ _ _ _ _ _ _ _ _ _ _ _ _ _ _ _ _ _ _ _ _ _ _ _ _ _ _ _ _ _ _ _ _ _ _ _ _ _ _ _ w2201 _ w2297 _ _ _ w2491 _ _ _ _ _ _ _ _ _ _]
          tunnel: [_ _ _ _ _ _ _ _ _ _ _ _ _ _ _ _ _ _ _ _ _ _ _ _ _ _ _ _ _ _ _ _ _ _ _ _ _ _ _ _ _ _ w2199 _ w2296 _ _ _ _ _ _ _ _ _ _ _ _ _ _] -> w301
          frame "None" {
            # ">>> yStepper command>>>"
          }
          frame "Startup" {
            # ">>> yStepper command>>>"
            n226 = for {
              shift-right: [w382] -> w376
              shift-left: w379 -> [w381]
              tunnel: string[] ["INIT", "RESET ARM", "RESET FLAGS", "RESET YAW", "NAVX CALIBRATE"] -> [w380] mode=indexing
              n227 = Enqueue Element(queue=w381, element=w380) -> (queue out=w382:refnum<queue>)  [unwired: 2 in, 2 out]
            }
            n228 = Bundle By Name(cluster=w374, "yStepper desired"=u8 0) -> (w373:T20)
            n229 = Bundle By Name(cluster=w371, "ySpeed"=0.0, "xSpeed"=0.0, "wSpeed"=0.0) -> (w370:T19)
          }
          frame "True Stop" {
            # ">>Action Queue>>"
            # ">>> Motor control cluster >>>"
            # ">>> yStepper command>>>"
            n230 = Flush Queue(queue=w389, error in (no error)=w388) -> ()  [unwired: 3 out]
            n231 = for {
              shift-right: [w395] -> w390
              shift-left: w391 -> [w394]
              tunnel: string[] ["STOP", "RESET ENCODERS", "RESET YAW", "RESET ARM", "RESET ALL SENSORS", "DISPOSE CAM BUFFERS", "DISPOSE PROC BUFFERS", "CAM CLOSE", ""] -> [w393] mode=indexing
              n232 = Enqueue Element(queue=w394, element=w393) -> (queue out=w395:refnum<queue>)  [unwired: 2 in, 2 out]
            }
          }
          frame "Idle", Default {
            # ">>> Motor control cluster >>>"
            # ">>> yStepper command>>>"
            n233 = Dequeue Element(queue=w407, timeout in ms (-1)=w406, error in (no error)=w402) -> (element=w405:T10)  [unwired: 3 out]
            n234 = case shown="\"Start Task 9\"" w405 {
              tunnel: [w410 w418 w426 w434 w442 w450 w458 w466 w474 w481 w491 w499 w506 w509] -> w401
              tunnel: w404 -> [w411 w419 w427 w435 w443 w451 w459 w467 w475 w482 w490 w498 w506 w510]
              tunnel: [State_Type_Definitions,_for_0.26g_versions_and_later_2."Task 1A" ("Enum") State_Type_Definitions,_for_0.26g_versions_and_later_2."Task 2:Raise Arm" ("Enum") State_Type_Definitions,_for_0.26g_versions_and_later_2."Task 3" ("Enum") State_Type_Definitions,_for_0.26g_versions_and_later_2."Task 4_A" ("Enum") State_Type_Definitions,_for_0.26g_versions_and_later_2."Task 5A" ("Enum") State_Type_Definitions,_for_0.26g_versions_and_later_2."Task 6_A" ("Enum") State_Type_Definitions,_for_0.26g_versions_and_later_2."Task 8A: RAISE ARM" ("Enum") State_Type_Definitions,_for_0.26g_versions_and_later_2."Task 8A: RAISE ARM" ("Enum") State_Type_Definitions,_for_0.26g_versions_and_later_2."Task 8A: RAISE ARM" ("Enum") State_Type_Definitions,_for_0.26g_versions_and_later_2."Task 8A: RAISE ARM" ("Enum") State_Type_Definitions,_for_0.26g_versions_and_later_2."Task 9A: Raise Arm" ("Enum") State_Type_Definitions,_for_0.26g_versions_and_later_2."Task A1: Task 9 Open cam" ("Enum") State_Type_Definitions,_for_0.26g_versions_and_later_2."Idle" ("Enum") State_Type_Definitions,_for_0.26g_versions_and_later_2."Shutdown" ("Enum")] -> w403
              tunnel: [enum16{"Ball", "Soap", "Gel", "Pipe", "None"}."None" ("Object recognition mode") enum16{"Ball", "Soap", "Gel", "Pipe", "None"}."None" ("Object recognition mode") enum16{"Ball", "Soap", "Gel", "Pipe", "None"}."None" ("Object recognition mode") enum16{"Ball", "Soap", "Gel", "Pipe", "None"}."None" ("Object recognition mode") enum16{"Ball", "Soap", "Gel", "Pipe", "None"}."None" ("Object recognition mode") enum16{"Ball", "Soap", "Gel", "Pipe", "None"}."None" ("Object recognition mode") enum16{"Ball", "Soap", "Gel", "Pipe", "None"}."Ball" ("Object recognition mode") enum16{"Ball", "Soap", "Gel", "Pipe", "None"}."Gel" ("Object recognition mode") enum16{"Ball", "Soap", "Gel", "Pipe", "None"}."Pipe" ("Object recognition mode") enum16{"Ball", "Soap", "Gel", "Pipe", "None"}."Soap" ("Object recognition mode") enum16{"Ball", "Soap", "Gel", "Pipe", "None"}."None" ("Object recognition mode") enum16{"Ball", "Soap", "Gel", "Pipe", "None"}."None" ("Object recognition mode") enum16{"Ball", "Soap", "Gel", "Pipe", "None"}."None" ("Object recognition mode") enum16{"Ball", "Soap", "Gel", "Pipe", "None"}."None" ("Object recognition mode")] -> w396
              frame "Start Task 1" {
                n235 = for {
                  shift-right: [w415] -> w410
                  shift-left: w411 -> [w414]
                  tunnel: string[] ["RESET ENCODERS", "RESET YAW", "FORWARD", "READ ENCODERS"] -> [w413] mode=indexing
                  n236 = Enqueue Element(queue=w414, element=w413) -> (queue out=w415:refnum<queue>)  [unwired: 2 in, 2 out]
                }
              }
              frame "Start Task 2" {
                n237 = for {
                  shift-right: [w423] -> w418
                  shift-left: w419 -> [w422]
                  tunnel: string[] ["RESET ENCODERS", "RESET YAW", "READ ULTRASONIC", "ARDUINO - ULTRASONIC"] -> [w421] mode=indexing
                  n238 = Enqueue Element(queue=w422, element=w421) -> (queue out=w423:refnum<queue>)  [unwired: 2 in, 2 out]
                }
              }
              frame "Start Task 3" {
                n239 = for {
                  shift-right: [w431] -> w426
                  shift-left: w427 -> [w430]
                  tunnel: string[] ["RESET ENCODERS", "READ ENCODERS", "R-ACW"] -> [w429] mode=indexing
                  n240 = Enqueue Element(queue=w430, element=w429) -> (queue out=w431:refnum<queue>)  [unwired: 2 in, 2 out]
                }
              }
              frame "Start Task 4" {
                n241 = for {
                  shift-right: [w439] -> w434
                  shift-left: w435 -> [w438]
                  tunnel: string[] ["RESET YAW", "RESET ENCODERS", "RESET ARM", "RESET FLAGS", "", ""] -> [w437] mode=indexing
                  n242 = Enqueue Element(queue=w438, element=w437) -> (queue out=w439:refnum<queue>)  [unwired: 2 in, 2 out]
                }
              }
              frame "Start Task 5" {
                n243 = for {
                  shift-right: [w447] -> w442
                  shift-left: w443 -> [w446]
                  tunnel: string[] ["RESET YAW", "RESET ENCODERS", "RESET ARM", "RESET ALL SENSORS", "", ""] -> [w445] mode=indexing
                  n244 = Enqueue Element(queue=w446, element=w445) -> (queue out=w447:refnum<queue>)  [unwired: 2 in, 2 out]
                }
              }
              frame "Start Task 6" {
                n245 = for {
                  shift-right: [w455] -> w450
                  shift-left: w451 -> [w454]
                  tunnel: string[] ["OPEN LOG CAM ", "", "", "", "", ""] -> [w453] mode=indexing
                  n246 = Enqueue Element(queue=w454, element=w453) -> (queue out=w455:refnum<queue>)  [unwired: 2 in, 2 out]
                }
              }
              frame "Start Task 8 - BALL" {
                n247 = for {
                  shift-right: [w463] -> w458
                  shift-left: w459 -> [w462]
                  tunnel: string[] ["RESET YAW", "RESET ENCODERS", "RESET ARM", "RESET FLAGS"] -> [w461] mode=indexing
                  n248 = Enqueue Element(queue=w462, element=w461) -> (queue out=w463:refnum<queue>)  [unwired: 2 in, 2 out]
                }
              }
              frame "Start Task 8 - Gel" {
                n249 = for {
                  shift-right: [w471] -> w466
                  shift-left: w467 -> [w470]
                  tunnel: string[] ["RESET YAW", "RESET ENCODERS", "RESET ARM", "RESET FLAGS"] -> [w469] mode=indexing
                  n250 = Enqueue Element(queue=w470, element=w469) -> (queue out=w471:refnum<queue>)  [unwired: 2 in, 2 out]
                }
              }
              frame "Start Task 8 - Pipe" {
                n251 = for {
                  shift-right: [w479] -> w474
                  shift-left: w475 -> [w478]
                  tunnel: string[] ["RESET YAW", "RESET ENCODERS", "RESET ARM", "RESET FLAGS"] -> [w477] mode=indexing
                  n252 = Enqueue Element(queue=w478, element=w477) -> (queue out=w479:refnum<queue>)  [unwired: 2 in, 2 out]
                }
              }
              frame "Start Task 8 - Soap" {
                n253 = for {
                  shift-right: [w487] -> w481
                  shift-left: w482 -> [w486]
                  tunnel: string[] ["RESET YAW", "RESET ENCODERS", "RESET ARM", "RESET FLAGS"] -> [w485] mode=indexing
                  n254 = Enqueue Element(queue=w486, element=w485) -> (queue out=w487:refnum<queue>)  [unwired: 2 in, 2 out]
                }
              }
              frame "Start Task 9" {
                n255 = for {
                  shift-right: [w495] -> w491
                  shift-left: w490 -> [w494]
                  tunnel: string[] ["Z STEPPER BOX HEIGHT", "READ STEPPER VALUES", "", ""] -> [w493] mode=indexing
                  n256 = Enqueue Element(queue=w494, element=w493) -> (queue out=w495:refnum<queue>)  [unwired: 2 in, 2 out]
                }
              }
              frame "Start Task A" {
                n257 = for {
                  shift-right: [w503] -> w499
                  shift-left: w498 -> [w502]
                  tunnel: string[] ["RESET ENCODERS", "READ ENCODERS", "RESET YAW", "Z STEPPER BOX HEIGHT"] -> [w501] mode=indexing
                  n258 = Enqueue Element(queue=w502, element=w501) -> (queue out=w503:refnum<queue>)  [unwired: 2 in, 2 out]
                }
              }
              frame "None", Default {
              }
              frame "Exit" {
                n259 = for {
                  shift-right: [w514] -> w509
                  shift-left: w510 -> [w513]
                  tunnel: string[] ["STOP", "RESET ENCODERS", "RESET YAW", "EXIT"] -> [w512] mode=indexing
                  n260 = Enqueue Element(queue=w513, element=w512) -> (queue out=w514:refnum<queue>)  [unwired: 2 in, 2 out]
                }
              }
            }
          }
          frame "Shutdown" {
            # ">> Item Selection Bias >>"
            # ">>> yStepper command>>>"
            n261 = for {
              shift-right: [w525] -> w519
              shift-left: w521 -> [w524]
              tunnel: string[] ["INIT", "RESET ENCODERS", "RESET FLAGS", "CAM CLOSE", "DISPOSE BUFFERS", "EXIT", ""] -> [w523] mode=indexing
              n262 = Enqueue Element(queue=w524, element=w523) -> (queue out=w525:refnum<queue>)  [unwired: 2 in, 2 out]
            }
          }
          frame "Task 1A" {
            # ">>> Motor control cluster >>>"
            # ">> Line detection >>"
            # ">> Checks if 1 metre moved >>"
            # ">>> yStepper command>>>"
            # "Use 250"
            n263 = Greater?(x=w535, y=265.0) -> (0:w529:bool)
            n264 = Dequeue Element(queue=w542, timeout in ms (-1)=w541, error in (no error)=w540) -> (element=w539:T10)  [unwired: 3 out]
            n265 = And(x=w528, y=w529) -> (x .and. y?=w526:bool)
            n266 = case shown="\"Start Task 1\", Default" w539 {
              tunnel: w527 -> [w543 _]
              tunnel: [w553 State_Type_Definitions,_for_0.26g_versions_and_later_2."True Stop" ("Enum")] -> w538
              tunnel: w537 -> [w551 w568]
              tunnel: [w550 w567] -> w536
              tunnel: [State_Type_Definitions,_for_0.26g_versions_and_later_2."Idle" ("Enum") State_Type_Definitions,_for_0.26g_versions_and_later_2."Shutdown" ("Enum")] -> w533
              tunnel: w526 -> [w544 _]
              frame "Start Task 1", Default {
                n267 = Or(x=w544, y=w543) -> (x .or. y?=w545:bool)
                n268 = case shown="True" w545 {
                  tunnel: w551 -> [w556 w562]
                  tunnel: [w555 w560] -> w550
                  frame False {
                    n269 = for {
                      shift-right: [w558] -> w555
                      shift-left: w556 -> [w559]
                      tunnel: string[] ["READ ENCODERS", "READ NAVX", "FORWARD", "READ LINE SENSOR"] ("element") -> [w557] mode=indexing
                      n270 = Enqueue Element(queue=w559, element=w557) -> (queue out=w558:refnum<queue>)  [unwired: 2 in, 2 out]
                    }
                  }
                  frame True {
                    n271 = for {
                      shift-right: [w564] -> w560
                      shift-left: w562 -> [w565]
                      tunnel: string[] ["RESET YAW", "RESET ENCODERS", "STOP", ""] -> [w563] mode=indexing
                      n272 = Enqueue Element(queue=w565, element=w563) -> (queue out=w564:refnum<queue>)  [unwired: 2 in, 2 out]
                    }
                  }
                }
                n273 = Select(t=State_Type_Definitions,_for_0.26g_versions_and_later_2."True Stop" ("Enum"), s=w543, f=State_Type_Definitions,_for_0.26g_versions_and_later_2."Task 1B" ("Enum")) -> (s? t:f=w548:T18)
                n274 = Select(t=w548, s=w544, f=State_Type_Definitions,_for_0.26g_versions_and_later_2."Task 1A" ("Enum")) -> (s? t:f=w553:T18)
              }
              frame "Exit" {
                n275 = for {
                  shift-right: [w572] -> w567
                  shift-left: w568 -> [w573]
                  tunnel: string[] ["STOP", "RESET ENCODERS", "RESET YAW", ""] -> [w571] mode=indexing
                  n276 = Enqueue Element(queue=w573, element=w571) -> (queue out=w572:refnum<queue>)  [unwired: 2 in, 2 out]
                }
              }
            }
          }
          frame "Task 1B" {
            # ">>> Motor control cluster >>>"
            # ">> Line detection >>"
            # ">> Adds small distance overhead after 1M >>"
            # ">>> yStepper command>>>"
            n277 = Greater?(x=w580, y=50.0) -> (0:w574:bool)
            n278 = Dequeue Element(queue=w589, timeout in ms (-1)=w588, error in (no error)=w587) -> (element=w586:T10)  [unwired: 3 out]
            n279 = Or(x=w574, y=w581) -> (x .or. y?=w585:bool)
            n280 = case shown="\"Start Task 1\", Default" w586 {
              tunnel: w585 -> [w592 _]
              tunnel: [w596 State_Type_Definitions,_for_0.26g_versions_and_later_2."True Stop" ("Enum")] -> w584
              tunnel: w583 -> [w593 w611]
              tunnel: [w591 w610] -> w582
              tunnel: [State_Type_Definitions,_for_0.26g_versions_and_later_2."Idle" ("Enum") State_Type_Definitions,_for_0.26g_versions_and_later_2."Shutdown" ("Enum")] -> w578
              frame "Start Task 1", Default {
                n281 = case shown="True" w592 {
                  tunnel: w593 -> [w599 w605]
                  tunnel: [w598 w603] -> w591
                  frame False {
                    n282 = for {
                      shift-right: [w601] -> w598
                      shift-left: w599 -> [w602]
                      tunnel: string[] ["READ ENCODERS", "READ NAVX", "FORWARD", "READ LINE SENSOR"] ("element") -> [w600] mode=indexing
                      n283 = Enqueue Element(queue=w602, element=w600) -> (queue out=w601:refnum<queue>)  [unwired: 2 in, 2 out]
                    }
                  }
                  frame True {
                    n284 = for {
                      shift-right: [w607] -> w603
                      shift-left: w605 -> [w608]
                      tunnel: string[] ["RESET YAW", "RESET ENCODERS", "STOP", ""] -> [w606] mode=indexing
                      n285 = Enqueue Element(queue=w608, element=w606) -> (queue out=w607:refnum<queue>)  [unwired: 2 in, 2 out]
                    }
                  }
                }
                n286 = Select(t=State_Type_Definitions,_for_0.26g_versions_and_later_2."True Stop" ("Enum"), s=w592, f=State_Type_Definitions,_for_0.26g_versions_and_later_2."Task 1B" ("Enum")) -> (s? t:f=w596:T18)
              }
              frame "Exit" {
                n287 = for {
                  shift-right: [w615] -> w610
                  shift-left: w611 -> [w616]
                  tunnel: string[] ["STOP", "RESET ENCODERS", "RESET YAW", ""] -> [w614] mode=indexing
                  n288 = Enqueue Element(queue=w616, element=w614) -> (queue out=w615:refnum<queue>)  [unwired: 2 in, 2 out]
                }
              }
            }
          }
          frame "Task 2:Raise Arm" {
            # ">> Stepper height reeached >>"
            # ">>> yStepper command>>>"
            # ">> Manual override >>"
            n289 = Dequeue Element(queue=w622, timeout in ms (-1)=w621, error in (no error)=w620) -> (element=w631:T10)  [unwired: 3 out]
            n290 = Equal?(x=w624, y=u8 60) -> (x = y?=w629:bool)
            n291 = case shown="\"Start Task 1\", Default" w631 {
              tunnel: [w642 State_Type_Definitions,_for_0.26g_versions_and_later_2."True Stop" ("Enum")] -> w626
              tunnel: [w640 w657] -> w619
              tunnel: w628 -> [w639 _]
              tunnel: w627 -> [w633 _]
              tunnel: [State_Type_Definitions,_for_0.26g_versions_and_later_2."Idle" ("Enum") State_Type_Definitions,_for_0.26g_versions_and_later_2."Shutdown" ("Enum")] -> w625
              tunnel: w629 -> [w632 _]
              frame "Start Task 1", Default {
                # ">> WIill proceed to part ii if not manual override >>"
                # ">>If ENABLE or Trigger is set to true>>"
                n292 = Or(x=w632, y=w633) -> (x .or. y?=w634:bool)
                n293 = case shown="True" w632 {
                  tunnel: [w645 w651] -> w640
                  tunnel: w639 -> [w644 w650]
                  frame False {
                    n294 = for {
                      shift-right: [w647] -> w645
                      shift-left: w644 -> [w648]
                      tunnel: string[] ["Z STEPPER CAM HEIGHT", "READ STEPPER VALUES"] ("element") -> [w646] mode=indexing
                      n295 = Enqueue Element(queue=w648, element=w646) -> (queue out=w647:refnum<queue>)  [unwired: 2 in, 2 out]
                    }
                  }
                  frame True {
                    n296 = for {
                      shift-right: [w653] -> w651
                      shift-left: w650 -> [w654]
                      tunnel: string[] ["ARDUINO - ULTRASONIC", "READ ULTRASONIC", "", "", "", ""] -> [w652] mode=indexing
                      n297 = Enqueue Element(queue=w654, element=w652) -> (queue out=w653:refnum<queue>)  [unwired: 2 in, 2 out]
                    }
                  }
                }
                n298 = Select(t=State_Type_Definitions,_for_0.26g_versions_and_later_2."True Stop" ("Enum"), s=w633, f=State_Type_Definitions,_for_0.26g_versions_and_later_2."Task 2:Sensor Mode" ("Enum")) -> (s? t:f=w636:T18)
                n299 = Select(t=w636, s=w634, f=State_Type_Definitions,_for_0.26g_versions_and_later_2."Task 2:Raise Arm" ("Enum")) -> (s? t:f=w642:T18)
              }
              frame "Exit" {
                n300 = for {
                  shift-right: [w660] -> w657
                  shift-left: _ -> [w661]
                  tunnel: string[] ["STOP", "RESET ENCODERS", "RESET YAW", ""] -> [w659] mode=indexing
                  n301 = Enqueue Element(queue=w661, element=w659) -> (queue out=w660:refnum<queue>)  [unwired: 2 in, 2 out]
                }
              }
            }
          }
          frame "Task 2:Sensor Mode" {
            w678 = u8 20 ("y")
            # ">>> yStepper command>>>"
            # ">>Object detected>>"
            n302 = Dequeue Element(queue=w671, timeout in ms (-1)=w670, error in (no error)=w669) -> (element=w679:T10)  [unwired: 3 out]
            n303 = Less?(x=w667, y=w678) -> (x < y?=w677:bool)
            n304 = Less?(x=w666, y=w678) -> (x < y?=w676:bool)
            n305 = Or(x=w677, y=w676) -> (x .or. y?=w662:bool)
            n306 = case shown="\"Start Task 1\", Default" w679 {
              tunnel: w662 -> [w682 _]
              tunnel: [w689 State_Type_Definitions,_for_0.26g_versions_and_later_2."True Stop" ("Enum")] -> w675
              tunnel: w668 -> [w681 _]
              tunnel: w672 -> [w688 w705]
              tunnel: [w687 w706] -> w674
              tunnel: [State_Type_Definitions,_for_0.26g_versions_and_later_2."Idle" ("Enum") State_Type_Definitions,_for_0.26g_versions_and_later_2."Shutdown" ("Enum")] -> w673
              frame "Start Task 1", Default {
                n307 = case shown="False" w682 {
                  tunnel: w688 -> [w692 w699]
                  tunnel: [w693 w698] -> w687
                  frame False {
                    n308 = for {
                      tunnel: string[] ["READ ULTRASONIC", "STOP"] ("element") -> [w694] mode=indexing
                      shift-right: [w696] -> w693
                      shift-left: w692 -> [w695]
                      n309 = Enqueue Element(queue=w695, element=w694) -> (queue out=w696:refnum<queue>)  [unwired: 2 in, 2 out]
                    }
                  }
                  frame True {
                    n310 = for {
                      shift-right: [w701] -> w698
                      shift-left: w699 -> [w702]
                      tunnel: string[] ["RESET ENCODERS", "READ NAVX", "READ ENCODERS"] -> [w700] mode=indexing
                      n311 = Enqueue Element(queue=w702, element=w700) -> (queue out=w701:refnum<queue>)  [unwired: 2 in, 2 out]
                    }
                  }
                }
                n312 = Or(x=w682, y=w681) -> (x .or. y?=w680:bool)
                n313 = Select(t=State_Type_Definitions,_for_0.26g_versions_and_later_2."True Stop" ("Enum"), s=w681, f=State_Type_Definitions,_for_0.26g_versions_and_later_2."Task 2:Reverse Mode" ("Enum")) -> (s? t:f=w683:T18)
                n314 = Select(t=w683, s=w680, f=State_Type_Definitions,_for_0.26g_versions_and_later_2."Task 2:Sensor Mode" ("Enum")) -> (s? t:f=w689:T18)
              }
              frame "Exit" {
                n315 = for {
                  shift-right: [w709] -> w706
                  shift-left: w705 -> [w710]
                  tunnel: string[] ["STOP", "RESET ENCODERS", "RESET YAW", "ARDUINO MODE 0"] -> [w708] mode=indexing
                  n316 = Enqueue Element(queue=w710, element=w708) -> (queue out=w709:refnum<queue>)  [unwired: 2 in, 2 out]
                }
              }
            }
          }
          frame "Task 2:Reverse Mode" {
            # ">>> yStepper command>>>"
            n317 = Dequeue Element(queue=w721, timeout in ms (-1)=w722, error in (no error)=w723) -> (element=w725:T10)  [unwired: 3 out]
            n318 = Less?(x=w715, y=-50.0) -> (x < y?=w713:bool)
            n319 = case shown="\"Start Task 1\", Default" w725 {
              tunnel: [w735 State_Type_Definitions,_for_0.26g_versions_and_later_2."True Stop" ("Enum")] -> w717
              tunnel: w724 -> [w728 _]
              tunnel: w720 -> [w734 w751]
              tunnel: [w733 w752] -> w716
              tunnel: [State_Type_Definitions,_for_0.26g_versions_and_later_2."Idle" ("Enum") State_Type_Definitions,_for_0.26g_versions_and_later_2."Shutdown" ("Enum")] -> w718
              tunnel: w713 -> [w726 _]
              frame "Start Task 1", Default {
                n320 = case shown="True" w726 {
                  tunnel: w734 -> [w738 w745]
                  tunnel: [w739 w744] -> w733
                  frame False {
                    n321 = for {
                      tunnel: string[] ["READ ENCODERS", "REVERSE", "READ NAVX"] ("element") -> [w740] mode=indexing
                      shift-right: [w742] -> w739
                      shift-left: w738 -> [w741]
                      n322 = Enqueue Element(queue=w741, element=w740) -> (queue out=w742:refnum<queue>)  [unwired: 2 in, 2 out]
                    }
                  }
                  frame True {
                    n323 = for {
                      shift-right: [w747] -> w744
                      shift-left: w745 -> [w748]
                      tunnel: string[] ["STOP", "ARDUINO - ULTRASONIC", "READ ULTRASONIC", "RESET ENCODERS"] -> [w746] mode=indexing
                      n324 = Enqueue Element(queue=w748, element=w746) -> (queue out=w747:refnum<queue>)  [unwired: 2 in, 2 out]
                    }
                  }
                }
                n325 = Or(x=w726, y=w728) -> (x .or. y?=w727:bool)
                n326 = Select(t=State_Type_Definitions,_for_0.26g_versions_and_later_2."True Stop" ("Enum"), s=w728, f=State_Type_Definitions,_for_0.26g_versions_and_later_2."Task 2:Sensor Mode" ("Enum")) -> (s? t:f=w729:T18)
                n327 = Select(t=w729, s=w727, f=State_Type_Definitions,_for_0.26g_versions_and_later_2."Task 2:Reverse Mode" ("Enum")) -> (s? t:f=w735:T18)
              }
              frame "Exit" {
                n328 = for {
                  shift-right: [w755] -> w752
                  shift-left: w751 -> [w756]
                  tunnel: string[] ["STOP", "RESET ENCODERS", "RESET YAW", "ARDUINO MODE 0"] -> [w754] mode=indexing
                  n329 = Enqueue Element(queue=w756, element=w754) -> (queue out=w755:refnum<queue>)  [unwired: 2 in, 2 out]
                }
              }
            }
          }
          frame "Task 3" {
            # ">>> Motor control cluster >>>"
            # ">>> yStepper command>>>"
            n330 = Dequeue Element(queue=w772, timeout in ms (-1)=w771, error in (no error)=w770) -> (element=w761:T10)  [unwired: 3 out]
            n331 = Less?(x=w769, y=-160.0) -> (x < y?=w766:bool)
            n332 = Or(x=w766, y=w767) -> (x .or. y?=w762:bool)
            n333 = case shown="\"Start Task 1\", Default" w761 {
              tunnel: w762 -> [w775 _]
              tunnel: [w779 State_Type_Definitions,_for_0.26g_versions_and_later_2."True Stop" ("Enum")] -> w763
              tunnel: w765 -> [w776 w795]
              tunnel: [w774 w794] -> w764
              tunnel: [State_Type_Definitions,_for_0.26g_versions_and_later_2."Idle" ("Enum") State_Type_Definitions,_for_0.26g_versions_and_later_2."Shutdown" ("Enum")] -> w760
              frame "Start Task 1", Default {
                n334 = case shown="False" w775 {
                  tunnel: w776 -> [w782 w788]
                  tunnel: [w781 w786] -> w774
                  frame False {
                    n335 = for {
                      shift-right: [w784] -> w781
                      shift-left: w782 -> [w785]
                      tunnel: string[] ["READ ENCODERS", "R-CW"] ("element") -> [w783] mode=indexing
                      n336 = Enqueue Element(queue=w785, element=w783) -> (queue out=w784:refnum<queue>)  [unwired: 2 in, 2 out]
                    }
                  }
                  frame True {
                    n337 = for {
                      shift-right: [w790] -> w786
                      shift-left: w788 -> [w791]
                      tunnel: string[] ["RESET YAW", "RESET ENCODERS", "STOP", "ARDUINO MODE 0"] -> [w789] mode=indexing
                      n338 = Enqueue Element(queue=w791, element=w789) -> (queue out=w790:refnum<queue>)  [unwired: 2 in, 2 out]
                    }
                  }
                }
                n339 = Select(t=State_Type_Definitions,_for_0.26g_versions_and_later_2."True Stop" ("Enum"), s=w775, f=State_Type_Definitions,_for_0.26g_versions_and_later_2."Task 3" ("Enum")) -> (s? t:f=w779:T18)
              }
              frame "Exit" {
                n340 = for {
                  shift-right: [w798] -> w794
                  shift-left: w795 -> [w799]
                  tunnel: string[] ["STOP", "RESET ENCODERS", "RESET YAW", ""] -> [w797] mode=indexing
                  n341 = Enqueue Element(queue=w799, element=w797) -> (queue out=w798:refnum<queue>)  [unwired: 2 in, 2 out]
                }
              }
            }
          }
          frame "Task 4_A" {
            # ">> Stepper height reeached >>"
            # ">>> yStepper command>>>"
            # ">> Manual override >>"
            n342 = Dequeue Element(queue=w813, timeout in ms (-1)=w812, error in (no error)=w811) -> (element=w810:T10)  [unwired: 3 out]
            n343 = Equal?(x=w804, y=u8 60) -> (x = y?=w802:bool)
            n344 = case shown="\"Start Task 1\", Default" w810 {
              tunnel: [w825 State_Type_Definitions,_for_0.26g_versions_and_later_2."True Stop" ("Enum")] -> w809
              tunnel: [w823 w841] -> w808
              tunnel: w814 -> [w822 w838]
              tunnel: w807 -> [w816 _]
              tunnel: [State_Type_Definitions,_for_0.26g_versions_and_later_2."Idle" ("Enum") State_Type_Definitions,_for_0.26g_versions_and_later_2."Shutdown" ("Enum")] -> w806
              tunnel: w802 -> [w815 _]
              frame "Start Task 1", Default {
                # ">> WIill proceed to part ii if not manual override >>"
                # ">>If ENABLE or Trigger is set to true>>"
                n345 = Or(x=w815, y=w816) -> (x .or. y?=w817:bool)
                n346 = case shown="False" w815 {
                  tunnel: [w828 w834] -> w823
                  tunnel: w822 -> [w827 w833]
                  frame False {
                    n347 = for {
                      shift-right: [w830] -> w828
                      shift-left: w827 -> [w831]
                      tunnel: string[] ["Z STEPPER CAM HEIGHT", "READ STEPPER VALUES"] ("element") -> [w829] mode=indexing
                      n348 = Enqueue Element(queue=w831, element=w829) -> (queue out=w830:refnum<queue>)  [unwired: 2 in, 2 out]
                    }
                  }
                  frame True {
                    n349 = for {
                      shift-right: [w836] -> w834
                      shift-left: w833 -> [w837]
                      tunnel: string[] ["ARDUINO - ULTRASONIC", "READ ULTRASONIC", "FORWARD", "", "", ""] -> [w835] mode=indexing
                      n350 = Enqueue Element(queue=w837, element=w835) -> (queue out=w836:refnum<queue>)  [unwired: 2 in, 2 out]
                    }
                  }
                }
                n351 = Select(t=State_Type_Definitions,_for_0.26g_versions_and_later_2."True Stop" ("Enum"), s=w816, f=State_Type_Definitions,_for_0.26g_versions_and_later_2."Task 4_B" ("Enum")) -> (s? t:f=w819:T18)
                n352 = Select(t=w819, s=w817, f=State_Type_Definitions,_for_0.26g_versions_and_later_2."Task 4_A" ("Enum")) -> (s? t:f=w825:T18)
              }
              frame "Exit" {
                n353 = for {
                  shift-right: [w844] -> w841
                  shift-left: w838 -> [w845]
                  tunnel: string[] ["STOP", "RESET ENCODERS", "RESET YAW", ""] -> [w843] mode=indexing
                  n354 = Enqueue Element(queue=w845, element=w843) -> (queue out=w844:refnum<queue>)  [unwired: 2 in, 2 out]
                }
              }
            }
          }
          frame "Task 4_B" {
            w851 = u8 20
            # ">> Path blocked >>"
            # ">>> yStepper command>>>"
            # ">> Manual override >>"
            n355 = Dequeue Element(queue=w860, timeout in ms (-1)=w859, error in (no error)=w858) -> (element=w857:T10)  [unwired: 3 out]
            n356 = Less?(x=w853, y=w851) -> (x < y?=w848:bool)
            n357 = Less?(x=w852, y=w851) -> (x < y?=w849:bool)
            n358 = And(x=w849, y=w848) -> (x .and. y?=w850:bool)
            n359 = case shown="\"Start Task 1\", Default" w857 {
              tunnel: [w874 State_Type_Definitions,_for_0.26g_versions_and_later_2."True Stop" ("Enum")] -> w862
              tunnel: [w872 w889] -> w863
              tunnel: w856 -> [w871 _]
              tunnel: w861 -> [w865 _]
              tunnel: [State_Type_Definitions,_for_0.26g_versions_and_later_2."Idle" ("Enum") State_Type_Definitions,_for_0.26g_versions_and_later_2."Shutdown" ("Enum")] -> w855
              tunnel: w850 -> [w864 _]
              frame "Start Task 1", Default {
                # ">> Manual override forces program to true stop >>"
                # ">>If ENABLE or Trigger is set to true>>"
                n360 = Or(x=w864, y=w865) -> (x .or. y?=w870:bool)
                n361 = case shown="False" w864 {
                  tunnel: [w877 w882] -> w872
                  tunnel: w871 -> [w876 w881]
                  frame False {
                    n362 = for {
                      shift-right: [w879] -> w877
                      shift-left: w876 -> [w880]
                      tunnel: string[] ["FORWARD", "READ ULTRASONIC", "READ NAVX"] ("element") -> [w878] mode=indexing
                      n363 = Enqueue Element(queue=w880, element=w878) -> (queue out=w879:refnum<queue>)  [unwired: 2 in, 2 out]
                    }
                  }
                  frame True {
                    n364 = for {
                      shift-right: [w885] -> w882
                      shift-left: w881 -> [w886]
                      tunnel: string[] ["STOP", "RESET YAW", "RESET ENCODERS", "RESET FLAGS"] -> [w884] mode=indexing
                      n365 = Enqueue Element(queue=w886, element=w884) -> (queue out=w885:refnum<queue>)  [unwired: 2 in, 2 out]
                    }
                  }
                }
                n366 = Select(t=State_Type_Definitions,_for_0.26g_versions_and_later_2."True Stop" ("Enum"), s=w865, f=State_Type_Definitions,_for_0.26g_versions_and_later_2."Task 4_C" ("Enum")) -> (s? t:f=w867:T18)
                n367 = Select(t=w867, s=w870, f=State_Type_Definitions,_for_0.26g_versions_and_later_2."Task 4_B" ("Enum")) -> (s? t:f=w874:T18)
              }
              frame "Exit" {
                n368 = for {
                  shift-right: [w892] -> w889
                  shift-left: _ -> [w893]
                  tunnel: string[] ["STOP", "RESET ENCODERS", "RESET YAW", ""] -> [w891] mode=indexing
                  n369 = Enqueue Element(queue=w893, element=w891) -> (queue out=w892:refnum<queue>)  [unwired: 2 in, 2 out]
                }
              }
            }
          }
          frame "Task 4_C" {
            w905 = u8 20
            # ">> xDistance travelled>>"
            # ">> Path NOT blocked >>"
            # ">>> yStepper command>>>"
            # ">> Manual override >>"
            n370 = Dequeue Element(queue=w915, timeout in ms (-1)=w908, error in (no error)=w907) -> (element=w909:T10)  [unwired: 3 out]
            n371 = Greater?(x=w897, y=w905) -> (0:w903:bool)
            n372 = Greater?(x=w902, y=80.0) -> (0:w900:bool)
            n373 = Greater?(x=w896, y=w905) -> (0:w904:bool)
            n374 = And(x=w904, y=w903) -> (x .and. y?=w899:bool)
            n375 = And(x=w900, y=w899) -> (x .and. y?=w898:bool)
            n376 = case shown="\"Start Task 1\", Default" w909 {
              tunnel: [w926 State_Type_Definitions,_for_0.26g_versions_and_later_2."True Stop" ("Enum")] -> w912
              tunnel: [w924 w942] -> w911
              tunnel: w914 -> [w923 w939]
              tunnel: w913 -> [w917 _]
              tunnel: [State_Type_Definitions,_for_0.26g_versions_and_later_2."Idle" ("t") State_Type_Definitions,_for_0.26g_versions_and_later_2."Shutdown" ("Enum")] -> w910
              tunnel: w898 -> [w916 _]
              frame "Start Task 1", Default {
                # ">> Manual override forces program to true stop >>"
                # ">>If ENABLE or Trigger is set to true>>"
                n377 = Or(x=w916, y=w917) -> (x .or. y?=w922:bool)
                n378 = case shown="False" w916 {
                  tunnel: [w929 w934] -> w924
                  tunnel: w923 -> [w927 w933]
                  frame False {
                    n379 = for {
                      shift-right: [w931] -> w929
                      shift-left: w927 -> [w932]
                      tunnel: string[] ["RIGHT", "READ NAVX", "READ ENCODERS", "READ ULTRASONIC"] ("element") -> [w930] mode=indexing
                      n380 = Enqueue Element(queue=w932, element=w930) -> (queue out=w931:refnum<queue>)  [unwired: 2 in, 2 out]
                    }
                  }
                  frame True {
                    n381 = for {
                      shift-right: [w937] -> w934
                      shift-left: w933 -> [w938]
                      tunnel: string[] ["STOP", "RESET YAW", "RESET ENCODERS", "ARDUINO - ULTRASONIC"] -> [w936] mode=indexing
                      n382 = Enqueue Element(queue=w938, element=w936) -> (queue out=w937:refnum<queue>)  [unwired: 2 in, 2 out]
                    }
                  }
                }
                n383 = Select(t=State_Type_Definitions,_for_0.26g_versions_and_later_2."True Stop" ("Enum"), s=w917, f=State_Type_Definitions,_for_0.26g_versions_and_later_2."Task 4_D" ("Enum")) -> (s? t:f=w918:T18)
                n384 = Select(t=w918, s=w922, f=State_Type_Definitions,_for_0.26g_versions_and_later_2."Task 4_C" ("Enum")) -> (s? t:f=w926:T18)
              }
              frame "Exit" {
                n385 = for {
                  shift-right: [w945] -> w942
                  shift-left: w939 -> [w946]
                  tunnel: string[] ["STOP", "RESET ENCODERS", "RESET YAW", ""] -> [w944] mode=indexing
                  n386 = Enqueue Element(queue=w946, element=w944) -> (queue out=w945:refnum<queue>)  [unwired: 2 in, 2 out]
                }
              }
            }
          }
          frame "Task 4_D" {
            w969 = u8 20
            # ">>> Motor control cluster >>>"
            # ">> Line detected >>"
            # ">> yDistance travelled>>"
            # ">> Path blocked >>"
            # ">>> yStepper command>>>"
            # ">> Manual override >>"
            n387 = Less?(x=w954, y=w969) -> (x < y?=w967:bool)
            n388 = Greater?(x=w958, y=200.0) -> (0:w965:bool)
            n389 = Less?(x=w953, y=w969) -> (x < y?=w968:bool)
            n390 = And(x=w968, y=w967) -> (x .and. y?=w964:bool)
            n391 = Dequeue Element(queue=w961, timeout in ms (-1)=w960, error in (no error)=w959) -> (element=w970:T10)  [unwired: 3 out]
            n392 = Or(x=w965, y=w964) -> (x .or. y?=w948:bool)
            n393 = And(x=w949, y=w948) -> (x .and. y?=w947:bool)
            n394 = case shown="\"Start Task 1\", Default" w970 {
              tunnel: [w981 State_Type_Definitions,_for_0.26g_versions_and_later_2."True Stop" ("Enum")] -> w957
              tunnel: [w979 w997] -> w955
              tunnel: w962 -> [w978 w994]
              tunnel: w963 -> [w972 _]
              tunnel: [State_Type_Definitions,_for_0.26g_versions_and_later_2."Idle" ("t") State_Type_Definitions,_for_0.26g_versions_and_later_2."Shutdown" ("Enum")] -> w956
              tunnel: w947 -> [w971 _]
              frame "Start Task 1", Default {
                # ">> Manual override forces program to true stop >>"
                # ">>If ENABLE or Trigger is set to true>>"
                n395 = Or(x=w971, y=w972) -> (x .or. y?=w977:bool)
                n396 = case shown="False" w971 {
                  tunnel: [w984 w989] -> w979
                  tunnel: w978 -> [w982 w988]
                  frame False {
                    n397 = for {
                      shift-right: [w986] -> w984
                      shift-left: w982 -> [w987]
                      tunnel: string[] ["FORWARD", "READ NAVX", "READ ENCODERS", "READ ULTRASONIC", "READ LINE SENSOR"] ("element") -> [w985] mode=indexing
                      n398 = Enqueue Element(queue=w987, element=w985) -> (queue out=w986:refnum<queue>)  [unwired: 2 in, 2 out]
                    }
                  }
                  frame True {
                    n399 = for {
                      shift-right: [w992] -> w989
                      shift-left: w988 -> [w993]
                      tunnel: string[] ["STOP", "RESET YAW", "RESET ENCODERS", "RESET FLAGS"] -> [w991] mode=indexing
                      n400 = Enqueue Element(queue=w993, element=w991) -> (queue out=w992:refnum<queue>)  [unwired: 2 in, 2 out]
                    }
                  }
                }
                n401 = Select(t=State_Type_Definitions,_for_0.26g_versions_and_later_2."True Stop" ("Enum"), s=w972, f=State_Type_Definitions,_for_0.26g_versions_and_later_2."True Stop" ("Enum")) -> (s? t:f=w973:T18)
                n402 = Select(t=w973, s=w977, f=State_Type_Definitions,_for_0.26g_versions_and_later_2."Task 4_D" ("Enum")) -> (s? t:f=w981:T18)
              }
              frame "Exit" {
                n403 = for {
                  shift-right: [w1000] -> w997
                  shift-left: w994 -> [w1001]
                  tunnel: string[] ["STOP", "RESET ENCODERS", "RESET YAW", ""] -> [w999] mode=indexing
                  n404 = Enqueue Element(queue=w1001, element=w999) -> (queue out=w1000:refnum<queue>)  [unwired: 2 in, 2 out]
                }
              }
            }
          }
          frame "Task 5A" {
            # "Stays in Task 5_A until stepper reaches desired \nheight"
            # ">>> Motor control cluster >>>"
            # ">>> yStepper command>>>"
            # ">> Manual override >>"
            n405 = Dequeue Element(queue=w1012, timeout in ms (-1)=w1011, error in (no error)=w1013) -> (element=w1010:T10)  [unwired: 3 out]
            n406 = Equal?(x=w1009, y=u8 1) -> (x = y?=w1007:bool)
            n407 = case shown="\"Start Task 1\", Default" w1010 {
              tunnel: [w1023 State_Type_Definitions,_for_0.26g_versions_and_later_2."True Stop" ("Enum")] -> w1014
              tunnel: [w1026 w1043] -> w1015
              tunnel: [State_Type_Definitions,_for_0.26g_versions_and_later_2."Idle" ("Enum") State_Type_Definitions,_for_0.26g_versions_and_later_2."Shutdown" ("Enum")] -> w1016
              tunnel: w1007 -> [w1022 _]
              tunnel: w1006 -> [w1021 _]
              tunnel: w1005 -> [w1017 w1040]
              frame "Start Task 1", Default {
                # "T: Go back to idle, F: Continue with task\""
                # ">> Manual override >>"
                n408 = case shown="True" w1022 {
                  tunnel: [w1030 w1036] -> w1026
                  tunnel: w1017 -> [w1028 w1034]
                  frame False {
                    n409 = for {
                      tunnel: string[] ["Z STEPPER GRAB HEIGHT", "READ STEPPER VALUES"] ("element") -> [w1031] mode=indexing
                      shift-right: [w1033] -> w1030
                      shift-left: w1028 -> [w1032]
                      n410 = Enqueue Element(queue=w1032, element=w1031) -> (queue out=w1033:refnum<queue>)  [unwired: 2 in, 2 out]
                    }
                  }
                  frame True {
                    n411 = for {
                      shift-right: [w1038] -> w1036
                      shift-left: w1034 -> [w1039]
                      tunnel: string[] ["SET TIMER 2", "", ""] -> [w1037] mode=indexing
                      n412 = Enqueue Element(queue=w1039, element=w1037) -> (queue out=w1038:refnum<queue>)  [unwired: 2 in, 2 out]
                    }
                  }
                }
                n413 = Or(x=w1022, y=w1021) -> (x .or. y?=w1024:bool)
                n414 = Select(t=State_Type_Definitions,_for_0.26g_versions_and_later_2."True Stop" ("Enum"), s=w1021, f=State_Type_Definitions,_for_0.26g_versions_and_later_2."Task 5B" ("Enum")) -> (s? t:f=w1018:T18)
                n415 = Select(t=w1018, s=w1024, f=State_Type_Definitions,_for_0.26g_versions_and_later_2."Task 5A" ("Enum")) -> (s? t:f=w1023:T18)
              }
              frame "Exit" {
                n416 = for {
                  shift-right: [w1046] -> w1043
                  shift-left: w1040 -> [w1047]
                  tunnel: string[] ["STOP", "RESET ENCODERS", "RESET YAW", "ARDUINO MODE 0"] -> [w1045] mode=indexing
                  n417 = Enqueue Element(queue=w1047, element=w1045) -> (queue out=w1046:refnum<queue>)  [unwired: 2 in, 2 out]
                }
              }
            }
          }
          frame "Task 5B" {
            # ">>> yStepper command>>>"
            n418 = Dequeue Element(queue=w1054, timeout in ms (-1)=w1053, error in (no error)=w1055) -> (element=w1052:T10)  [unwired: 3 out]
            n419 = case shown="\"Start Task 1\", Default" w1052 {
              tunnel: [w1067 State_Type_Definitions,_for_0.26g_versions_and_later_2."True Stop" ("Enum")] -> w1057
              tunnel: [w1070 w1087] -> w1056
              tunnel: [State_Type_Definitions,_for_0.26g_versions_and_later_2."Idle" ("Enum") State_Type_Definitions,_for_0.26g_versions_and_later_2."Shutdown" ("Enum")] -> w1058
              tunnel: w1060 -> [w1066 _]
              tunnel: w1059 -> [w1062 w1084]
              tunnel: w1048 -> [w1061 _]
              frame "Start Task 1", Default {
                # "T: Go back to idle, F: Continue with task\""
                # ">> Manual override >>"
                n420 = case shown="True" w1061 {
                  tunnel: [w1074 w1080] -> w1070
                  tunnel: w1062 -> [w1072 w1078]
                  frame False {
                    n421 = for {
                      tunnel: string[] ["CLOSE CLAW", "START TIMER", ""] ("element") -> [w1075] mode=indexing
                      shift-right: [w1077] -> w1074
                      shift-left: w1072 -> [w1076]
                      n422 = Enqueue Element(queue=w1076, element=w1075) -> (queue out=w1077:refnum<queue>)  [unwired: 2 in, 2 out]
                    }
                  }
                  frame True {
                    n423 = for {
                      shift-right: [w1082] -> w1080
                      shift-left: w1078 -> [w1083]
                      tunnel: string[] ["STOP", "", "", ""] -> [w1081] mode=indexing
                      n424 = Enqueue Element(queue=w1083, element=w1081) -> (queue out=w1082:refnum<queue>)  [unwired: 2 in, 2 out]
                    }
                  }
                }
                n425 = Or(x=w1061, y=w1066) -> (x .or. y?=w1068:bool)
                n426 = Select(t=State_Type_Definitions,_for_0.26g_versions_and_later_2."True Stop" ("Enum"), s=w1066, f=State_Type_Definitions,_for_0.26g_versions_and_later_2."Task 5C" ("Enum")) -> (s? t:f=w1063:T18)
                n427 = Select(t=w1063, s=w1068, f=State_Type_Definitions,_for_0.26g_versions_and_later_2."Task 5B" ("Enum")) -> (s? t:f=w1067:T18)
              }
              frame "Exit" {
                n428 = for {
                  shift-right: [w1090] -> w1087
                  shift-left: w1084 -> [w1091]
                  tunnel: string[] ["STOP", "RESET ENCODERS", "RESET YAW", "ARDUINO MODE 0"] -> [w1089] mode=indexing
                  n429 = Enqueue Element(queue=w1091, element=w1089) -> (queue out=w1090:refnum<queue>)  [unwired: 2 in, 2 out]
                }
              }
            }
          }
          frame "Task 5C" {
            # ">>> Motor control cluster >>>"
            # ">>> yStepper command>>>"
            # ">> Manual override >>"
            n430 = Equal?(x=w1094, y=u8 60) -> (x = y?=w1092:bool)
            n431 = Dequeue Element(queue=w1104, timeout in ms (-1)=w1103, error in (no error)=w1102) -> (element=w1101:T10)  [unwired: 3 out]
            n432 = case shown="\"Start Task 1\", Default" w1101 {
              tunnel: [w1113 State_Type_Definitions,_for_0.26g_versions_and_later_2."True Stop" ("Enum")] -> w1106
              tunnel: [w1116 w1133] -> w1099
              tunnel: [State_Type_Definitions,_for_0.26g_versions_and_later_2."Idle" ("Enum") State_Type_Definitions,_for_0.26g_versions_and_later_2."Shutdown" ("Enum")] -> w1098
              tunnel: w1100 -> [w1107 _]
              tunnel: w1105 -> [w1112 w1130]
              tunnel: w1092 -> [w1111 _]
              frame "Start Task 1", Default {
                # ">> Is time up? >>"
                # "Determines if object is in range to pick up"
                # ">> Manual override >>"
                n433 = case shown="True" w1111 {
                  tunnel: [w1120 w1126] -> w1116
                  tunnel: w1112 -> [w1118 w1124]
                  frame False {
                    n434 = for {
                      tunnel: string[] ["Z STEPPER CAM HEIGHT", "READ STEPPER VALUES"] ("element") -> [w1121] mode=indexing
                      shift-right: [w1123] -> w1120
                      shift-left: w1118 -> [w1122]
                      n435 = Enqueue Element(queue=w1122, element=w1121) -> (queue out=w1123:refnum<queue>)  [unwired: 2 in, 2 out]
                    }
                  }
                  frame True {
                    n436 = for {
                      shift-right: [w1128] -> w1126
                      shift-left: w1124 -> [w1129]
                      tunnel: string[] ["SET TIMER 5", "", ""] -> [w1127] mode=indexing
                      n437 = Enqueue Element(queue=w1129, element=w1127) -> (queue out=w1128:refnum<queue>)  [unwired: 2 in, 2 out]
                    }
                  }
                }
                n438 = Or(x=w1111, y=w1107) -> (x .or. y?=w1114:bool)
                n439 = Select(t=State_Type_Definitions,_for_0.26g_versions_and_later_2."True Stop" ("Enum"), s=w1107, f=State_Type_Definitions,_for_0.26g_versions_and_later_2."Task 5D" ("Enum")) -> (s? t:f=w1109:T18)
                n440 = Select(t=w1109, s=w1114, f=State_Type_Definitions,_for_0.26g_versions_and_later_2."Task 5C" ("Enum")) -> (s? t:f=w1113:T18)
              }
              frame "Exit" {
                n441 = for {
                  shift-right: [w1136] -> w1133
                  shift-left: w1130 -> [w1137]
                  tunnel: string[] ["STOP", "RESET ENCODERS", "RESET YAW", "ARDUINO MODE 0"] -> [w1135] mode=indexing
                  n442 = Enqueue Element(queue=w1137, element=w1135) -> (queue out=w1136:refnum<queue>)  [unwired: 2 in, 2 out]
                }
              }
            }
          }
          frame "Task 5D" {
            # ">>> yStepper command>>>"
            n443 = Dequeue Element(queue=w1145, timeout in ms (-1)=w1144, error in (no error)=w1143) -> (element=w1142:T10)  [unwired: 3 out]
            n444 = case shown="\"Start Task 1\", Default" w1142 {
              tunnel: [w1157 State_Type_Definitions,_for_0.26g_versions_and_later_2."True Stop" ("Enum")] -> w1149
              tunnel: [w1160 w1177] -> w1148
              tunnel: [State_Type_Definitions,_for_0.26g_versions_and_later_2."Idle" ("Enum") State_Type_Definitions,_for_0.26g_versions_and_later_2."Shutdown" ("Enum")] -> w1150
              tunnel: w1146 -> [w1156 _]
              tunnel: w1147 -> [w1152 w1174]
              tunnel: w1140 -> [w1151 _]
              frame "Start Task 1", Default {
                # ">> T: Breaks out of state loop; F: Stays in loop>>"
                # ">> Manual override >>"
                # ">> Checks if time is up>>"
                # "Stays in Task 5D until the object is detected"
                # "T: Go back to idle, F: Continue with task\""
                # ">> Manual override >>"
                n445 = case shown="False" w1151 {
                  tunnel: [w1164 w1170] -> w1160
                  tunnel: w1152 -> [w1162 w1168]
                  frame False {
                    n446 = for {
                      tunnel: string[] ["START TIMER", "OPEN CLAW", ""] ("element") -> [w1165] mode=indexing
                      shift-right: [w1167] -> w1164
                      shift-left: w1162 -> [w1166]
                      n447 = Enqueue Element(queue=w1166, element=w1165) -> (queue out=w1167:refnum<queue>)  [unwired: 2 in, 2 out]
                    }
                  }
                  frame True {
                    n448 = for {
                      shift-right: [w1172] -> w1170
                      shift-left: w1168 -> [w1173]
                      tunnel: string[] ["CAM CLOSE", "", ""] -> [w1171] mode=indexing
                      n449 = Enqueue Element(queue=w1173, element=w1171) -> (queue out=w1172:refnum<queue>)  [unwired: 2 in, 2 out]
                    }
                  }
                }
                n450 = Or(x=w1151, y=w1156) -> (x .or. y?=w1158:bool)
                n451 = Select(t=State_Type_Definitions,_for_0.26g_versions_and_later_2."True Stop" ("Enum"), s=w1156, f=State_Type_Definitions,_for_0.26g_versions_and_later_2."True Stop" ("Enum")) -> (s? t:f=w1153:T18)
                n452 = Select(t=w1153, s=w1158, f=State_Type_Definitions,_for_0.26g_versions_and_later_2."Task 5D" ("Enum")) -> (s? t:f=w1157:T18)
              }
              frame "Exit" {
                n453 = for {
                  shift-right: [w1180] -> w1177
                  shift-left: w1174 -> [w1181]
                  tunnel: string[] ["STOP", "RESET ENCODERS", "RESET YAW", "ARDUINO MODE 0"] -> [w1179] mode=indexing
                  n454 = Enqueue Element(queue=w1181, element=w1179) -> (queue out=w1180:refnum<queue>)  [unwired: 2 in, 2 out]
                }
              }
            }
          }
          frame "Task 5E: POSITION ARM" {
            # ">>> yStepper command>>>"
            n455 = Dequeue Element(queue=w1195, timeout in ms (-1)=w1196, error in (no error)=w1197) -> (element=w1199:T10)  [unwired: 3 out]
            n456 = formula code="if (pos < 100)\ny = 41;\n\nelse if (pos >= 100 && pos <= 140)\ny = 30;\n\nelse if (pos >= 141 && pos <= 170)\ny = 25;\n\nelse if (pos >= 171 &&pos <= 180) \ny = 20;\n\nelse if (pos >= 181&& pos <= 200)\ny = 15;\n\nelse if (pos >= 201 && pos <= 230)\ny = 10;\n\nelse if (pos >= 231 && pos <= 320)\ny = 8;\n\nelse if (pos > 320)\ny = 0;"("pos"=w1187) -> ("y"=w1190:dbl)
            n457 = To Unsigned Byte Integer(number=w1190) -> (unsigned 8bit integer=w1185:u8)
            n458 = Equal?(x=w1186, y=w1185) -> (x = y?=w1184:bool)
            n459 = case shown="\"Start Task 1\", Default" w1199 {
              tunnel: [w1206 State_Type_Definitions,_for_0.26g_versions_and_later_2."True Stop" ("Enum")] -> w1193
              tunnel: [w1209 w1226] -> w1191
              tunnel: [State_Type_Definitions,_for_0.26g_versions_and_later_2."Idle" ("Enum") State_Type_Definitions,_for_0.26g_versions_and_later_2."Shutdown" ("Enum")] -> w1192
              tunnel: w1198 -> [w1205 _]
              tunnel: w1194 -> [w1201 w1223]
              tunnel: w1184 -> [w1200 _]
              frame "Start Task 1", Default {
                # ">> T: Breaks out of state loop; F: Stays in loop>>"
                # ">> Manual override >>"
                # ">> Checks if time is up>>"
                # "Stays in Task 5D until the object is detected"
                # "T: Go back to idle, F: Continue with task\""
                # ">> Manual override >>"
                n460 = case shown="False" w1200 {
                  tunnel: [w1213 w1219] -> w1209
                  tunnel: w1201 -> [w1211 w1217]
                  frame False {
                    n461 = for {
                      tunnel: string[] ["READ STEPPER VALUES", "Y STEPPER CONTROL", ""] ("element") -> [w1214] mode=indexing
                      shift-right: [w1216] -> w1213
                      shift-left: w1211 -> [w1215]
                      n462 = Enqueue Element(queue=w1215, element=w1214) -> (queue out=w1216:refnum<queue>)  [unwired: 2 in, 2 out]
                    }
                  }
                  frame True {
                    n463 = for {
                      shift-right: [w1221] -> w1219
                      shift-left: w1217 -> [w1222]
                      tunnel: string[] ["CAM CLOSE", "DISPOSE BUFFERS", ""] -> [w1220] mode=indexing
                      n464 = Enqueue Element(queue=w1222, element=w1220) -> (queue out=w1221:refnum<queue>)  [unwired: 2 in, 2 out]
                    }
                  }
                }
                n465 = Or(x=w1200, y=w1205) -> (x .or. y?=w1207:bool)
                n466 = Select(t=State_Type_Definitions,_for_0.26g_versions_and_later_2."True Stop" ("Enum"), s=w1205, f=State_Type_Definitions,_for_0.26g_versions_and_later_2."Task 5F: ARM GRAB HEIGHT" ("Enum")) -> (s? t:f=w1202:T18)
                n467 = Select(t=w1202, s=w1207, f=State_Type_Definitions,_for_0.26g_versions_and_later_2."Task 5E: POSITION ARM" ("Enum")) -> (s? t:f=w1206:T18)
              }
              frame "Exit" {
                n468 = for {
                  shift-right: [w1229] -> w1226
                  shift-left: w1223 -> [w1230]
                  tunnel: string[] ["STOP", "RESET ENCODERS", "RESET YAW", "ARDUINO MODE 0"] -> [w1228] mode=indexing
                  n469 = Enqueue Element(queue=w1230, element=w1228) -> (queue out=w1229:refnum<queue>)  [unwired: 2 in, 2 out]
                }
              }
            }
            n470 = Bundle By Name(cluster=w1189, "yStepper desired"=w1185) -> (w1188:T20)
          }
          frame "Task 5F: ARM GRAB HEIGHT" {
            # ">>> Motor control cluster >>>"
            # ">>> yStepper command>>>"
            # ">> Manual override >>"
            n471 = Dequeue Element(queue=w1241, timeout in ms (-1)=w1240, error in (no error)=w1242) -> (element=w1239:T10)  [unwired: 3 out]
            n472 = Equal?(x=w1238, y=u8 1) -> (x = y?=w1236:bool)
            n473 = case shown="\"Start Task 1\", Default" w1239 {
              tunnel: [w1252 State_Type_Definitions,_for_0.26g_versions_and_later_2."True Stop" ("Enum")] -> w1243
              tunnel: [w1255 w1272] -> w1244
              tunnel: [State_Type_Definitions,_for_0.26g_versions_and_later_2."Idle" ("Enum") State_Type_Definitions,_for_0.26g_versions_and_later_2."Shutdown" ("Enum")] -> w1245
              tunnel: w1236 -> [w1251 _]
              tunnel: w1235 -> [w1250 _]
              tunnel: w1234 -> [w1246 w1269]
              frame "Start Task 1", Default {
                # "Stays in Task 5F until stepper reaches desired \nheight"
                # "T: Go back to idle, F: Continue with task\""
                # ">> Manual override >>"
                n474 = case shown="True" w1251 {
                  tunnel: [w1259 w1265] -> w1255
                  tunnel: w1246 -> [w1257 w1263]
                  frame False {
                    n475 = for {
                      tunnel: string[] ["Z STEPPER GRAB HEIGHT", "READ STEPPER VALUES"] ("element") -> [w1260] mode=indexing
                      shift-right: [w1262] -> w1259
                      shift-left: w1257 -> [w1261]
                      n476 = Enqueue Element(queue=w1261, element=w1260) -> (queue out=w1262:refnum<queue>)  [unwired: 2 in, 2 out]
                    }
                  }
                  frame True {
                    n477 = for {
                      shift-right: [w1267] -> w1265
                      shift-left: w1263 -> [w1268]
                      tunnel: string[] ["SET TIMER 5", "CLOSE CLAW", ""] -> [w1266] mode=indexing
                      n478 = Enqueue Element(queue=w1268, element=w1266) -> (queue out=w1267:refnum<queue>)  [unwired: 2 in, 2 out]
                    }
                  }
                }
                n479 = Or(x=w1251, y=w1250) -> (x .or. y?=w1253:bool)
                n480 = Select(t=State_Type_Definitions,_for_0.26g_versions_and_later_2."True Stop" ("Enum"), s=w1250, f=State_Type_Definitions,_for_0.26g_versions_and_later_2."Task 5G: CLOSE CLAW" ("Enum")) -> (s? t:f=w1247:T18)
                n481 = Select(t=w1247, s=w1253, f=State_Type_Definitions,_for_0.26g_versions_and_later_2."Task 5F: ARM GRAB HEIGHT" ("Enum")) -> (s? t:f=w1252:T18)
              }
              frame "Exit" {
                n482 = for {
                  shift-right: [w1275] -> w1272
                  shift-left: w1269 -> [w1276]
                  tunnel: string[] ["STOP", "RESET ENCODERS", "RESET YAW", "ARDUINO MODE 0"] -> [w1274] mode=indexing
                  n483 = Enqueue Element(queue=w1276, element=w1274) -> (queue out=w1275:refnum<queue>)  [unwired: 2 in, 2 out]
                }
              }
            }
          }
          frame "Task 5G: CLOSE CLAW" {
            # ">>> yStepper command>>>"
            # ">> Manual override >>"
            n484 = Dequeue Element(queue=w1287, timeout in ms (-1)=w1286, error in (no error)=w1285) -> (element=w1284:T10)  [unwired: 3 out]
            n485 = case shown="\"Start Task 1\", Default" w1284 {
              tunnel: [w1296 State_Type_Definitions,_for_0.26g_versions_and_later_2."True Stop" ("Enum")] -> w1289
              tunnel: [w1299 w1316] -> w1282
              tunnel: [State_Type_Definitions,_for_0.26g_versions_and_later_2."Idle" ("Enum") State_Type_Definitions,_for_0.26g_versions_and_later_2."Shutdown" ("Enum")] -> w1281
              tunnel: w1283 -> [w1290 _]
              tunnel: w1288 -> [w1295 w1313]
              tunnel: w1279 -> [w1294 _]
              frame "Start Task 1", Default {
                # ">> Is time up? >>"
                # "Determines if object is in range to pick up"
                # ">> Manual override >>"
                n486 = case shown="True" w1294 {
                  tunnel: [w1303 w1309] -> w1299
                  tunnel: w1295 -> [w1301 w1307]
                  frame False {
                    n487 = for {
                      tunnel: string[] ["CLOSE CLAW", "START TIMER"] ("element") -> [w1304] mode=indexing
                      shift-right: [w1306] -> w1303
                      shift-left: w1301 -> [w1305]
                      n488 = Enqueue Element(queue=w1305, element=w1304) -> (queue out=w1306:refnum<queue>)  [unwired: 2 in, 2 out]
                    }
                  }
                  frame True {
                    n489 = for {
                      shift-right: [w1311] -> w1309
                      shift-left: w1307 -> [w1312]
                      tunnel: string[] ["READ STEPPER VALUES", "", ""] -> [w1310] mode=indexing
                      n490 = Enqueue Element(queue=w1312, element=w1310) -> (queue out=w1311:refnum<queue>)  [unwired: 2 in, 2 out]
                    }
                  }
                }
                n491 = Or(x=w1294, y=w1290) -> (x .or. y?=w1297:bool)
                n492 = Select(t=State_Type_Definitions,_for_0.26g_versions_and_later_2."True Stop" ("Enum"), s=w1290, f=State_Type_Definitions,_for_0.26g_versions_and_later_2."Task 5H: RAISE ARM" ("Enum")) -> (s? t:f=w1292:T18)
                n493 = Select(t=w1292, s=w1297, f=State_Type_Definitions,_for_0.26g_versions_and_later_2."Task 5G: CLOSE CLAW" ("Enum")) -> (s? t:f=w1296:T18)
              }
              frame "Exit" {
                n494 = for {
                  shift-right: [w1319] -> w1316
                  shift-left: w1313 -> [w1320]
                  tunnel: string[] ["STOP", "RESET ENCODERS", "RESET YAW", "ARDUINO MODE 0"] -> [w1318] mode=indexing
                  n495 = Enqueue Element(queue=w1320, element=w1318) -> (queue out=w1319:refnum<queue>)  [unwired: 2 in, 2 out]
                }
              }
            }
          }
          frame "Task 5H: RAISE ARM" {
            # ">>> yStepper command>>>"
            # ">> Manual override >>"
            n496 = Dequeue Element(queue=w1331, timeout in ms (-1)=w1330, error in (no error)=w1332) -> (element=w1329:T10)  [unwired: 3 out]
            n497 = Equal?(x=w1328, y=u8 60) -> (x = y?=w1326:bool)
            n498 = case shown="\"Start Task 1\", Default" w1329 {
              tunnel: [w1342 State_Type_Definitions,_for_0.26g_versions_and_later_2."True Stop" ("Enum")] -> w1333
              tunnel: [w1345 w1362] -> w1334
              tunnel: [State_Type_Definitions,_for_0.26g_versions_and_later_2."Idle" ("Enum") State_Type_Definitions,_for_0.26g_versions_and_later_2."Shutdown" ("Enum")] -> w1335
              tunnel: w1326 -> [w1341 _]
              tunnel: w1325 -> [w1340 _]
              tunnel: w1324 -> [w1336 w1359]
              frame "Start Task 1", Default {
                # "Stays in Task 5_A until stepper reaches desired \nheight"
                # "T: Go back to idle, F: Continue with task\""
                # ">> Manual override >>"
                n499 = case shown="False" w1341 {
                  tunnel: [w1349 w1355] -> w1345
                  tunnel: w1336 -> [w1347 w1353]
                  frame False {
                    n500 = for {
                      tunnel: string[] ["Z STEPPER CAM HEIGHT", "READ STEPPER VALUES"] ("element") -> [w1350] mode=indexing
                      shift-right: [w1352] -> w1349
                      shift-left: w1347 -> [w1351]
                      n501 = Enqueue Element(queue=w1351, element=w1350) -> (queue out=w1352:refnum<queue>)  [unwired: 2 in, 2 out]
                    }
                  }
                  frame True {
                    n502 = for {
                      shift-right: [w1357] -> w1355
                      shift-left: w1353 -> [w1358]
                      tunnel: string[] ["ARDUINO - ULTRASONIC", "READ ULTRASONIC", ""] -> [w1356] mode=indexing
                      n503 = Enqueue Element(queue=w1358, element=w1356) -> (queue out=w1357:refnum<queue>)  [unwired: 2 in, 2 out]
                    }
                  }
                }
                n504 = Or(x=w1341, y=w1340) -> (x .or. y?=w1343:bool)
                n505 = Select(t=State_Type_Definitions,_for_0.26g_versions_and_later_2."True Stop" ("Enum"), s=w1340, f=State_Type_Definitions,_for_0.26g_versions_and_later_2."True Stop" ("Enum")) -> (s? t:f=w1337:T18)
                n506 = Select(t=w1337, s=w1343, f=State_Type_Definitions,_for_0.26g_versions_and_later_2."Task 5H: RAISE ARM" ("Enum")) -> (s? t:f=w1342:T18)
              }
              frame "Exit" {
                n507 = for {
                  shift-right: [w1365] -> w1362
                  shift-left: w1359 -> [w1366]
                  tunnel: string[] ["STOP", "RESET ENCODERS", "RESET YAW", "ARDUINO MODE 0"] -> [w1364] mode=indexing
                  n508 = Enqueue Element(queue=w1366, element=w1364) -> (queue out=w1365:refnum<queue>)  [unwired: 2 in, 2 out]
                }
              }
            }
          }
          frame "Task 6_A" {
            # ">>> yStepper command>>>"
            n509 = Dequeue Element(queue=w1376, timeout in ms (-1)=w1375, error in (no error)=w1374) -> (element=w1381:T10)  [unwired: 3 out]
            n510 = Equal?(x=w1372, y=u8 60) -> (x = y?=w1371:bool)
            n511 = case shown="\"Start Task 1\", Default" w1381 {
              tunnel: [w1388 State_Type_Definitions,_for_0.26g_versions_and_later_2."True Stop" ("Enum")] -> w1379
              tunnel: [w1387 w1405] -> w1378
              tunnel: [State_Type_Definitions,_for_0.26g_versions_and_later_2."Idle" ("Enum") State_Type_Definitions,_for_0.26g_versions_and_later_2."Shutdown" ("Enum")] -> w1380
              tunnel: w1377 -> [w1383 _]
              tunnel: w1373 -> [w1385 _]
              tunnel: w1371 -> [w1382 _]
              frame "Start Task 1", Default {
                n512 = case shown="False" w1382 {
                  tunnel: [w1393 w1399] -> w1387
                  tunnel: w1385 -> [w1391 w1397]
                  frame False {
                    n513 = for {
                      tunnel: string[] ["Z STEPPER CAM HEIGHT", "READ STEPPER VALUES"] ("element") -> [w1394] mode=indexing
                      shift-right: [w1396] -> w1393
                      shift-left: w1391 -> [w1395]
                      n514 = Enqueue Element(queue=w1395, element=w1394) -> (queue out=w1396:refnum<queue>)  [unwired: 2 in, 2 out]
                    }
                  }
                  frame True {
                    n515 = for {
                      shift-right: [w1401] -> w1399
                      shift-left: w1397 -> [w1402]
                      tunnel: string[] ["CAM ACQ", "OPEN LOG CAM"] -> [w1400] mode=indexing
                      n516 = Enqueue Element(queue=w1402, element=w1400) -> (queue out=w1401:refnum<queue>)  [unwired: 2 in, 2 out]
                    }
                  }
                }
                n517 = Or(x=w1382, y=w1383) -> (x .or. y?=w1384:bool)
                n518 = Select(t=State_Type_Definitions,_for_0.26g_versions_and_later_2."Task 6_B" ("Enum"), s=w1384, f=State_Type_Definitions,_for_0.26g_versions_and_later_2."Task 6_A" ("Enum")) -> (s? t:f=w1388:T18)
              }
              frame "Exit" {
                n519 = for {
                  shift-right: [w1408] -> w1405
                  shift-left: _ -> [w1409]
                  tunnel: string[] ["STOP", "RESET ENCODERS", "RESET YAW", "ARDUINO MODE 0"] -> [w1407] mode=indexing
                  n520 = Enqueue Element(queue=w1409, element=w1407) -> (queue out=w1408:refnum<queue>)  [unwired: 2 in, 2 out]
                }
              }
            }
          }
          frame "Task 6_B" {
            # ">>> yStepper command>>>"
            n521 = Dequeue Element(queue=w1421, timeout in ms (-1)=w1419, error in (no error)=w1420) -> (element=w1418:T10)  [unwired: 3 out]
            n522 = case shown="\"Start Task 1\", Default" w1418 {
              tunnel: [w1428 State_Type_Definitions,_for_0.26g_versions_and_later_2."True Stop" ("Enum")] -> w1414
              tunnel: [w1427 w1446] -> w1422
              tunnel: [State_Type_Definitions,_for_0.26g_versions_and_later_2."Idle" ("Enum") State_Type_Definitions,_for_0.26g_versions_and_later_2."Shutdown" ("Enum")] -> w1415
              tunnel: w1417 -> [w1423 _]
              tunnel: w1416 -> [w1425 _]
              tunnel: w1413 -> [w1424 w1443]
              frame "Start Task 1", Default {
                # ">> Manual override >>"
                n523 = case shown="False" w1425 {
                  tunnel: [w1433 w1439] -> w1427
                  tunnel: w1424 -> [w1432 w1437]
                  frame False {
                    n524 = for {
                      shift-right: [w1436] -> w1433
                      shift-left: w1432 -> [w1435]
                      tunnel: string[] ["CAM ACQ", "PROCESS IMAGE", "OPEN CLAW"] -> [w1434] mode=indexing
                      n525 = Enqueue Element(queue=w1435, element=w1434) -> (queue out=w1436:refnum<queue>)  [unwired: 2 in, 2 out]
                    }
                  }
                  frame True {
                    n526 = for {
                      shift-right: [w1441] -> w1439
                      shift-left: w1437 -> [w1442]
                      tunnel: string[] ["CAM ACQ", "PROCESS IMAGE", "CLOSE CLAW"] -> [w1440] mode=indexing
                      n527 = Enqueue Element(queue=w1442, element=w1440) -> (queue out=w1441:refnum<queue>)  [unwired: 2 in, 2 out]
                    }
                  }
                }
                n528 = Select(t=State_Type_Definitions,_for_0.26g_versions_and_later_2."True Stop" ("Enum"), s=w1423, f=State_Type_Definitions,_for_0.26g_versions_and_later_2."Task 6_B" ("Enum")) -> (s? t:f=w1428:T18)
              }
              frame "Exit" {
                # ">> State after true stop >>"
                # ">> Goes to true stop >>"
                n529 = for {
                  shift-right: [w1449] -> w1446
                  shift-left: w1443 -> [w1450]
                  tunnel: string[] ["STOP", "RESET ENCODERS", "RESET YAW", ""] -> [w1448] mode=indexing
                  n530 = Enqueue Element(queue=w1450, element=w1448) -> (queue out=w1449:refnum<queue>)  [unwired: 2 in, 2 out]
                }
              }
            }
          }
          frame "Task 7" {
          }
          frame "Task 8A: RAISE ARM" {
            # ">>> Motor control cluster >>>"
            # ">>> yStepper command>>>"
            # ">> Manual override >>"
            n531 = Dequeue Element(queue=w1467, timeout in ms (-1)=w1466, error in (no error)=w1468) -> (element=w1465:T10)  [unwired: 3 out]
            n532 = Equal?(x=w1464, y=u8 60) -> (x = y?=w1462:bool)
            n533 = case shown="\"Start Task 1\", Default" w1465 {
              tunnel: [w1478 State_Type_Definitions,_for_0.26g_versions_and_later_2."True Stop" ("Enum")] -> w1469
              tunnel: [w1481 w1498] -> w1470
              tunnel: [State_Type_Definitions,_for_0.26g_versions_and_later_2."Idle" ("Enum") State_Type_Definitions,_for_0.26g_versions_and_later_2."Shutdown" ("Enum")] -> w1471
              tunnel: w1462 -> [w1477 _]
              tunnel: w1461 -> [w1476 _]
              tunnel: w1460 -> [w1472 w1495]
              frame "Start Task 1", Default {
                # "Stays in Task 5_A until stepper reaches desired \nheight"
                # "T: Go back to idle, F: Continue with task\""
                # ">> Manual override >>"
                n534 = case shown="False" w1477 {
                  tunnel: [w1485 w1491] -> w1481
                  tunnel: w1472 -> [w1483 w1489]
                  frame False {
                    n535 = for {
                      tunnel: string[] ["Z STEPPER CAM HEIGHT", "READ STEPPER VALUES", "READ IR"] ("element") -> [w1486] mode=indexing
                      shift-right: [w1488] -> w1485
                      shift-left: w1483 -> [w1487]
                      n536 = Enqueue Element(queue=w1487, element=w1486) -> (queue out=w1488:refnum<queue>)  [unwired: 2 in, 2 out]
                    }
                  }
                  frame True {
                    n537 = for {
                      shift-right: [w1493] -> w1491
                      shift-left: w1489 -> [w1494]
                      tunnel: string[] ["RESET YAW", "RESET ENCODERS", "READ IR"] -> [w1492] mode=indexing
                      n538 = Enqueue Element(queue=w1494, element=w1492) -> (queue out=w1493:refnum<queue>)  [unwired: 2 in, 2 out]
                    }
                  }
                }
                n539 = Or(x=w1477, y=w1476) -> (x .or. y?=w1479:bool)
                n540 = Select(t=State_Type_Definitions,_for_0.26g_versions_and_later_2."True Stop" ("Enum"), s=w1476, f=State_Type_Definitions,_for_0.26g_versions_and_later_2."Task 8B: MOVE TO BOX" ("Enum")) -> (s? t:f=w1473:T18)
                n541 = Select(t=w1473, s=w1479, f=State_Type_Definitions,_for_0.26g_versions_and_later_2."Task 8A: RAISE ARM" ("Enum")) -> (s? t:f=w1478:T18)
              }
              frame "Exit" {
                n542 = for {
                  shift-right: [w1501] -> w1498
                  shift-left: w1495 -> [w1502]
                  tunnel: string[] ["STOP", "RESET ENCODERS", "RESET YAW", "ARDUINO MODE 0"] -> [w1500] mode=indexing
                  n543 = Enqueue Element(queue=w1502, element=w1500) -> (queue out=w1501:refnum<queue>)  [unwired: 2 in, 2 out]
                }
              }
            }
          }
          frame "Task 8B: MOVE TO BOX" {
            w1512 = u8 15 ("y")
            # ">>> yStepper command>>>"
            n544 = Less?(x=w1509, y=w1512) -> (x < y?=w1510:bool)
            n545 = Less?(x=w1508, y=w1512) -> (x < y?=w1511:bool)
            n546 = And(x=w1511, y=w1510) -> ()  [unwired: 1 out]
            n547 = Dequeue Element(queue=w1516, timeout in ms (-1)=w1515, error in (no error)=w1517) -> (element=w1514:T10)  [unwired: 3 out]
            n548 = Less?(x=w1505, y=70.0) -> (x < y?=w1503:bool)
            n549 = case shown="\"Start Task 1\", Default" w1514 {
              tunnel: [w1529 State_Type_Definitions,_for_0.26g_versions_and_later_2."True Stop" ("Enum")] -> w1519
              tunnel: [w1532 w1549] -> w1518
              tunnel: [State_Type_Definitions,_for_0.26g_versions_and_later_2."Idle" ("Enum") State_Type_Definitions,_for_0.26g_versions_and_later_2."Shutdown" ("Enum")] -> w1520
              tunnel: w1522 -> [w1528 _]
              tunnel: w1521 -> [w1524 w1546]
              tunnel: w1503 -> [w1523 _]
              frame "Start Task 1", Default {
                # "Stays in Task 5_B to capture image over 5 seconds"
                # "T: Go back to idle, F: Continue with task\""
                # ">> Manual override >>"
                n550 = case shown="True" w1523 {
                  tunnel: [w1536 w1542] -> w1532
                  tunnel: w1524 -> [w1534 w1540]
                  frame False {
                    n551 = for {
                      tunnel: string[] ["FORWARD", "READ IR", "READ NAVX"] ("element") -> [w1537] mode=indexing
                      shift-right: [w1539] -> w1536
                      shift-left: w1534 -> [w1538]
                      n552 = Enqueue Element(queue=w1538, element=w1537) -> (queue out=w1539:refnum<queue>)  [unwired: 2 in, 2 out]
                    }
                  }
                  frame True {
                    n553 = for {
                      shift-right: [w1544] -> w1542
                      shift-left: w1540 -> [w1545]
                      tunnel: string[] ["STOP", "RESET ENCODERS", "OPEN LOG CAM", "SET TIMER 2", "OPEN IMAQ REF"] -> [w1543] mode=indexing
                      n554 = Enqueue Element(queue=w1545, element=w1543) -> (queue out=w1544:refnum<queue>)  [unwired: 2 in, 2 out]
                    }
                  }
                }
                n555 = Or(x=w1523, y=w1528) -> (x .or. y?=w1530:bool)
                n556 = Select(t=State_Type_Definitions,_for_0.26g_versions_and_later_2."True Stop" ("Enum"), s=w1528, f=State_Type_Definitions,_for_0.26g_versions_and_later_2."Task 8C: CAM BURST" ("Enum")) -> (s? t:f=w1525:T18)
                n557 = Select(t=w1525, s=w1530, f=State_Type_Definitions,_for_0.26g_versions_and_later_2."Task 8B: MOVE TO BOX" ("Enum")) -> (s? t:f=w1529:T18)
              }
              frame "Exit" {
                n558 = for {
                  shift-right: [w1552] -> w1549
                  shift-left: w1546 -> [w1553]
                  tunnel: string[] ["STOP", "RESET ENCODERS", "RESET YAW", "ARDUINO MODE 0"] -> [w1551] mode=indexing
                  n559 = Enqueue Element(queue=w1553, element=w1551) -> (queue out=w1552:refnum<queue>)  [unwired: 2 in, 2 out]
                }
              }
            }
          }
          frame "Task 8C: CAM BURST" {
            # ">>> Motor control cluster >>>"
            # ">>> yStepper command>>>"
            # ">> Manual override >>"
            n560 = Dequeue Element(queue=w1564, timeout in ms (-1)=w1563, error in (no error)=w1562) -> (element=w1561:T10)  [unwired: 3 out]
            n561 = case shown="\"Start Task 1\", Default" w1561 {
              tunnel: [w1573 State_Type_Definitions,_for_0.26g_versions_and_later_2."True Stop" ("Enum")] -> w1566
              tunnel: [w1576 w1593] -> w1559
              tunnel: [State_Type_Definitions,_for_0.26g_versions_and_later_2."Idle" ("Enum") State_Type_Definitions,_for_0.26g_versions_and_later_2."Shutdown" ("Enum")] -> w1558
              tunnel: w1560 -> [w1567 _]
              tunnel: w1565 -> [w1572 w1590]
              tunnel: w1556 -> [w1571 _]
              frame "Start Task 1", Default {
                # ">> Is time up? >>"
                # "Determines if object is in range to pick up"
                # ">> Manual override >>"
                n562 = case shown="True" w1571 {
                  tunnel: [w1580 w1586] -> w1576
                  tunnel: w1572 -> [w1578 w1584]
                  frame False {
                    n563 = for {
                      tunnel: string[] ["CAM ACQ", "START TIMER"] ("element") -> [w1581] mode=indexing
                      shift-right: [w1583] -> w1580
                      shift-left: w1578 -> [w1582]
                      n564 = Enqueue Element(queue=w1582, element=w1581) -> (queue out=w1583:refnum<queue>)  [unwired: 2 in, 2 out]
                    }
                  }
                  frame True {
                    n565 = for {
                      shift-right: [w1588] -> w1586
                      shift-left: w1584 -> [w1589]
                      tunnel: string[] ["CAM CLOSE", "PROCESS IMAGE", "SET TIMER 2"] -> [w1587] mode=indexing
                      n566 = Enqueue Element(queue=w1589, element=w1587) -> (queue out=w1588:refnum<queue>)  [unwired: 2 in, 2 out]
                    }
                  }
                }
                n567 = Or(x=w1571, y=w1567) -> (x .or. y?=w1574:bool)
                n568 = Select(t=State_Type_Definitions,_for_0.26g_versions_and_later_2."True Stop" ("Enum"), s=w1567, f=State_Type_Definitions,_for_0.26g_versions_and_later_2."Task 8D: PROCESS IMAGE" ("Enum")) -> (s? t:f=w1569:T18)
                n569 = Select(t=w1569, s=w1574, f=State_Type_Definitions,_for_0.26g_versions_and_later_2."Task 8C: CAM BURST" ("Enum")) -> (s? t:f=w1573:T18)
              }
              frame "Exit" {
                n570 = for {
                  shift-right: [w1596] -> w1593
                  shift-left: w1590 -> [w1597]
                  tunnel: string[] ["STOP", "RESET ENCODERS", "RESET YAW", "ARDUINO MODE 0"] -> [w1595] mode=indexing
                  n571 = Enqueue Element(queue=w1597, element=w1595) -> (queue out=w1596:refnum<queue>)  [unwired: 2 in, 2 out]
                }
              }
            }
          }
          frame "Task 8D: PROCESS IMAGE" {
            # ">>> yStepper command>>>"
            n572 = Dequeue Element(queue=w1605, timeout in ms (-1)=w1604, error in (no error)=w1603) -> (element=w1602:T10)  [unwired: 3 out]
            n573 = case shown="\"Start Task 1\", Default" w1602 {
              tunnel: [w1617 State_Type_Definitions,_for_0.26g_versions_and_later_2."True Stop" ("Enum")] -> w1609
              tunnel: [w1620 w1637] -> w1608
              tunnel: [State_Type_Definitions,_for_0.26g_versions_and_later_2."Idle" ("Enum") State_Type_Definitions,_for_0.26g_versions_and_later_2."Shutdown" ("Enum")] -> w1610
              tunnel: w1606 -> [w1616 _]
              tunnel: w1607 -> [w1612 w1634]
              tunnel: w1600 -> [w1611 _]
              frame "Start Task 1", Default {
                # ">> T: Breaks out of state loop; F: Stays in loop>>"
                # ">> Manual override >>"
                # ">> Checks if time is up>>"
                # "Stays in Task 5D until the object is detected"
                # "T: Go back to idle, F: Continue with task\""
                # ">> Manual override >>"
                n574 = case shown="False" w1611 {
                  tunnel: [w1624 w1630] -> w1620
                  tunnel: w1612 -> [w1622 w1628]
                  frame False {
                    n575 = for {
                      tunnel: string[] ["START TIMER", "PROCESS IMAGE", ""] ("element") -> [w1625] mode=indexing
                      shift-right: [w1627] -> w1624
                      shift-left: w1622 -> [w1626]
                      n576 = Enqueue Element(queue=w1626, element=w1625) -> (queue out=w1627:refnum<queue>)  [unwired: 2 in, 2 out]
                    }
                  }
                  frame True {
                    n577 = for {
                      shift-right: [w1632] -> w1630
                      shift-left: w1628 -> [w1633]
                      tunnel: string[] ["RESET ENCODERS", "", ""] -> [w1631] mode=indexing
                      n578 = Enqueue Element(queue=w1633, element=w1631) -> (queue out=w1632:refnum<queue>)  [unwired: 2 in, 2 out]
                    }
                  }
                }
                n579 = Or(x=w1611, y=w1616) -> (x .or. y?=w1618:bool)
                n580 = Select(t=State_Type_Definitions,_for_0.26g_versions_and_later_2."True Stop" ("Enum"), s=w1616, f=State_Type_Definitions,_for_0.26g_versions_and_later_2."Task 8E: ROBOT ADJUST" ("Enum")) -> (s? t:f=w1613:T18)
                n581 = Select(t=w1613, s=w1618, f=State_Type_Definitions,_for_0.26g_versions_and_later_2."Task 8D: PROCESS IMAGE" ("Enum")) -> (s? t:f=w1617:T18)
              }
              frame "Exit" {
                n582 = for {
                  shift-right: [w1640] -> w1637
                  shift-left: w1634 -> [w1641]
                  tunnel: string[] ["STOP", "RESET ENCODERS", "RESET YAW", "ARDUINO MODE 0"] -> [w1639] mode=indexing
                  n583 = Enqueue Element(queue=w1641, element=w1639) -> (queue out=w1640:refnum<queue>)  [unwired: 2 in, 2 out]
                }
              }
            }
          }
          frame "Task 8E: ROBOT ADJUST" {
            # ">>> Motor control cluster >>>"
            # ">>> yStepper command>>>"
            n584 = Dequeue Element(queue=w1658, timeout in ms (-1)=w1657, error in (no error)=w1656) -> (element=w1655:T10)  [unwired: 3 out]
            n585 = Subtract(x=w1653, y=300.0) -> (x-y=w1651:dbl)
            n586 = formula code="if (error <= -61&&error > -300){\ndistance = -15;\nxSpeed = -30;\n}\n\nelse if (error <= -51 && error >= -60){\ndistance = -10;\nxSpeed = -30;\n}\n\nelse if (error >= -50 && error <= 50){\ndistance = 0;\nxSpeed = 0;\n}\n\nelse if (error >= 51 && error <= 80){\ndistance = 10;\nxSpeed = 30;\n}\n\nelse if (error >= 81 && error <= 100){\ndistance = 15;\nxSpeed = 30;\n}\n\nelse if (error >= 101 && error <= 120){\ndistance = 20;\nxSpeed = 30;\n}\n\nelse if (error >= 121 && error < 300){\ndistance = 25;\nxSpeed = 30;\n}\n\nelse{\ndistance = 0;\nxSpeed = 0;\n}"("error"=w1651) -> ("distance"=w1646:dbl, "xSpeed"=w1648:dbl)
            n587 = formula code="if (target > 0){\nif (current  >= target)\noutput = 1;\n\nelse if (current != target)\noutput = 0;\n}\n\nelse if (target == 0){\nif (current == target)\noutput = 1;\n\nelse if (current != target)\noutput = 0;\n}\n\nelse if (target < 0){\nif (current <= target)\noutput = 1;\n\nelse if (current != target)\noutput = 0;\n}\n\nelse if (current != target)\noutput = 0;"("target"=w1646, "current"=w1647) -> ("output"=w1645:dbl)
            n588 = Bundle By Name(cluster=w1650, "xSpeed"=w1648) -> (w1649:T19)
            n589 = Equal?(x=w1645, y=1.0) -> (x = y?=w1643:bool)
            n590 = case shown="\"Start Task 1\", Default" w1655 {
              tunnel: [w1670 State_Type_Definitions,_for_0.26g_versions_and_later_2."True Stop" ("Enum")] -> w1662
              tunnel: [w1673 w1690] -> w1661
              tunnel: [State_Type_Definitions,_for_0.26g_versions_and_later_2."Idle" ("Enum") State_Type_Definitions,_for_0.26g_versions_and_later_2."Shutdown" ("Enum")] -> w1663
              tunnel: w1659 -> [w1669 _]
              tunnel: w1660 -> [w1665 w1687]
              tunnel: w1643 -> [w1664 _]
              frame "Start Task 1", Default {
                # ">> T: Breaks out of state loop; F: Stays in loop>>"
                # ">> Manual override >>"
                # ">> Checks if time is up>>"
                # "Stays in Task 5D until the object is detected"
                # "T: Go back to idle, F: Continue with task\""
                # ">> Manual override >>"
                n591 = case shown="True" w1664 {
                  tunnel: [w1677 w1683] -> w1673
                  tunnel: w1665 -> [w1675 w1681]
                  frame False {
                    n592 = for {
                      tunnel: string[] ["X AXIS - SLOW", "READ ENCODERS", "READ NAVX"] ("element") -> [w1678] mode=indexing
                      shift-right: [w1680] -> w1677
                      shift-left: w1675 -> [w1679]
                      n593 = Enqueue Element(queue=w1679, element=w1678) -> (queue out=w1680:refnum<queue>)  [unwired: 2 in, 2 out]
                    }
                  }
                  frame True {
                    n594 = for {
                      shift-right: [w1685] -> w1683
                      shift-left: w1681 -> [w1686]
                      tunnel: string[] ["SET TIMER 2", "STOP", "READ STEPPER VALUES", ""] -> [w1684] mode=indexing
                      n595 = Enqueue Element(queue=w1686, element=w1684) -> (queue out=w1685:refnum<queue>)  [unwired: 2 in, 2 out]
                    }
                  }
                }
                n596 = Or(x=w1664, y=w1669) -> (x .or. y?=w1671:bool)
                n597 = Select(t=State_Type_Definitions,_for_0.26g_versions_and_later_2."True Stop" ("Enum"), s=w1669, f=State_Type_Definitions,_for_0.26g_versions_and_later_2."Task 8H: ARM ADJUST" ("Enum")) -> (s? t:f=w1666:T18)
                n598 = Select(t=w1666, s=w1671, f=State_Type_Definitions,_for_0.26g_versions_and_later_2."Task 8E: ROBOT ADJUST" ("Enum")) -> (s? t:f=w1670:T18)
              }
              frame "Exit" {
                n599 = for {
                  shift-right: [w1693] -> w1690
                  shift-left: w1687 -> [w1694]
                  tunnel: string[] ["STOP", "RESET ENCODERS", "RESET YAW", "ARDUINO MODE 0"] -> [w1692] mode=indexing
                  n600 = Enqueue Element(queue=w1694, element=w1692) -> (queue out=w1693:refnum<queue>)  [unwired: 2 in, 2 out]
                }
              }
            }
          }
          frame "Task 8F: CAM BURST 2" {
            # ">>> Motor control cluster >>>"
            # ">>> yStepper command>>>"
            # ">> Manual override >>"
            n601 = Dequeue Element(queue=w1705, timeout in ms (-1)=w1704, error in (no error)=w1703) -> (element=w1702:T10)  [unwired: 3 out]
            n602 = case shown="\"Start Task 1\", Default" w1702 {
              tunnel: [w1714 State_Type_Definitions,_for_0.26g_versions_and_later_2."True Stop" ("Enum")] -> w1707
              tunnel: [w1717 w1734] -> w1700
              tunnel: [State_Type_Definitions,_for_0.26g_versions_and_later_2."Idle" ("Enum") State_Type_Definitions,_for_0.26g_versions_and_later_2."Shutdown" ("Enum")] -> w1699
              tunnel: w1701 -> [w1708 _]
              tunnel: w1706 -> [w1713 w1731]
              tunnel: w1697 -> [w1712 _]
              frame "Start Task 1", Default {
                # ">> Is time up? >>"
                # "Determines if object is in range to pick up"
                # ">> Manual override >>"
                n603 = case shown="False" w1712 {
                  tunnel: [w1721 w1727] -> w1717
                  tunnel: w1713 -> [w1719 w1725]
                  frame False {
                    n604 = for {
                      tunnel: string[] ["CAM ACQ", "START TIMER"] ("element") -> [w1722] mode=indexing
                      shift-right: [w1724] -> w1721
                      shift-left: w1719 -> [w1723]
                      n605 = Enqueue Element(queue=w1723, element=w1722) -> (queue out=w1724:refnum<queue>)  [unwired: 2 in, 2 out]
                    }
                  }
                  frame True {
                    n606 = for {
                      shift-right: [w1729] -> w1727
                      shift-left: w1725 -> [w1730]
                      tunnel: string[] ["CAM CLOSE", "PROCESS IMAGE", "SET TIMER 3"] -> [w1728] mode=indexing
                      n607 = Enqueue Element(queue=w1730, element=w1728) -> (queue out=w1729:refnum<queue>)  [unwired: 2 in, 2 out]
                    }
                  }
                }
                n608 = Or(x=w1712, y=w1708) -> (x .or. y?=w1715:bool)
                n609 = Select(t=State_Type_Definitions,_for_0.26g_versions_and_later_2."True Stop" ("Enum"), s=w1708, f=State_Type_Definitions,_for_0.26g_versions_and_later_2."Task 8G: PROCESS IMAGE 2" ("Enum")) -> (s? t:f=w1710:T18)
                n610 = Select(t=w1710, s=w1715, f=State_Type_Definitions,_for_0.26g_versions_and_later_2."Task 8F: CAM BURST 2" ("Enum")) -> (s? t:f=w1714:T18)
              }
              frame "Exit" {
                n611 = for {
                  shift-right: [w1737] -> w1734
                  shift-left: w1731 -> [w1738]
                  tunnel: string[] ["STOP", "RESET ENCODERS", "RESET YAW", "ARDUINO MODE 0"] -> [w1736] mode=indexing
                  n612 = Enqueue Element(queue=w1738, element=w1736) -> (queue out=w1737:refnum<queue>)  [unwired: 2 in, 2 out]
                }
              }
            }
          }
          frame "Task 8G: PROCESS IMAGE 2" {
            # ">>> yStepper command>>>"
            n613 = Dequeue Element(queue=w1746, timeout in ms (-1)=w1745, error in (no error)=w1744) -> (element=w1743:T10)  [unwired: 3 out]
            n614 = case shown="\"Start Task 1\", Default" w1743 {
              tunnel: [w1758 State_Type_Definitions,_for_0.26g_versions_and_later_2."True Stop" ("Enum")] -> w1750
              tunnel: [w1761 w1778] -> w1749
              tunnel: [State_Type_Definitions,_for_0.26g_versions_and_later_2."Idle" ("Enum") State_Type_Definitions,_for_0.26g_versions_and_later_2."Shutdown" ("Enum")] -> w1751
              tunnel: w1747 -> [w1757 _]
              tunnel: w1748 -> [w1753 w1775]
              tunnel: w1741 -> [w1752 _]
              frame "Start Task 1", Default {
                # ">> T: Breaks out of state loop; F: Stays in loop>>"
                # ">> Manual override >>"
                # ">> Checks if time is up>>"
                # "Stays in Task 5D until the object is detected"
                # "T: Go back to idle, F: Continue with task\""
                # ">> Manual override >>"
                n615 = case shown="False" w1752 {
                  tunnel: [w1765 w1771] -> w1761
                  tunnel: w1753 -> [w1763 w1769]
                  frame False {
                    n616 = for {
                      tunnel: string[] ["START TIMER", "PROCESS IMAGE", ""] ("element") -> [w1766] mode=indexing
                      shift-right: [w1768] -> w1765
                      shift-left: w1763 -> [w1767]
                      n617 = Enqueue Element(queue=w1767, element=w1766) -> (queue out=w1768:refnum<queue>)  [unwired: 2 in, 2 out]
                    }
                  }
                  frame True {
                    n618 = for {
                      shift-right: [w1773] -> w1771
                      shift-left: w1769 -> [w1774]
                      tunnel: string[] ["READ STEPPER VALUES", "Y STEPPER CONTROL", ""] -> [w1772] mode=indexing
                      n619 = Enqueue Element(queue=w1774, element=w1772) -> (queue out=w1773:refnum<queue>)  [unwired: 2 in, 2 out]
                    }
                  }
                }
                n620 = Or(x=w1752, y=w1757) -> (x .or. y?=w1759:bool)
                n621 = Select(t=State_Type_Definitions,_for_0.26g_versions_and_later_2."True Stop" ("Enum"), s=w1757, f=State_Type_Definitions,_for_0.26g_versions_and_later_2."Task 8H: ARM ADJUST" ("Enum")) -> (s? t:f=w1754:T18)
                n622 = Select(t=w1754, s=w1759, f=State_Type_Definitions,_for_0.26g_versions_and_later_2."Task 8G: PROCESS IMAGE 2" ("Enum")) -> (s? t:f=w1758:T18)
              }
              frame "Exit" {
                n623 = for {
                  shift-right: [w1781] -> w1778
                  shift-left: w1775 -> [w1782]
                  tunnel: string[] ["STOP", "RESET ENCODERS", "RESET YAW", "ARDUINO MODE 0"] -> [w1780] mode=indexing
                  n624 = Enqueue Element(queue=w1782, element=w1780) -> (queue out=w1781:refnum<queue>)  [unwired: 2 in, 2 out]
                }
              }
            }
          }
          frame "Task 8H: ARM ADJUST" {
            # ">>> yStepper command>>>"
            n625 = Dequeue Element(queue=w1796, timeout in ms (-1)=w1797, error in (no error)=w1798) -> (element=w1800:T10)  [unwired: 3 out]
            n626 = formula code="if (pos < 70)\ny = 43;\n\nelse if (pos >= 71 &&pos <= 80)\ny = 40;\n\nelse if (pos >= 81 && pos <= 90)\ny = 38;\n\nelse if (pos >= 91 &&pos <= 120)\ny = 35;\n\nelse if (pos >= 121 && pos <= 140)\ny = 30;\n\nelse if (pos >= 141 && pos <= 170)\ny = 26;\n\nelse if (pos >= 171 &&pos <= 220) \ny = 20;\n\nelse if (pos >= 221&& pos <= 240)\ny = 15;\n\nelse if (pos >= 241 && pos <= 250)\ny = 10;\n\nelse if (pos >= 251)\ny = 0;"("pos"=w1788) -> ("y"=w1791:dbl)
            n627 = To Unsigned Byte Integer(number=w1791) -> (unsigned 8bit integer=w1786:u8)
            n628 = Equal?(x=w1787, y=w1786) -> (x = y?=w1785:bool)
            n629 = case shown="\"Start Task 1\", Default" w1800 {
              tunnel: [w1807 State_Type_Definitions,_for_0.26g_versions_and_later_2."True Stop" ("Enum")] -> w1794
              tunnel: [w1810 w1827] -> w1792
              tunnel: [State_Type_Definitions,_for_0.26g_versions_and_later_2."Idle" ("Enum") State_Type_Definitions,_for_0.26g_versions_and_later_2."Shutdown" ("Enum")] -> w1793
              tunnel: w1799 -> [w1806 _]
              tunnel: w1795 -> [w1802 w1824]
              tunnel: w1785 -> [w1801 _]
              frame "Start Task 1", Default {
                # ">> T: Breaks out of state loop; F: Stays in loop>>"
                # ">> Manual override >>"
                # ">> Checks if time is up>>"
                # "Stays in Task 5D until the object is detected"
                # "T: Go back to idle, F: Continue with task\""
                # ">> Manual override >>"
                n630 = case shown="False" w1801 {
                  tunnel: [w1814 w1820] -> w1810
                  tunnel: w1802 -> [w1812 w1818]
                  frame False {
                    n631 = for {
                      tunnel: string[] ["READ STEPPER VALUES", "Y STEPPER CONTROL", ""] ("element") -> [w1815] mode=indexing
                      shift-right: [w1817] -> w1814
                      shift-left: w1812 -> [w1816]
                      n632 = Enqueue Element(queue=w1816, element=w1815) -> (queue out=w1817:refnum<queue>)  [unwired: 2 in, 2 out]
                    }
                  }
                  frame True {
                    n633 = for {
                      shift-right: [w1822] -> w1820
                      shift-left: w1818 -> [w1823]
                      tunnel: string[] ["DISPOSE BUFFERS", "READ STEPPER VALUES", ""] -> [w1821] mode=indexing
                      n634 = Enqueue Element(queue=w1823, element=w1821) -> (queue out=w1822:refnum<queue>)  [unwired: 2 in, 2 out]
                    }
                  }
                }
                n635 = Or(x=w1801, y=w1806) -> (x .or. y?=w1808:bool)
                n636 = Select(t=State_Type_Definitions,_for_0.26g_versions_and_later_2."True Stop" ("Enum"), s=w1806, f=State_Type_Definitions,_for_0.26g_versions_and_later_2."Task 8I: ARM GRAB HEIGHT" ("Enum")) -> (s? t:f=w1803:T18)
                n637 = Select(t=w1803, s=w1808, f=State_Type_Definitions,_for_0.26g_versions_and_later_2."Task 8H: ARM ADJUST" ("Enum")) -> (s? t:f=w1807:T18)
              }
              frame "Exit" {
                n638 = for {
                  shift-right: [w1830] -> w1827
                  shift-left: w1824 -> [w1831]
                  tunnel: string[] ["STOP", "RESET ENCODERS", "RESET YAW", "ARDUINO MODE 0"] -> [w1829] mode=indexing
                  n639 = Enqueue Element(queue=w1831, element=w1829) -> (queue out=w1830:refnum<queue>)  [unwired: 2 in, 2 out]
                }
              }
            }
            n640 = Bundle By Name(cluster=w1790, "yStepper desired"=w1786) -> (w1789:T20)
          }
          frame "Task 8I: ARM GRAB HEIGHT" {
            # ">>> Motor control cluster >>>"
            # ">>> yStepper command>>>"
            # ">> Manual override >>"
            n641 = Dequeue Element(queue=w1842, timeout in ms (-1)=w1841, error in (no error)=w1843) -> (element=w1840:T10)  [unwired: 3 out]
            n642 = Equal?(x=w1839, y=u8 1) -> (x = y?=w1837:bool)
            n643 = case shown="\"Start Task 1\", Default" w1840 {
              tunnel: [w1853 State_Type_Definitions,_for_0.26g_versions_and_later_2."True Stop" ("Enum")] -> w1844
              tunnel: [w1856 w1873] -> w1845
              tunnel: [State_Type_Definitions,_for_0.26g_versions_and_later_2."Idle" ("Enum") State_Type_Definitions,_for_0.26g_versions_and_later_2."Shutdown" ("Enum")] -> w1846
              tunnel: w1837 -> [w1852 _]
              tunnel: w1836 -> [w1851 _]
              tunnel: w1835 -> [w1847 w1870]
              frame "Start Task 1", Default {
                # "Stays in Task 5F until stepper reaches desired \nheight"
                # "T: Go back to idle, F: Continue with task\""
                # ">> Manual override >>"
                n644 = case shown="True" w1852 {
                  tunnel: [w1860 w1866] -> w1856
                  tunnel: w1847 -> [w1858 w1864]
                  frame False {
                    n645 = for {
                      tunnel: string[] ["Z STEPPER GRAB HEIGHT", "READ STEPPER VALUES"] ("element") -> [w1861] mode=indexing
                      shift-right: [w1863] -> w1860
                      shift-left: w1858 -> [w1862]
                      n646 = Enqueue Element(queue=w1862, element=w1861) -> (queue out=w1863:refnum<queue>)  [unwired: 2 in, 2 out]
                    }
                  }
                  frame True {
                    n647 = for {
                      shift-right: [w1868] -> w1866
                      shift-left: w1864 -> [w1869]
                      tunnel: string[] ["SET TIMER 2", "CLOSE CLAW", ""] -> [w1867] mode=indexing
                      n648 = Enqueue Element(queue=w1869, element=w1867) -> (queue out=w1868:refnum<queue>)  [unwired: 2 in, 2 out]
                    }
                  }
                }
                n649 = Or(x=w1852, y=w1851) -> (x .or. y?=w1854:bool)
                n650 = Select(t=State_Type_Definitions,_for_0.26g_versions_and_later_2."True Stop" ("Enum"), s=w1851, f=State_Type_Definitions,_for_0.26g_versions_and_later_2."Task 8J: CLOSE CLAW" ("Enum")) -> (s? t:f=w1848:T18)
                n651 = Select(t=w1848, s=w1854, f=State_Type_Definitions,_for_0.26g_versions_and_later_2."Task 8I: ARM GRAB HEIGHT" ("Enum")) -> (s? t:f=w1853:T18)
              }
              frame "Exit" {
                n652 = for {
                  shift-right: [w1876] -> w1873
                  shift-left: w1870 -> [w1877]
                  tunnel: string[] ["STOP", "RESET ENCODERS", "RESET YAW", "ARDUINO MODE 0"] -> [w1875] mode=indexing
                  n653 = Enqueue Element(queue=w1877, element=w1875) -> (queue out=w1876:refnum<queue>)  [unwired: 2 in, 2 out]
                }
              }
            }
          }
          frame "Task 8J: CLOSE CLAW" {
            # ">>> yStepper command>>>"
            # ">> Manual override >>"
            n654 = Dequeue Element(queue=w1888, timeout in ms (-1)=w1887, error in (no error)=w1886) -> (element=w1885:T10)  [unwired: 3 out]
            n655 = case shown="\"Start Task 1\", Default" w1885 {
              tunnel: [w1897 State_Type_Definitions,_for_0.26g_versions_and_later_2."True Stop" ("Enum")] -> w1890
              tunnel: [w1900 w1917] -> w1883
              tunnel: [State_Type_Definitions,_for_0.26g_versions_and_later_2."Idle" ("Enum") State_Type_Definitions,_for_0.26g_versions_and_later_2."Shutdown" ("Enum")] -> w1882
              tunnel: w1884 -> [w1891 _]
              tunnel: w1889 -> [w1896 w1914]
              tunnel: w1880 -> [w1895 _]
              frame "Start Task 1", Default {
                # ">> Is time up? >>"
                # "Determines if object is in range to pick up"
                # ">> Manual override >>"
                n656 = case shown="True" w1895 {
                  tunnel: [w1904 w1910] -> w1900
                  tunnel: w1896 -> [w1902 w1908]
                  frame False {
                    n657 = for {
                      tunnel: string[] ["CLOSE CLAW", "START TIMER"] ("element") -> [w1905] mode=indexing
                      shift-right: [w1907] -> w1904
                      shift-left: w1902 -> [w1906]
                      n658 = Enqueue Element(queue=w1906, element=w1905) -> (queue out=w1907:refnum<queue>)  [unwired: 2 in, 2 out]
                    }
                  }
                  frame True {
                    n659 = for {
                      shift-right: [w1912] -> w1910
                      shift-left: w1908 -> [w1913]
                      tunnel: string[] ["READ STEPPER VALUES", "", ""] -> [w1911] mode=indexing
                      n660 = Enqueue Element(queue=w1913, element=w1911) -> (queue out=w1912:refnum<queue>)  [unwired: 2 in, 2 out]
                    }
                  }
                }
                n661 = Or(x=w1895, y=w1891) -> (x .or. y?=w1898:bool)
                n662 = Select(t=State_Type_Definitions,_for_0.26g_versions_and_later_2."True Stop" ("Enum"), s=w1891, f=State_Type_Definitions,_for_0.26g_versions_and_later_2."Task 8K: RAISE MY SWORD" ("Enum")) -> (s? t:f=w1893:T18)
                n663 = Select(t=w1893, s=w1898, f=State_Type_Definitions,_for_0.26g_versions_and_later_2."Task 8J: CLOSE CLAW" ("Enum")) -> (s? t:f=w1897:T18)
              }
              frame "Exit" {
                n664 = for {
                  shift-right: [w1920] -> w1917
                  shift-left: w1914 -> [w1921]
                  tunnel: string[] ["STOP", "RESET ENCODERS", "RESET YAW", "ARDUINO MODE 0"] -> [w1919] mode=indexing
                  n665 = Enqueue Element(queue=w1921, element=w1919) -> (queue out=w1920:refnum<queue>)  [unwired: 2 in, 2 out]
                }
              }
            }
          }
          frame "Task 8K: RAISE MY SWORD" {
            # ">>> yStepper command>>>"
            # ">> Manual override >>"
            n666 = Dequeue Element(queue=w1932, timeout in ms (-1)=w1931, error in (no error)=w1933) -> (element=w1930:T10)  [unwired: 3 out]
            n667 = Equal?(x=w1929, y=u8 60) -> (x = y?=w1927:bool)
            n668 = case shown="\"Start Task 1\", Default" w1930 {
              tunnel: [w1943 State_Type_Definitions,_for_0.26g_versions_and_later_2."True Stop" ("Enum")] -> w1934
              tunnel: [w1946 w1963] -> w1935
              tunnel: [State_Type_Definitions,_for_0.26g_versions_and_later_2."Idle" ("Enum") State_Type_Definitions,_for_0.26g_versions_and_later_2."Shutdown" ("Enum")] -> w1936
              tunnel: w1927 -> [w1942 _]
              tunnel: w1926 -> [w1941 _]
              tunnel: w1925 -> [w1937 w1960]
              frame "Start Task 1", Default {
                # "Stays in Task 5_A until stepper reaches desired \nheight"
                # "T: Go back to idle, F: Continue with task\""
                # ">> Manual override >>"
                n669 = case shown="True" w1942 {
                  tunnel: [w1950 w1956] -> w1946
                  tunnel: w1937 -> [w1948 w1954]
                  frame False {
                    n670 = for {
                      tunnel: string[] ["Z STEPPER CAM HEIGHT", "READ STEPPER VALUES"] ("element") -> [w1951] mode=indexing
                      shift-right: [w1953] -> w1950
                      shift-left: w1948 -> [w1952]
                      n671 = Enqueue Element(queue=w1952, element=w1951) -> (queue out=w1953:refnum<queue>)  [unwired: 2 in, 2 out]
                    }
                  }
                  frame True {
                    n672 = for {
                      shift-right: [w1958] -> w1956
                      shift-left: w1954 -> [w1959]
                      tunnel: string[] ["CAM CLOSE", "DISPOSE CAM BUFFERS", "DISPOSE PROC BUFFERS", "RESET ENCODERS"] -> [w1957] mode=indexing
                      n673 = Enqueue Element(queue=w1959, element=w1957) -> (queue out=w1958:refnum<queue>)  [unwired: 2 in, 2 out]
                    }
                  }
                }
                n674 = Or(x=w1942, y=w1941) -> (x .or. y?=w1944:bool)
                n675 = Select(t=State_Type_Definitions,_for_0.26g_versions_and_later_2."True Stop" ("Enum"), s=w1941, f=State_Type_Definitions,_for_0.26g_versions_and_later_2."True Stop" ("Enum")) -> (s? t:f=w1938:T18)
                n676 = Select(t=w1938, s=w1944, f=State_Type_Definitions,_for_0.26g_versions_and_later_2."Task 8K: RAISE MY SWORD" ("Enum")) -> (s? t:f=w1943:T18)
              }
              frame "Exit" {
                n677 = for {
                  shift-right: [w1966] -> w1963
                  shift-left: w1960 -> [w1967]
                  tunnel: string[] ["STOP", "RESET ENCODERS", "RESET YAW", "ARDUINO MODE 0"] -> [w1965] mode=indexing
                  n678 = Enqueue Element(queue=w1967, element=w1965) -> (queue out=w1966:refnum<queue>)  [unwired: 2 in, 2 out]
                }
              }
            }
          }
          frame "Task 9A: Raise Arm" {
            # ">>> Motor control cluster >>>"
            # ">> Stepper height reeached >>"
            # ">>> yStepper command>>>"
            # ">> Manual override >>"
            n679 = Dequeue Element(queue=w1980, timeout in ms (-1)=w1975, error in (no error)=w1979) -> (element=w1982:T10)  [unwired: 3 out]
            n680 = Equal?(x=w1977, y=u8 50) -> (x = y?=w1968:bool)
            n681 = case shown="\"Start Task 1\", Default" w1982 {
              tunnel: [w1993 State_Type_Definitions,_for_0.26g_versions_and_later_2."True Stop" ("Enum")] -> w1973
              tunnel: [w1991 w2008] -> w1972
              tunnel: w1976 -> [w1990 _]
              tunnel: w1978 -> [w1984 _]
              tunnel: [State_Type_Definitions,_for_0.26g_versions_and_later_2."Idle" ("Enum") State_Type_Definitions,_for_0.26g_versions_and_later_2."Shutdown" ("Enum")] -> w1974
              tunnel: w1968 -> [w1983 _]
              frame "Start Task 1", Default {
                # ">> WIill proceed to part ii if not manual override >>"
                # ">>If ENABLE or Trigger is set to true>>"
                n682 = Or(x=w1983, y=w1984) -> (x .or. y?=w1985:bool)
                n683 = case shown="False" w1983 {
                  tunnel: [w1996 w2002] -> w1991
                  tunnel: w1990 -> [w1995 w2001]
                  frame False {
                    n684 = for {
                      shift-right: [w1998] -> w1996
                      shift-left: w1995 -> [w1999]
                      tunnel: string[] ["Z STEPPER BOX HEIGHT", "READ STEPPER VALUES"] ("element") -> [w1997] mode=indexing
                      n685 = Enqueue Element(queue=w1999, element=w1997) -> (queue out=w1998:refnum<queue>)  [unwired: 2 in, 2 out]
                    }
                  }
                  frame True {
                    n686 = for {
                      shift-right: [w2004] -> w2002
                      shift-left: w2001 -> [w2005]
                      tunnel: string[] ["READ NAVX", "RESET FLAGS", "RESET YAW", "", "", ""] -> [w2003] mode=indexing
                      n687 = Enqueue Element(queue=w2005, element=w2003) -> (queue out=w2004:refnum<queue>)  [unwired: 2 in, 2 out]
                    }
                  }
                }
                n688 = Select(t=State_Type_Definitions,_for_0.26g_versions_and_later_2."True Stop" ("Enum"), s=w1984, f=State_Type_Definitions,_for_0.26g_versions_and_later_2."Task 9B: Rotate to Angle" ("Enum")) -> (s? t:f=w1987:T18)
                n689 = Select(t=w1987, s=w1985, f=State_Type_Definitions,_for_0.26g_versions_and_later_2."Task 9A: Raise Arm" ("Enum")) -> (s? t:f=w1993:T18)
              }
              frame "Exit" {
                n690 = for {
                  shift-right: [w2011] -> w2008
                  shift-left: _ -> [w2012]
                  tunnel: string[] ["STOP", "RESET ENCODERS", "RESET YAW", ""] -> [w2010] mode=indexing
                  n691 = Enqueue Element(queue=w2012, element=w2010) -> (queue out=w2011:refnum<queue>)  [unwired: 2 in, 2 out]
                }
              }
            }
          }
          frame "Task 9B: Rotate to Angle" {
            # ">>> Motor control cluster >>>"
            # ">>> yStepper command>>>"
            n692 = Dequeue Element(queue=w2026, timeout in ms (-1)=w2025, error in (no error)=w2024) -> (element=w2028:T10)  [unwired: 3 out]
            n693 = In Range and Coerce(upper limit=65.0, x=w2018, lower limit=58.0) -> (In Range?=w2013:bool)  [unwired: 1 out]
            n694 = case shown="\"Start Task 1\", Default" w2028 {
              tunnel: w2019 -> [w2031 _]
              tunnel: [w2039 State_Type_Definitions,_for_0.26g_versions_and_later_2."True Stop" ("Enum")] -> w2021
              tunnel: w2027 -> [w2037 w2055]
              tunnel: [w2036 w2054] -> w2020
              tunnel: [State_Type_Definitions,_for_0.26g_versions_and_later_2."Idle" ("Enum") State_Type_Definitions,_for_0.26g_versions_and_later_2."Shutdown" ("Enum")] -> w2022
              tunnel: w2013 -> [w2029 _]
              frame "Start Task 1", Default {
                n695 = Or(x=w2029, y=w2031) -> (x .or. y?=w2030:bool)
                n696 = case shown="False" w2029 {
                  tunnel: w2037 -> [w2042 w2048]
                  tunnel: [w2041 w2046] -> w2036
                  frame False {
                    n697 = for {
                      shift-right: [w2044] -> w2041
                      shift-left: w2042 -> [w2045]
                      tunnel: string[] ["READ NAVX", "R-CW", ""] ("element") -> [w2043] mode=indexing
                      n698 = Enqueue Element(queue=w2045, element=w2043) -> (queue out=w2044:refnum<queue>)  [unwired: 2 in, 2 out]
                    }
                  }
                  frame True {
                    n699 = for {
                      shift-right: [w2050] -> w2046
                      shift-left: w2048 -> [w2051]
                      tunnel: string[] ["STOP", "RESET ENCODERS", "RESET YAW", "", ""] -> [w2049] mode=indexing
                      n700 = Enqueue Element(queue=w2051, element=w2049) -> (queue out=w2050:refnum<queue>)  [unwired: 2 in, 2 out]
                    }
                  }
                }
                n701 = Select(t=State_Type_Definitions,_for_0.26g_versions_and_later_2."True Stop" ("Enum"), s=w2031, f=State_Type_Definitions,_for_0.26g_versions_and_later_2."Task 9C: Detect Box") -> (s? t:f=w2033:T18)
                n702 = Select(t=w2033, s=w2030, f=State_Type_Definitions,_for_0.26g_versions_and_later_2."Task 9B: Rotate to Angle" ("Enum")) -> (s? t:f=w2039:T18)
              }
              frame "Exit" {
                n703 = for {
                  shift-right: [w2058] -> w2054
                  shift-left: w2055 -> [w2059]
                  tunnel: string[] ["STOP", "RESET ENCODERS", "RESET YAW", ""] -> [w2057] mode=indexing
                  n704 = Enqueue Element(queue=w2059, element=w2057) -> (queue out=w2058:refnum<queue>)  [unwired: 2 in, 2 out]
                }
              }
            }
          }
          frame "Task 9C: Detect Box" {
            # ">>> Motor control cluster >>>"
            # ">>Line Detected>>"
            # ">>Action Queue>>"
            # ">>> yStepper command>>>"
            n705 = Dequeue Element(queue=w2071, timeout in ms (-1)=w2070, error in (no error)=w2069) -> (element=w2072:T10)  [unwired: 3 out]
            n706 = case shown="\"Start Task 1\", Default" w2072 {
              tunnel: w2067 -> [w2073 _]
              tunnel: [w2083 State_Type_Definitions,_for_0.26g_versions_and_later_2."True Stop" ("Enum")] -> w2064
              tunnel: w2068 -> [w2081 w2099]
              tunnel: [w2080 w2098] -> w2063
              tunnel: [State_Type_Definitions,_for_0.26g_versions_and_later_2."Idle" ("Enum") State_Type_Definitions,_for_0.26g_versions_and_later_2."Shutdown" ("Enum")] -> w2066
              tunnel: w2060 -> [w2074 _]
              frame "Start Task 1", Default {
                n707 = Or(x=w2073, y=w2074) -> (x .or. y?=w2075:bool)
                n708 = case shown="False" w2074 {
                  tunnel: w2081 -> [w2086 w2092]
                  tunnel: [w2085 w2090] -> w2080
                  frame False {
                    n709 = for {
                      shift-right: [w2088] -> w2085
                      shift-left: w2086 -> [w2089]
                      tunnel: string[] ["READ IR", "READ LINE SENSOR", "FORWARD - IR ASSIST"] ("element") -> [w2087] mode=indexing
                      n710 = Enqueue Element(queue=w2089, element=w2087) -> (queue out=w2088:refnum<queue>)  [unwired: 2 in, 2 out]
                    }
                  }
                  frame True {
                    n711 = for {
                      shift-right: [w2094] -> w2090
                      shift-left: w2092 -> [w2095]
                      tunnel: string[] ["STOP", "RESET ENCODERS", "RESET YAW", "RESET FLAGS"] -> [w2093] mode=indexing
                      n712 = Enqueue Element(queue=w2095, element=w2093) -> (queue out=w2094:refnum<queue>)  [unwired: 2 in, 2 out]
                    }
                  }
                }
                n713 = Select(t=State_Type_Definitions,_for_0.26g_versions_and_later_2."True Stop" ("Enum"), s=w2073, f=State_Type_Definitions,_for_0.26g_versions_and_later_2."Task 9D: MOVE FORWARD") -> (s? t:f=w2077:T18)
                n714 = Select(t=w2077, s=w2075, f=State_Type_Definitions,_for_0.26g_versions_and_later_2."Task 9C: Detect Box" ("Enum")) -> (s? t:f=w2083:T18)
              }
              frame "Exit" {
                n715 = for {
                  shift-right: [w2102] -> w2098
                  shift-left: w2099 -> [w2103]
                  tunnel: string[] ["STOP", "RESET ENCODERS", "RESET YAW", ""] -> [w2101] mode=indexing
                  n716 = Enqueue Element(queue=w2103, element=w2101) -> (queue out=w2102:refnum<queue>)  [unwired: 2 in, 2 out]
                }
              }
            }
          }
          frame "Task 9D: MOVE FORWARD" {
            (unwired) 50.0 ("y")
            # ">> Item Selection Bias >>"
            # ">> Wall detected >>"
            # ">> Manual override >>"
            # ">>Table Detected>>"
            # ">>> Motor control cluster >>>"
            # ">>Table or wall detectected>>"
            # ">>Action Queue>>"
            # ">>> yStepper command>>>"
            n717 = Dequeue Element(queue=w2121, timeout in ms (-1)=w2120, error in (no error)=w2119) -> (element=w2122:T10)  [unwired: 3 out]
            n718 = Less Or Equal?(x=w2110, y=18.0) -> (x <= y?=w2105:bool)
            n719 = Less?(x=w2108, y=20.0) -> (x < y?=w2106:bool)
            n720 = Or(x=w2105, y=w2106) -> (x .or. y?=w2104:bool)
            n721 = case shown="\"Start Task 1\", Default" w2122 {
              tunnel: w2117 -> [w2123 _]
              tunnel: [w2133 State_Type_Definitions,_for_0.26g_versions_and_later_2."True Stop" ("Enum")] -> w2114
              tunnel: w2118 -> [w2131 w2149]
              tunnel: [w2130 w2148] -> w2113
              tunnel: [State_Type_Definitions,_for_0.26g_versions_and_later_2."Idle" ("Enum") State_Type_Definitions,_for_0.26g_versions_and_later_2."Shutdown" ("Enum")] -> w2116
              tunnel: w2104 -> [w2124 _]
              frame "Start Task 1", Default {
                n722 = Or(x=w2123, y=w2124) -> (x .or. y?=w2125:bool)
                n723 = case shown="True" w2124 {
                  tunnel: w2131 -> [w2136 w2142]
                  tunnel: [w2135 w2140] -> w2130
                  frame False {
                    n724 = for {
                      shift-right: [w2138] -> w2135
                      shift-left: w2136 -> [w2139]
                      tunnel: string[] ["READ IR", "FORWARD - IR ASSIST", ""] ("element") -> [w2137] mode=indexing
                      n725 = Enqueue Element(queue=w2139, element=w2137) -> (queue out=w2138:refnum<queue>)  [unwired: 2 in, 2 out]
                    }
                  }
                  frame True {
                    n726 = for {
                      shift-right: [w2144] -> w2140
                      shift-left: w2142 -> [w2145]
                      tunnel: string[] ["STOP", "RESET ENCODERS", "RESET YAW", "RESET FLAGS"] -> [w2143] mode=indexing
                      n727 = Enqueue Element(queue=w2145, element=w2143) -> (queue out=w2144:refnum<queue>)  [unwired: 2 in, 2 out]
                    }
                  }
                }
                n728 = Select(t=State_Type_Definitions,_for_0.26g_versions_and_later_2."True Stop" ("Enum"), s=w2123, f=State_Type_Definitions,_for_0.26g_versions_and_later_2."Task 9E: MOVE LEFT") -> (s? t:f=w2127:T18)
                n729 = Select(t=w2127, s=w2125, f=State_Type_Definitions,_for_0.26g_versions_and_later_2."Task 9D: MOVE FORWARD" ("Enum")) -> (s? t:f=w2133:T18)
              }
              frame "Exit" {
                n730 = for {
                  shift-right: [w2152] -> w2148
                  shift-left: w2149 -> [w2153]
                  tunnel: string[] ["STOP", "RESET ENCODERS", "RESET YAW", ""] -> [w2151] mode=indexing
                  n731 = Enqueue Element(queue=w2153, element=w2151) -> (queue out=w2152:refnum<queue>)  [unwired: 2 in, 2 out]
                }
              }
            }
          }
          frame "Task 9E: MOVE LEFT" {
            # ">> Item Selection Bias >>"
            # ">> Line detected? >>"
            # ">> Manual override >>"
            # ">>> Motor control cluster >>>"
            # ">>Action Queue>>"
            # ">>> yStepper command>>>"
            n732 = Dequeue Element(queue=w2165, timeout in ms (-1)=w2164, error in (no error)=w2163) -> (element=w2166:T10)  [unwired: 3 out]
            n733 = case shown="\"Start Task 1\", Default" w2166 {
              tunnel: w2161 -> [w2167 _]
              tunnel: [w2177 State_Type_Definitions,_for_0.26g_versions_and_later_2."True Stop" ("Enum")] -> w2158
              tunnel: w2162 -> [w2175 w2193]
              tunnel: [w2174 w2192] -> w2157
              tunnel: [State_Type_Definitions,_for_0.26g_versions_and_later_2."Idle" ("Enum") State_Type_Definitions,_for_0.26g_versions_and_later_2."Shutdown" ("Enum")] -> w2160
              tunnel: w2154 -> [w2168 _]
              frame "Start Task 1", Default {
                n734 = Or(x=w2167, y=w2168) -> (x .or. y?=w2169:bool)
                n735 = case shown="True" w2168 {
                  tunnel: w2175 -> [w2180 w2186]
                  tunnel: [w2179 w2184] -> w2174
                  frame False {
                    n736 = for {
                      shift-right: [w2182] -> w2179
                      shift-left: w2180 -> [w2183]
                      tunnel: string[] ["LEFT", "READ NAVX", "READ LINE SENSOR", ""] ("element") -> [w2181] mode=indexing
                      n737 = Enqueue Element(queue=w2183, element=w2181) -> (queue out=w2182:refnum<queue>)  [unwired: 2 in, 2 out]
                    }
                  }
                  frame True {
                    n738 = for {
                      shift-right: [w2188] -> w2184
                      shift-left: w2186 -> [w2189]
                      tunnel: string[] ["STOP", "RESET ENCODERS", "RESET YAW", "BOX COLOUR", "", ""] -> [w2187] mode=indexing
                      n739 = Enqueue Element(queue=w2189, element=w2187) -> (queue out=w2188:refnum<queue>)  [unwired: 2 in, 2 out]
                    }
                  }
                }
                n740 = Select(t=State_Type_Definitions,_for_0.26g_versions_and_later_2."True Stop" ("Enum"), s=w2167, f=State_Type_Definitions,_for_0.26g_versions_and_later_2."Task 9F: SCAN BOX") -> (s? t:f=w2171:T18)
                n741 = Select(t=w2171, s=w2169, f=State_Type_Definitions,_for_0.26g_versions_and_later_2."Task 9E: MOVE LEFT" ("Enum")) -> (s? t:f=w2177:T18)
              }
              frame "Exit" {
                n742 = for {
                  shift-right: [w2196] -> w2192
                  shift-left: w2193 -> [w2197]
                  tunnel: string[] ["STOP", "RESET ENCODERS", "RESET YAW", ""] -> [w2195] mode=indexing
                  n743 = Enqueue Element(queue=w2197, element=w2195) -> (queue out=w2196:refnum<queue>)  [unwired: 2 in, 2 out]
                }
              }
            }
          }
          frame "Task 9F: SCAN BOX" {
            # ">>> Motor control cluster >>>"
            # ">>Colour detection >>"
            # ">>> yStepper command>>>"
            # ">> Manual override >>"
            n744 = Dequeue Element(queue=w2214, timeout in ms (-1)=w2212, error in (no error)=w2213) -> (element=w2207:T10)  [unwired: 3 out]
            n745 = call "Box Colour FGV.vi"("Init/R/W State"=Box_Colour_FGV_States."Read") -> ("Colour to detect (output)"=w2200:T2)  [unwired: 9 in, 1 out]
            n746 = Equal?(x=w2201, y=w2200) -> (x = y?=w2199:bool)
            n747 = case shown="\"Start Task 1\", Default" w2207 {
              tunnel: [w2227 State_Type_Definitions,_for_0.26g_versions_and_later_2."True Stop" ("Enum")] -> w2204
              tunnel: [w2225 w2242] -> w2205
              tunnel: w2206 -> [w2224 _]
              tunnel: w2208 -> [w2217 _]
              tunnel: [State_Type_Definitions,_for_0.26g_versions_and_later_2."Idle" ("Enum") State_Type_Definitions,_for_0.26g_versions_and_later_2."Shutdown" ("Enum")] -> w2203
              tunnel: w2198 -> [w2218 _]
              tunnel: w2199 -> [w2216 _]
              frame "Start Task 1", Default {
                # ">> Will stop either due to manual override or is same box colour >>"
                # ">> WIill proceed to part ii if not manual override >>"
                # ">>If ENABLE or Trigger is set to true>>"
                n748 = Or(x=w2218, y=w2217) -> (x .or. y?=w2219:bool)
                n749 = case shown="True" w2218 {
                  tunnel: [w2230 w2236] -> w2225
                  tunnel: w2224 -> [w2229 w2235]
                  frame False {
                    n750 = for {
                      shift-right: [w2232] -> w2230
                      shift-left: w2229 -> [w2233]
                      tunnel: string[] ["", ""] ("element") -> [w2231] mode=indexing
                      n751 = Enqueue Element(queue=w2233, element=w2231) -> (queue out=w2232:refnum<queue>)  [unwired: 2 in, 2 out]
                    }
                  }
                  frame True {
                    n752 = for {
                      shift-right: [w2238] -> w2236
                      shift-left: w2235 -> [w2239]
                      tunnel: string[] ["RESET ENCODER", "RESET FLAGS", "RESET YAW", "", "", ""] -> [w2237] mode=indexing
                      n753 = Enqueue Element(queue=w2239, element=w2237) -> (queue out=w2238:refnum<queue>)  [unwired: 2 in, 2 out]
                    }
                  }
                }
                n754 = Or(x=w2217, y=w2216) -> (x .or. y?=w2215:bool)
                n755 = Select(t=State_Type_Definitions,_for_0.26g_versions_and_later_2."True Stop" ("Enum"), s=w2215, f=State_Type_Definitions,_for_0.26g_versions_and_later_2."Task 9G: MOVE RIGHT" ("Enum")) -> (s? t:f=w2221:T18)
                n756 = Select(t=w2221, s=w2219, f=State_Type_Definitions,_for_0.26g_versions_and_later_2."Task 9F: SCAN BOX" ("Enum")) -> (s? t:f=w2227:T18)
              }
              frame "Exit" {
                n757 = for {
                  shift-right: [w2245] -> w2242
                  shift-left: _ -> [w2246]
                  tunnel: string[] ["STOP", "RESET ENCODERS", "RESET YAW", ""] -> [w2244] mode=indexing
                  n758 = Enqueue Element(queue=w2246, element=w2244) -> (queue out=w2245:refnum<queue>)  [unwired: 2 in, 2 out]
                }
              }
            }
          }
          frame "Task 9G: MOVE RIGHT" {
            # ">>> Motor control cluster >>>"
            # ">>> yStepper command>>>"
            n759 = Dequeue Element(queue=w2258, timeout in ms (-1)=w2257, error in (no error)=w2256) -> (element=w2263:T10)  [unwired: 3 out]
            n760 = Greater?(x=w2248, y=50.0) -> (0:w2251:bool)
            n761 = And(x=w2249, y=w2251) -> (x .and. y?=w2247:bool)
            n762 = case shown="\"Start Task 1\", Default" w2263 {
              tunnel: w2247 -> [w2266 _]
              tunnel: [w2273 State_Type_Definitions,_for_0.26g_versions_and_later_2."True Stop" ("Enum")] -> w2262
              tunnel: w2255 -> [w2265 _]
              tunnel: w2259 -> [w2272 w2289]
              tunnel: [w2271 w2290] -> w2261
              tunnel: [State_Type_Definitions,_for_0.26g_versions_and_later_2."Idle" ("Enum") State_Type_Definitions,_for_0.26g_versions_and_later_2."Shutdown" ("Enum")] -> w2260
              frame "Start Task 1", Default {
                n763 = case shown="True" w2266 {
                  tunnel: w2272 -> [w2276 w2283]
                  tunnel: [w2277 w2282] -> w2271
                  frame False {
                    n764 = for {
                      tunnel: string[] ["READ LINE SENSOR", "READ NAVX", "RIGHT", "READ ENCODERS"] ("element") -> [w2278] mode=indexing
                      shift-right: [w2280] -> w2277
                      shift-left: w2276 -> [w2279]
                      n765 = Enqueue Element(queue=w2279, element=w2278) -> (queue out=w2280:refnum<queue>)  [unwired: 2 in, 2 out]
                    }
                  }
                  frame True {
                    n766 = for {
                      shift-right: [w2285] -> w2282
                      shift-left: w2283 -> [w2286]
                      tunnel: string[] ["RESET ENCODERS", "RESET YAW", "RESET FLAGS", "STOP", "BOX COLOUR"] -> [w2284] mode=indexing
                      n767 = Enqueue Element(queue=w2286, element=w2284) -> (queue out=w2285:refnum<queue>)  [unwired: 2 in, 2 out]
                    }
                  }
                }
                n768 = Or(x=w2266, y=w2265) -> (x .or. y?=w2264:bool)
                n769 = Select(t=State_Type_Definitions,_for_0.26g_versions_and_later_2."True Stop" ("Enum"), s=w2265, f=State_Type_Definitions,_for_0.26g_versions_and_later_2."Task 9H: SCAN BOX 2" ("Enum")) -> (s? t:f=w2267:T18)
                n770 = Select(t=w2267, s=w2264, f=State_Type_Definitions,_for_0.26g_versions_and_later_2."Task 9G: MOVE RIGHT" ("Enum")) -> (s? t:f=w2273:T18)
              }
              frame "Exit" {
                n771 = for {
                  shift-right: [w2293] -> w2290
                  shift-left: w2289 -> [w2294]
                  tunnel: string[] ["STOP", "RESET ENCODERS", "RESET YAW", "ARDUINO MODE 0"] -> [w2292] mode=indexing
                  n772 = Enqueue Element(queue=w2294, element=w2292) -> (queue out=w2293:refnum<queue>)  [unwired: 2 in, 2 out]
                }
              }
            }
          }
          frame "Task 9H: SCAN BOX 2" {
            # ">> Item Selection Bias >>"
            # ">>> Motor control cluster >>>"
            # ">>> yStepper command>>>"
            n773 = Dequeue Element(queue=w2304, timeout in ms (-1)=w2305, error in (no error)=w2306) -> (element=w2308:T10)  [unwired: 3 out]
            n774 = call "Box Colour FGV.vi"("Init/R/W State"=Box_Colour_FGV_States."Read") -> ("Colour to detect (output)"=w2298:T2)  [unwired: 9 in, 1 out]
            n775 = Equal?(x=w2297, y=w2298) -> (x = y?=w2296:bool)
            n776 = case shown="\"Start Task 1\", Default" w2308 {
              tunnel: w2295 -> [w2316 _]
              tunnel: [w2323 State_Type_Definitions,_for_0.26g_versions_and_later_2."True Stop" ("Enum")] -> w2301
              tunnel: w2307 -> [w2313 _]
              tunnel: w2303 -> [w2322 w2339]
              tunnel: [w2321 w2340] -> w2302
              tunnel: [State_Type_Definitions,_for_0.26g_versions_and_later_2."Idle" ("Enum") State_Type_Definitions,_for_0.26g_versions_and_later_2."Shutdown" ("Enum")] -> w2300
              tunnel: w2296 -> [w2314 _]
              frame "Start Task 1", Default {
                n777 = Or(x=w2316, y=w2313) -> (x .or. y?=w2315:bool)
                n778 = Or(x=w2314, y=w2313) -> (x .or. y?=w2312:bool)
                n779 = case shown="True" w2316 {
                  tunnel: w2322 -> [w2326 w2333]
                  tunnel: [w2327 w2332] -> w2321
                  frame False {
                    n780 = for {
                      tunnel: string[] ["", "", "", ""] ("element") -> [w2328] mode=indexing
                      shift-right: [w2330] -> w2327
                      shift-left: w2326 -> [w2329]
                      n781 = Enqueue Element(queue=w2329, element=w2328) -> (queue out=w2330:refnum<queue>)  [unwired: 2 in, 2 out]
                    }
                  }
                  frame True {
                    n782 = for {
                      shift-right: [w2335] -> w2332
                      shift-left: w2333 -> [w2336]
                      tunnel: string[] ["READ NAVX", "RESET FLAGS", "RESET ENCODERS", "", "", ""] -> [w2334] mode=indexing
                      n783 = Enqueue Element(queue=w2336, element=w2334) -> (queue out=w2335:refnum<queue>)  [unwired: 2 in, 2 out]
                    }
                  }
                }
                n784 = Select(t=State_Type_Definitions,_for_0.26g_versions_and_later_2."True Stop" ("Enum"), s=w2312, f=State_Type_Definitions,_for_0.26g_versions_and_later_2."Task 9I: ROTATE 90 CW" ("Enum")) -> (s? t:f=w2317:T18)
                n785 = Select(t=w2317, s=w2315, f=State_Type_Definitions,_for_0.26g_versions_and_later_2."Task 9H: SCAN BOX 2" ("Enum")) -> (s? t:f=w2323:T18)
              }
              frame "Exit" {
                n786 = for {
                  shift-right: [w2343] -> w2340
                  shift-left: w2339 -> [w2344]
                  tunnel: string[] ["STOP", "RESET ENCODERS", "RESET YAW", "ARDUINO MODE 0"] -> [w2342] mode=indexing
                  n787 = Enqueue Element(queue=w2344, element=w2342) -> (queue out=w2343:refnum<queue>)  [unwired: 2 in, 2 out]
                }
              }
            }
          }
          frame "Task 9I: ROTATE 90 CW" {
            # "High battery voltage: -36\nMid voltage: -38 \nLow voltage: -40"
            # ">> Item Selection Bias >>"
            n788 = Dequeue Element(queue=w2348, timeout in ms (-1)=w2349, error in (no error)=w2350) -> (element=w2356:T10)  [unwired: 3 out]
            n789 = Less?(x=w2346, y=-38.0) -> (x < y?=w2345:bool)
            n790 = case shown="\"Start Task 1\", Default" w2356 {
              tunnel: w2345 -> [w2362 _]
              tunnel: [w2369 State_Type_Definitions,_for_0.26g_versions_and_later_2."True Stop" ("Enum")] -> w2353
              tunnel: w2351 -> [w2361 _]
              tunnel: w2355 -> [w2368 w2385]
              tunnel: [w2367 w2386] -> w2354
              tunnel: [State_Type_Definitions,_for_0.26g_versions_and_later_2."Idle" ("Enum") State_Type_Definitions,_for_0.26g_versions_and_later_2."Shutdown" ("Enum")] -> w2352
              frame "Start Task 1", Default {
                n791 = case shown="False" w2362 {
                  tunnel: w2368 -> [w2372 w2379]
                  tunnel: [w2373 w2378] -> w2367
                  frame False {
                    n792 = for {
                      tunnel: string[] ["R-CW", "READ ENCODERS", "READ IR"] ("element") -> [w2374] mode=indexing
                      shift-right: [w2376] -> w2373
                      shift-left: w2372 -> [w2375]
                      n793 = Enqueue Element(queue=w2375, element=w2374) -> (queue out=w2376:refnum<queue>)  [unwired: 2 in, 2 out]
                    }
                  }
                  frame True {
                    n794 = for {
                      shift-right: [w2381] -> w2378
                      shift-left: w2379 -> [w2382]
                      tunnel: string[] ["STOP", "RESET ENCODERS", "RESET YAW", "RESET FLAGS", "READ IR", ""] -> [w2380] mode=indexing
                      n795 = Enqueue Element(queue=w2382, element=w2380) -> (queue out=w2381:refnum<queue>)  [unwired: 2 in, 2 out]
                    }
                  }
                }
                n796 = Or(x=w2362, y=w2361) -> (x .or. y?=w2360:bool)
                n797 = Select(t=State_Type_Definitions,_for_0.26g_versions_and_later_2."True Stop" ("Enum"), s=w2361, f=State_Type_Definitions,_for_0.26g_versions_and_later_2."Task 9J: FORWARD" ("Enum")) -> (s? t:f=w2363:T18)
                n798 = Select(t=w2363, s=w2360, f=State_Type_Definitions,_for_0.26g_versions_and_later_2."Task 9I: ROTATE 90 CW" ("Enum")) -> (s? t:f=w2369:T18)
              }
              frame "Exit" {
                n799 = for {
                  shift-right: [w2389] -> w2386
                  shift-left: w2385 -> [w2390]
                  tunnel: string[] ["STOP", "RESET ENCODERS", "RESET YAW", "ARDUINO MODE 0"] -> [w2388] mode=indexing
                  n800 = Enqueue Element(queue=w2390, element=w2388) -> (queue out=w2389:refnum<queue>)  [unwired: 2 in, 2 out]
                }
              }
            }
          }
          frame "Task 9J: FORWARD" {
            # "Tried values: 70, 150"
            # ">>Stops if either table or wall is obstructing >>"
            # ">> Item Selection Bias >>"
            n801 = Less?(x=w2400, y=25.0) -> (x < y?=w2398:bool)
            n802 = Greater Than 0?(x=w2400) -> (x > 0?=w2399:bool)
            n803 = Less?(x=w2394, y=250.0) -> (x < y?=w2397:bool)
            n804 = Greater Than 0?(x=w2394) -> (x > 0?=w2396:bool)
            n805 = Dequeue Element(queue=w2406, timeout in ms (-1)=w2407, error in (no error)=w2408) -> (element=w2410:T10)  [unwired: 3 out]
            n806 = And(x=w2399, y=w2398) -> (x .and. y?=w2392:bool)
            n807 = And(x=w2396, y=w2397) -> (x .and. y?=w2393:bool)
            n808 = Or(x=w2392, y=w2393) -> (x .or. y?=w2391:bool)
            n809 = case shown="\"Start Task 1\", Default" w2410 {
              tunnel: w2391 -> [w2416 _]
              tunnel: [w2423 State_Type_Definitions,_for_0.26g_versions_and_later_2."True Stop" ("Enum")] -> w2404
              tunnel: w2409 -> [w2415 _]
              tunnel: w2405 -> [w2422 w2439]
              tunnel: [w2421 w2440] -> w2403
              tunnel: [State_Type_Definitions,_for_0.26g_versions_and_later_2."Idle" ("Enum") State_Type_Definitions,_for_0.26g_versions_and_later_2."Shutdown" ("Enum")] -> w2402
              frame "Start Task 1", Default {
                n810 = case shown="False" w2416 {
                  tunnel: w2422 -> [w2426 w2433]
                  tunnel: [w2427 w2432] -> w2421
                  frame False {
                    n811 = for {
                      tunnel: string[] ["READ IR", "READ NAVX", "FORWARD"] ("element") -> [w2428] mode=indexing
                      shift-right: [w2430] -> w2427
                      shift-left: w2426 -> [w2429]
                      n812 = Enqueue Element(queue=w2429, element=w2428) -> (queue out=w2430:refnum<queue>)  [unwired: 2 in, 2 out]
                    }
                  }
                  frame True {
                    n813 = for {
                      shift-right: [w2435] -> w2432
                      shift-left: w2433 -> [w2436]
                      tunnel: string[] ["STOP", "RESET ENCODERS", "RESET YAW", "RESET FLAGS", "", ""] -> [w2434] mode=indexing
                      n814 = Enqueue Element(queue=w2436, element=w2434) -> (queue out=w2435:refnum<queue>)  [unwired: 2 in, 2 out]
                    }
                  }
                }
                n815 = Or(x=w2416, y=w2415) -> (x .or. y?=w2414:bool)
                n816 = Select(t=State_Type_Definitions,_for_0.26g_versions_and_later_2."True Stop" ("Enum"), s=w2415, f=State_Type_Definitions,_for_0.26g_versions_and_later_2."True Stop" ("Enum")) -> (s? t:f=w2417:T18)
                n817 = Select(t=w2417, s=w2414, f=State_Type_Definitions,_for_0.26g_versions_and_later_2."Task 9J: FORWARD" ("Enum")) -> (s? t:f=w2423:T18)
              }
              frame "Exit" {
                n818 = for {
                  shift-right: [w2443] -> w2440
                  shift-left: w2439 -> [w2444]
                  tunnel: string[] ["STOP", "RESET ENCODERS", "RESET YAW", "ARDUINO MODE 0"] -> [w2442] mode=indexing
                  n819 = Enqueue Element(queue=w2444, element=w2442) -> (queue out=w2443:refnum<queue>)  [unwired: 2 in, 2 out]
                }
              }
            }
          }
          frame "Task 9K: MOVE RIGHT" {
            # ">>> Motor control cluster >>>"
            # ">>> yStepper command>>>"
            # ">> Item Selection Bias >>"
            n820 = Dequeue Element(queue=w2452, timeout in ms (-1)=w2451, error in (no error)=w2450) -> (element=w2454:T10)  [unwired: 3 out]
            n821 = case shown="\"Start Task 1\", Default" w2454 {
              tunnel: w2445 -> [w2460 _]
              tunnel: [w2467 State_Type_Definitions,_for_0.26g_versions_and_later_2."True Stop" ("Enum")] -> w2448
              tunnel: w2449 -> [w2459 _]
              tunnel: w2453 -> [w2466 w2483]
              tunnel: [w2465 w2484] -> w2446
              tunnel: [State_Type_Definitions,_for_0.26g_versions_and_later_2."Idle" ("Enum") State_Type_Definitions,_for_0.26g_versions_and_later_2."Shutdown" ("Enum")] -> w2447
              frame "Start Task 1", Default {
                n822 = case shown="False" w2460 {
                  tunnel: w2466 -> [w2470 w2477]
                  tunnel: [w2471 w2476] -> w2465
                  frame False {
                    n823 = for {
                      tunnel: string[] ["READ LINE SENSOR", "READ NAVX", "RIGHT", ""] ("element") -> [w2472] mode=indexing
                      shift-right: [w2474] -> w2471
                      shift-left: w2470 -> [w2473]
                      n824 = Enqueue Element(queue=w2473, element=w2472) -> (queue out=w2474:refnum<queue>)  [unwired: 2 in, 2 out]
                    }
                  }
                  frame True {
                    n825 = for {
                      shift-right: [w2479] -> w2476
                      shift-left: w2477 -> [w2480]
                      tunnel: string[] ["STOP", "RESET ENCODERS", "RESET FLAGS", "RESET YAW", "READ IR", "BOX COLOUR"] -> [w2478] mode=indexing
                      n826 = Enqueue Element(queue=w2480, element=w2478) -> (queue out=w2479:refnum<queue>)  [unwired: 2 in, 2 out]
                    }
                  }
                }
                n827 = Or(x=w2460, y=w2459) -> (x .or. y?=w2458:bool)
                n828 = Select(t=State_Type_Definitions,_for_0.26g_versions_and_later_2."True Stop" ("Enum"), s=w2459, f=State_Type_Definitions,_for_0.26g_versions_and_later_2."Task 9L: SCAN BOX 3" ("Enum")) -> (s? t:f=w2461:T18)
                n829 = Select(t=w2461, s=w2458, f=State_Type_Definitions,_for_0.26g_versions_and_later_2."Task 9K: MOVE RIGHT" ("Enum")) -> (s? t:f=w2467:T18)
              }
              frame "Exit" {
                n830 = for {
                  shift-right: [w2487] -> w2484
                  shift-left: w2483 -> [w2488]
                  tunnel: string[] ["STOP", "RESET ENCODERS", "RESET YAW", "ARDUINO MODE 0"] -> [w2486] mode=indexing
                  n831 = Enqueue Element(queue=w2488, element=w2486) -> (queue out=w2487:refnum<queue>)  [unwired: 2 in, 2 out]
                }
              }
            }
          }
          frame "Task 9L: SCAN BOX 3" {
            # ">>> Motor control cluster >>>"
            # ">>> yStepper command>>>"
            # ">> Item Selection Bias >>"
            n832 = Dequeue Element(queue=w2498, timeout in ms (-1)=w2497, error in (no error)=w2496) -> (element=w2502:T10)  [unwired: 3 out]
            n833 = call "Box Colour FGV.vi"("Init/R/W State"=Box_Colour_FGV_States."Read") -> ("Colour to detect (output)"=w2492:T2)  [unwired: 9 in, 1 out]
            n834 = Equal?(x=w2491, y=w2492) -> (x = y?=w2490:bool)
            n835 = case shown="\"Start Task 1\", Default" w2502 {
              tunnel: w2489 -> [w2510 _]
              tunnel: [w2517 State_Type_Definitions,_for_0.26g_versions_and_later_2."True Stop" ("Enum")] -> w2500
              tunnel: w2495 -> [w2506 _]
              tunnel: w2499 -> [w2516 w2533]
              tunnel: [w2515 w2534] -> w2494
              tunnel: [State_Type_Definitions,_for_0.26g_versions_and_later_2."Idle" ("Enum") State_Type_Definitions,_for_0.26g_versions_and_later_2."Shutdown" ("Enum")] -> w2501
              tunnel: w2490 -> [w2508 _]
              frame "Start Task 1", Default {
                n836 = case shown="False" w2510 {
                  tunnel: w2516 -> [w2520 w2527]
                  tunnel: [w2521 w2526] -> w2515
                  frame False {
                    n837 = for {
                      tunnel: string[] ["", "", "", ""] ("element") -> [w2522] mode=indexing
                      shift-right: [w2524] -> w2521
                      shift-left: w2520 -> [w2523]
                      n838 = Enqueue Element(queue=w2523, element=w2522) -> (queue out=w2524:refnum<queue>)  [unwired: 2 in, 2 out]
                    }
                  }
                  frame True {
                    n839 = for {
                      shift-right: [w2529] -> w2526
                      shift-left: w2527 -> [w2530]
                      tunnel: string[] ["STOP", "RESET ENCODERS", "RESET FLAGS", "RESET YAW", "", ""] -> [w2528] mode=indexing
                      n840 = Enqueue Element(queue=w2530, element=w2528) -> (queue out=w2529:refnum<queue>)  [unwired: 2 in, 2 out]
                    }
                  }
                }
                n841 = Or(x=w2510, y=w2506) -> (x .or. y?=w2509:bool)
                n842 = Or(x=w2508, y=w2506) -> (x .or. y?=w2507:bool)
                n843 = Select(t=State_Type_Definitions,_for_0.26g_versions_and_later_2."True Stop" ("Enum"), s=w2507, f=State_Type_Definitions,_for_0.26g_versions_and_later_2."True Stop" ("Enum")) -> (s? t:f=w2511:T18)
                n844 = Select(t=w2511, s=w2509, f=State_Type_Definitions,_for_0.26g_versions_and_later_2."Task 9L: SCAN BOX 3" ("Enum")) -> (s? t:f=w2517:T18)
              }
              frame "Exit" {
                n845 = for {
                  shift-right: [w2537] -> w2534
                  shift-left: w2533 -> [w2538]
                  tunnel: string[] ["STOP", "RESET ENCODERS", "RESET YAW", "ARDUINO MODE 0"] -> [w2536] mode=indexing
                  n846 = Enqueue Element(queue=w2538, element=w2536) -> (queue out=w2537:refnum<queue>)  [unwired: 2 in, 2 out]
                }
              }
            }
          }
          frame "Task 9M: MOVE RIGHT" {
            # ">> Item Selection Bias >>"
            n847 = Dequeue Element(queue=w2543, timeout in ms (-1)=w2542, error in (no error)=w2541) -> (element=w2548:T10)  [unwired: 3 out]
            n848 = case shown="\"Start Task 1\", Default" w2548 {
              tunnel: w2539 -> [w2554 _]
              tunnel: [w2561 State_Type_Definitions,_for_0.26g_versions_and_later_2."True Stop" ("Enum")] -> w2546
              tunnel: w2540 -> [w2553 _]
              tunnel: w2544 -> [w2560 w2577]
              tunnel: [w2559 w2578] -> w2545
              tunnel: [State_Type_Definitions,_for_0.26g_versions_and_later_2."Idle" ("Enum") State_Type_Definitions,_for_0.26g_versions_and_later_2."Shutdown" ("Enum")] -> w2547
              frame "Start Task 1", Default {
                n849 = case shown="False" w2554 {
                  tunnel: w2560 -> [w2564 w2571]
                  tunnel: [w2565 w2570] -> w2559
                  frame False {
                    n850 = for {
                      tunnel: string[] ["READ LINE SENSOR", "READ NAVX", "RIGHT", "READ ENCODERS"] ("element") -> [w2566] mode=indexing
                      shift-right: [w2568] -> w2565
                      shift-left: w2564 -> [w2567]
                      n851 = Enqueue Element(queue=w2567, element=w2566) -> (queue out=w2568:refnum<queue>)  [unwired: 2 in, 2 out]
                    }
                  }
                  frame True {
                    n852 = for {
                      shift-right: [w2573] -> w2570
                      shift-left: w2571 -> [w2574]
                      tunnel: string[] ["STOP", "RESET ENCODERS", "RESET YAW", "OPEN LIFE CAM", "SET TIMER 2", "RESET FLAGS"] -> [w2572] mode=indexing
                      n853 = Enqueue Element(queue=w2574, element=w2572) -> (queue out=w2573:refnum<queue>)  [unwired: 2 in, 2 out]
                    }
                  }
                }
                n854 = Or(x=w2554, y=w2553) -> (x .or. y?=w2552:bool)
                n855 = Select(t=State_Type_Definitions,_for_0.26g_versions_and_later_2."True Stop" ("Enum"), s=w2553, f=State_Type_Definitions,_for_0.26g_versions_and_later_2."Task 9N: SCAN BOX 4" ("Enum")) -> (s? t:f=w2555:T18)
                n856 = Select(t=w2555, s=w2552, f=State_Type_Definitions,_for_0.26g_versions_and_later_2."Task 9M: MOVE RIGHT" ("Enum")) -> (s? t:f=w2561:T18)
              }
              frame "Exit" {
                n857 = for {
                  shift-right: [w2581] -> w2578
                  shift-left: w2577 -> [w2582]
                  tunnel: string[] ["STOP", "RESET ENCODERS", "RESET YAW", "ARDUINO MODE 0"] -> [w2580] mode=indexing
                  n858 = Enqueue Element(queue=w2582, element=w2580) -> (queue out=w2581:refnum<queue>)  [unwired: 2 in, 2 out]
                }
              }
            }
          }
          frame "Task 9N: SCAN BOX 4" {
            # ">> Manual override >>"
            n859 = Dequeue Element(queue=w2591, timeout in ms (-1)=w2590, error in (no error)=w2589) -> (element=w2592:T10)  [unwired: 3 out]
            n860 = case shown="\"Start Task 1\", Default" w2592 {
              tunnel: [w2606 State_Type_Definitions,_for_0.26g_versions_and_later_2."True Stop" ("Enum")] -> w2584
              tunnel: [w2604 w2622] -> w2583
              tunnel: w2587 -> [w2603 w2619]
              tunnel: w2588 -> [w2597 _]
              tunnel: [State_Type_Definitions,_for_0.26g_versions_and_later_2."Idle" ("Enum") State_Type_Definitions,_for_0.26g_versions_and_later_2."Shutdown" ("Enum")] -> w2585
              tunnel: w2586 -> [w2596 _]
              frame "Start Task 1", Default {
                # ">> WIill proceed to part ii if not manual override >>"
                # ">>If ENABLE or Trigger is set to true>>"
                n861 = Or(x=w2596, y=w2597) -> (x .or. y?=w2598:bool)
                n862 = case shown="False" w2596 {
                  tunnel: [w2609 w2615] -> w2604
                  tunnel: w2603 -> [w2608 w2614]
                  frame False {
                    n863 = for {
                      shift-right: [w2611] -> w2609
                      shift-left: w2608 -> [w2612]
                      tunnel: string[] ["CAM ACQ", "START TIMER"] ("element") -> [w2610] mode=indexing
                      n864 = Enqueue Element(queue=w2612, element=w2610) -> (queue out=w2611:refnum<queue>)  [unwired: 2 in, 2 out]
                    }
                  }
                  frame True {
                    n865 = for {
                      shift-right: [w2617] -> w2615
                      shift-left: w2614 -> [w2618]
                      tunnel: string[] ["CLOSE CAM", "SET TIMER 5", "", "", "", ""] -> [w2616] mode=indexing
                      n866 = Enqueue Element(queue=w2618, element=w2616) -> (queue out=w2617:refnum<queue>)  [unwired: 2 in, 2 out]
                    }
                  }
                }
                n867 = Select(t=State_Type_Definitions,_for_0.26g_versions_and_later_2."True Stop" ("Enum"), s=w2597, f=State_Type_Definitions,_for_0.26g_versions_and_later_2."PENIS" ("Enum")) -> (s? t:f=w2600:T18)
                n868 = Select(t=w2600, s=w2598, f=State_Type_Definitions,_for_0.26g_versions_and_later_2."Task 9N: SCAN BOX 4" ("Enum")) -> (s? t:f=w2606:T18)
              }
              frame "Exit" {
                n869 = for {
                  shift-right: [w2625] -> w2622
                  shift-left: w2619 -> [w2626]
                  tunnel: string[] ["STOP", "RESET ENCODERS", "RESET YAW", ""] -> [w2624] mode=indexing
                  n870 = Enqueue Element(queue=w2626, element=w2624) -> (queue out=w2625:refnum<queue>)  [unwired: 2 in, 2 out]
                }
              }
            }
          }
          frame "PENIS" {
            # ">> Item Selection Bias >>"
            n871 = Dequeue Element(queue=w2634, timeout in ms (-1)=w2633, error in (no error)=w2632) -> (element=w2636:T10)  [unwired: 3 out]
            n872 = case shown="\"Start Task 1\", Default" w2636 {
              tunnel: w2627 -> [w2642 _]
              tunnel: [w2649 State_Type_Definitions,_for_0.26g_versions_and_later_2."True Stop" ("Enum")] -> w2630
              tunnel: w2631 -> [w2641 _]
              tunnel: w2635 -> [w2648 w2665]
              tunnel: [w2647 w2666] -> w2629
              tunnel: [State_Type_Definitions,_for_0.26g_versions_and_later_2."Idle" ("Enum") State_Type_Definitions,_for_0.26g_versions_and_later_2."Shutdown" ("Enum")] -> w2628
              frame "Start Task 1", Default {
                n873 = case shown="False" w2642 {
                  tunnel: w2648 -> [w2652 w2659]
                  tunnel: [w2653 w2658] -> w2647
                  frame False {
                    n874 = for {
                      tunnel: string[] ["START TIMER", "COLOUR PROCESSING", ""] ("element") -> [w2654] mode=indexing
                      shift-right: [w2656] -> w2653
                      shift-left: w2652 -> [w2655]
                      n875 = Enqueue Element(queue=w2655, element=w2654) -> (queue out=w2656:refnum<queue>)  [unwired: 2 in, 2 out]
                    }
                  }
                  frame True {
                    n876 = for {
                      shift-right: [w2661] -> w2658
                      shift-left: w2659 -> [w2662]
                      tunnel: string[] ["CLOSE CAM", "DISPOSE BUFFERS", "RESET ENCODERS", "RESET YAW", "RESET FLAGS", ""] -> [w2660] mode=indexing
                      n877 = Enqueue Element(queue=w2662, element=w2660) -> (queue out=w2661:refnum<queue>)  [unwired: 2 in, 2 out]
                    }
                  }
                }
                n878 = Or(x=w2642, y=w2641) -> (x .or. y?=w2640:bool)
                n879 = Select(t=State_Type_Definitions,_for_0.26g_versions_and_later_2."True Stop" ("Enum"), s=w2641, f=State_Type_Definitions,_for_0.26g_versions_and_later_2."PENIS 2" ("Enum")) -> (s? t:f=w2643:T18)
                n880 = Select(t=w2643, s=w2640, f=State_Type_Definitions,_for_0.26g_versions_and_later_2."PENIS" ("Enum")) -> (s? t:f=w2649:T18)
              }
              frame "Exit" {
                n881 = for {
                  shift-right: [w2669] -> w2666
                  shift-left: w2665 -> [w2670]
                  tunnel: string[] ["STOP", "RESET ENCODERS", "RESET YAW", "ARDUINO MODE 0"] -> [w2668] mode=indexing
                  n882 = Enqueue Element(queue=w2670, element=w2668) -> (queue out=w2669:refnum<queue>)  [unwired: 2 in, 2 out]
                }
              }
            }
          }
          frame "PENIS 2" {
            # ">> Item Selection Bias >>"
            n883 = Dequeue Element(queue=w2676, timeout in ms (-1)=w2675, error in (no error)=w2674) -> (element=w2684:T10)  [unwired: 3 out]
            n884 = Greater?(x=w2672, y=50.0) -> (0:w2682:bool)
            n885 = And(x=w2671, y=w2682) -> (x .and. y?=w2683:bool)
            n886 = case shown="\"Start Task 1\", Default" w2684 {
              tunnel: w2683 -> [w2690 _]
              tunnel: [w2697 State_Type_Definitions,_for_0.26g_versions_and_later_2."True Stop" ("Enum")] -> w2679
              tunnel: w2673 -> [w2689 _]
              tunnel: w2677 -> [w2696 w2713]
              tunnel: [w2695 w2714] -> w2678
              tunnel: [State_Type_Definitions,_for_0.26g_versions_and_later_2."Idle" ("Enum") State_Type_Definitions,_for_0.26g_versions_and_later_2."Shutdown" ("Enum")] -> w2680
              frame "Start Task 1", Default {
                n887 = case shown="False" w2690 {
                  tunnel: w2696 -> [w2700 w2707]
                  tunnel: [w2701 w2706] -> w2695
                  frame False {
                    n888 = for {
                      tunnel: string[] ["READ LINE SENSOR", "READ NAVX", "RIGHT", "READ ENCODERS"] ("element") -> [w2702] mode=indexing
                      shift-right: [w2704] -> w2701
                      shift-left: w2700 -> [w2703]
                      n889 = Enqueue Element(queue=w2703, element=w2702) -> (queue out=w2704:refnum<queue>)  [unwired: 2 in, 2 out]
                    }
                  }
                  frame True {
                    n890 = for {
                      shift-right: [w2709] -> w2706
                      shift-left: w2707 -> [w2710]
                      tunnel: string[] ["STOP", "RESET ENCODERS", "RESET YAW", "OPEN LIFE CAM", "SET TIMER 2", "RESET FLAGS"] -> [w2708] mode=indexing
                      n891 = Enqueue Element(queue=w2710, element=w2708) -> (queue out=w2709:refnum<queue>)  [unwired: 2 in, 2 out]
                    }
                  }
                }
                n892 = Or(x=w2690, y=w2689) -> (x .or. y?=w2688:bool)
                n893 = Select(t=State_Type_Definitions,_for_0.26g_versions_and_later_2."True Stop" ("Enum"), s=w2689, f=State_Type_Definitions,_for_0.26g_versions_and_later_2."PENIS 3" ("Enum")) -> (s? t:f=w2691:T18)
                n894 = Select(t=w2691, s=w2688, f=State_Type_Definitions,_for_0.26g_versions_and_later_2."PENIS 2" ("Enum")) -> (s? t:f=w2697:T18)
              }
              frame "Exit" {
                n895 = for {
                  shift-right: [w2717] -> w2714
                  shift-left: w2713 -> [w2718]
                  tunnel: string[] ["STOP", "RESET ENCODERS", "RESET YAW", "ARDUINO MODE 0"] -> [w2716] mode=indexing
                  n896 = Enqueue Element(queue=w2718, element=w2716) -> (queue out=w2717:refnum<queue>)  [unwired: 2 in, 2 out]
                }
              }
            }
          }
          frame "PENIS 3" {
            # ">> Manual override >>"
            n897 = Dequeue Element(queue=w2727, timeout in ms (-1)=w2726, error in (no error)=w2725) -> (element=w2728:T10)  [unwired: 3 out]
            n898 = case shown="\"Start Task 1\", Default" w2728 {
              tunnel: [w2742 State_Type_Definitions,_for_0.26g_versions_and_later_2."True Stop" ("Enum")] -> w2720
              tunnel: [w2740 w2758] -> w2719
              tunnel: w2723 -> [w2739 w2755]
              tunnel: w2724 -> [w2733 _]
              tunnel: [State_Type_Definitions,_for_0.26g_versions_and_later_2."Idle" ("Enum") State_Type_Definitions,_for_0.26g_versions_and_later_2."Shutdown" ("Enum")] -> w2721
              tunnel: w2722 -> [w2732 _]
              frame "Start Task 1", Default {
                # ">> WIill proceed to part ii if not manual override >>"
                # ">>If ENABLE or Trigger is set to true>>"
                n899 = Or(x=w2732, y=w2733) -> (x .or. y?=w2734:bool)
                n900 = case shown="False" w2732 {
                  tunnel: [w2745 w2751] -> w2740
                  tunnel: w2739 -> [w2744 w2750]
                  frame False {
                    n901 = for {
                      shift-right: [w2747] -> w2745
                      shift-left: w2744 -> [w2748]
                      tunnel: string[] ["CAM ACQ", "START TIMER"] ("element") -> [w2746] mode=indexing
                      n902 = Enqueue Element(queue=w2748, element=w2746) -> (queue out=w2747:refnum<queue>)  [unwired: 2 in, 2 out]
                    }
                  }
                  frame True {
                    n903 = for {
                      shift-right: [w2753] -> w2751
                      shift-left: w2750 -> [w2754]
                      tunnel: string[] ["CLOSE CAM", "SET TIMER 5", "", "", "", ""] -> [w2752] mode=indexing
                      n904 = Enqueue Element(queue=w2754, element=w2752) -> (queue out=w2753:refnum<queue>)  [unwired: 2 in, 2 out]
                    }
                  }
                }
                n905 = Select(t=State_Type_Definitions,_for_0.26g_versions_and_later_2."True Stop" ("Enum"), s=w2733, f=State_Type_Definitions,_for_0.26g_versions_and_later_2."Task 9R: PROCESS COLOUR" ("Enum")) -> (s? t:f=w2736:T18)
                n906 = Select(t=w2736, s=w2734, f=State_Type_Definitions,_for_0.26g_versions_and_later_2."PENIS 3" ("Enum")) -> (s? t:f=w2742:T18)
              }
              frame "Exit" {
                n907 = for {
                  shift-right: [w2761] -> w2758
                  shift-left: w2755 -> [w2762]
                  tunnel: string[] ["STOP", "RESET ENCODERS", "RESET YAW", ""] -> [w2760] mode=indexing
                  n908 = Enqueue Element(queue=w2762, element=w2760) -> (queue out=w2761:refnum<queue>)  [unwired: 2 in, 2 out]
                }
              }
            }
          }
          frame "Task 9R: PROCESS COLOUR" {
            # ">> Item Selection Bias >>"
            # ">>> Motor control cluster >>>"
            # ">>> yStepper command>>>"
            n909 = Dequeue Element(queue=w2768, timeout in ms (-1)=w2769, error in (no error)=w2770) -> (element=w2772:T10)  [unwired: 3 out]
            n910 = case shown="\"Start Task 1\", Default" w2772 {
              tunnel: w2766 -> [w2778 _]
              tunnel: [w2785 State_Type_Definitions,_for_0.26g_versions_and_later_2."True Stop" ("Enum")] -> w2764
              tunnel: w2771 -> [w2777 _]
              tunnel: w2767 -> [w2784 w2801]
              tunnel: [w2783 w2802] -> w2763
              tunnel: [State_Type_Definitions,_for_0.26g_versions_and_later_2."Idle" ("Enum") State_Type_Definitions,_for_0.26g_versions_and_later_2."Shutdown" ("Enum")] -> w2765
              frame "Start Task 1", Default {
                n911 = case shown="False" w2778 {
                  tunnel: w2784 -> [w2788 w2795]
                  tunnel: [w2789 w2794] -> w2783
                  frame False {
                    n912 = for {
                      tunnel: string[] ["START TIMER", "COLOUR PROCESSING", ""] ("element") -> [w2790] mode=indexing
                      shift-right: [w2792] -> w2789
                      shift-left: w2788 -> [w2791]
                      n913 = Enqueue Element(queue=w2791, element=w2790) -> (queue out=w2792:refnum<queue>)  [unwired: 2 in, 2 out]
                    }
                  }
                  frame True {
                    n914 = for {
                      shift-right: [w2797] -> w2794
                      shift-left: w2795 -> [w2798]
                      tunnel: string[] ["CLOSE CAM", "DISPOSE BUFFERS", "RESET ENCODERS", "RESET YAW", "RESET FLAGS", ""] -> [w2796] mode=indexing
                      n915 = Enqueue Element(queue=w2798, element=w2796) -> (queue out=w2797:refnum<queue>)  [unwired: 2 in, 2 out]
                    }
                  }
                }
                n916 = Or(x=w2778, y=w2777) -> (x .or. y?=w2776:bool)
                n917 = Select(t=State_Type_Definitions,_for_0.26g_versions_and_later_2."True Stop" ("Enum"), s=w2777, f=State_Type_Definitions,_for_0.26g_versions_and_later_2."True Stop" ("Enum")) -> (s? t:f=w2779:T18)
                n918 = Select(t=w2779, s=w2776, f=State_Type_Definitions,_for_0.26g_versions_and_later_2."Task 9R: PROCESS COLOUR" ("Enum")) -> (s? t:f=w2785:T18)
              }
              frame "Exit" {
                n919 = for {
                  shift-right: [w2805] -> w2802
                  shift-left: w2801 -> [w2806]
                  tunnel: string[] ["STOP", "RESET ENCODERS", "RESET YAW", "ARDUINO MODE 0"] -> [w2804] mode=indexing
                  n920 = Enqueue Element(queue=w2806, element=w2804) -> (queue out=w2805:refnum<queue>)  [unwired: 2 in, 2 out]
                }
              }
            }
          }
          frame "Task A1: Task 9 Open cam" {
            # ">>> Motor control cluster >>>"
            # ">>> yStepper command>>>"
            # ">> Manual override >>"
            n921 = Dequeue Element(queue=w2818, timeout in ms (-1)=w2814, error in (no error)=w2817) -> (element=w2819:T10)  [unwired: 3 out]
            n922 = case shown="\"Start Task 1\", Default" w2819 {
              tunnel: [w2830 State_Type_Definitions,_for_0.26g_versions_and_later_2."True Stop" ("Enum")] -> w2812
              tunnel: [w2828 w2845] -> w2811
              tunnel: w2815 -> [w2827 _]
              tunnel: w2816 -> [w2821 _]
              tunnel: [State_Type_Definitions,_for_0.26g_versions_and_later_2."Idle" ("Enum") State_Type_Definitions,_for_0.26g_versions_and_later_2."Shutdown" ("Enum")] -> w2813
              tunnel: w2807 -> [w2820 _]
              frame "Start Task 1", Default {
                # ">> WIill proceed to part ii if not manual override >>"
                # ">>If ENABLE or Trigger is set to true>>"
                n923 = Or(x=w2820, y=w2821) -> (x .or. y?=w2822:bool)
                n924 = case shown="False" w2820 {
                  tunnel: [w2833 w2839] -> w2828
                  tunnel: w2827 -> [w2832 w2838]
                  frame False {
                    n925 = for {
                      shift-right: [w2835] -> w2833
                      shift-left: w2832 -> [w2836]
                      tunnel: string[] ["Task 9", ""] ("element") -> [w2834] mode=indexing
                      n926 = Enqueue Element(queue=w2836, element=w2834) -> (queue out=w2835:refnum<queue>)  [unwired: 2 in, 2 out]
                    }
                  }
                  frame True {
                    n927 = for {
                      shift-right: [w2841] -> w2839
                      shift-left: w2838 -> [w2842]
                      tunnel: string[] ["ARDUINO - ULTRASONIC", "READ NAVX", "RESET FLAGS", "", "", ""] -> [w2840] mode=indexing
                      n928 = Enqueue Element(queue=w2842, element=w2840) -> (queue out=w2841:refnum<queue>)  [unwired: 2 in, 2 out]
                    }
                  }
                }
                n929 = Select(t=State_Type_Definitions,_for_0.26g_versions_and_later_2."True Stop" ("Enum"), s=w2821, f=State_Type_Definitions,_for_0.26g_versions_and_later_2."True Stop" ("Enum")) -> (s? t:f=w2824:T18)
                n930 = Select(t=w2824, s=w2822, f=State_Type_Definitions,_for_0.26g_versions_and_later_2."Task A1: Task 9 Open cam" ("Enum")) -> (s? t:f=w2830:T18)
              }
              frame "Exit" {
                n931 = for {
                  shift-right: [w2848] -> w2845
                  shift-left: _ -> [w2849]
                  tunnel: string[] ["STOP", "RESET ENCODERS", "RESET YAW", ""] -> [w2847] mode=indexing
                  n932 = Enqueue Element(queue=w2849, element=w2847) -> (queue out=w2848:refnum<queue>)  [unwired: 2 in, 2 out]
                }
              }
            }
          }
          frame "Task A2: Task 9 Move Arm" {
            # ">>> Motor control cluster >>>"
            # ">>> yStepper command>>>"
            n933 = Dequeue Element(queue=w2863, timeout in ms (-1)=w2862, error in (no error)=w2861) -> (element=w2865:T10)  [unwired: 3 out]
            n934 = In Range and Coerce(upper limit=65.0, x=w2855, lower limit=58.0) -> (In Range?=w2852:bool)  [unwired: 1 out]
            n935 = case shown="\"Start Task 1\", Default" w2865 {
              tunnel: w2856 -> [w2868 _]
              tunnel: [w2876 State_Type_Definitions,_for_0.26g_versions_and_later_2."True Stop" ("Enum")] -> w2858
              tunnel: w2864 -> [w2874 w2892]
              tunnel: [w2873 w2891] -> w2857
              tunnel: [State_Type_Definitions,_for_0.26g_versions_and_later_2."Idle" ("Enum") State_Type_Definitions,_for_0.26g_versions_and_later_2."Shutdown" ("Enum")] -> w2859
              tunnel: w2852 -> [w2866 _]
              frame "Start Task 1", Default {
                n936 = Or(x=w2866, y=w2868) -> (x .or. y?=w2867:bool)
                n937 = case shown="True" w2866 {
                  tunnel: w2874 -> [w2879 w2885]
                  tunnel: [w2878 w2883] -> w2873
                  frame False {
                    n938 = for {
                      shift-right: [w2881] -> w2878
                      shift-left: w2879 -> [w2882]
                      tunnel: string[] ["READ NAVX", "R-CW", "READ ULTRASONIC"] ("element") -> [w2880] mode=indexing
                      n939 = Enqueue Element(queue=w2882, element=w2880) -> (queue out=w2881:refnum<queue>)  [unwired: 2 in, 2 out]
                    }
                  }
                  frame True {
                    n940 = for {
                      shift-right: [w2887] -> w2883
                      shift-left: w2885 -> [w2888]
                      tunnel: string[] ["STOP", "RESET ENCODERS", "RESET YAW", "READ IR", "ARDUINO - ULTRASONIC"] -> [w2886] mode=indexing
                      n941 = Enqueue Element(queue=w2888, element=w2886) -> (queue out=w2887:refnum<queue>)  [unwired: 2 in, 2 out]
                    }
                  }
                }
                n942 = Select(t=State_Type_Definitions,_for_0.26g_versions_and_later_2."True Stop" ("Enum"), s=w2868, f=State_Type_Definitions,_for_0.26g_versions_and_later_2."Task A3: Task 9 Set Timer") -> (s? t:f=w2870:T18)
                n943 = Select(t=w2870, s=w2867, f=State_Type_Definitions,_for_0.26g_versions_and_later_2."Task A2: Task 9 Move Arm" ("Enum")) -> (s? t:f=w2876:T18)
              }
              frame "Exit" {
                n944 = for {
                  shift-right: [w2895] -> w2891
                  shift-left: w2892 -> [w2896]
                  tunnel: string[] ["STOP", "RESET ENCODERS", "RESET YAW", ""] -> [w2894] mode=indexing
                  n945 = Enqueue Element(queue=w2896, element=w2894) -> (queue out=w2895:refnum<queue>)  [unwired: 2 in, 2 out]
                }
              }
            }
          }
          frame "Task A3: Task 9 Set Timer" {
            (unwired) 50.0 ("y")
            (unwired) 15.0 ("y")
            # ">> Item Selection Bias >>"
            # ">> Wall detected >>"
            # ">> Manual override >>"
            # ">>> Motor control cluster >>>"
            # ">>Table or wall detectected>>"
            # ">>Action Queue>>"
            # ">>> yStepper command>>>"
            n946 = Dequeue Element(queue=w2912, timeout in ms (-1)=w2911, error in (no error)=w2910) -> (element=w2913:T10)  [unwired: 3 out]
            n947 = Less?(x=w2899, y=100.0) -> (x < y?=w2900:bool)
            n948 = Not Equal To 0?(x=w2899) -> (x != 0?=w2898:bool)
            n949 = And(x=w2898, y=w2900) -> (x .and. y?=w2897:bool)
            n950 = case shown="\"Start Task 1\", Default" w2913 {
              tunnel: w2908 -> [w2914 _]
              tunnel: [w2924 State_Type_Definitions,_for_0.26g_versions_and_later_2."True Stop" ("Enum")] -> w2905
              tunnel: w2909 -> [w2922 w2940]
              tunnel: [w2921 w2939] -> w2904
              tunnel: [State_Type_Definitions,_for_0.26g_versions_and_later_2."Idle" ("Enum") State_Type_Definitions,_for_0.26g_versions_and_later_2."Shutdown" ("Enum")] -> w2907
              tunnel: w2897 -> [w2915 _]
              frame "Start Task 1", Default {
                n951 = Or(x=w2914, y=w2915) -> (x .or. y?=w2916:bool)
                n952 = case shown="False" w2915 {
                  tunnel: w2922 -> [w2927 w2933]
                  tunnel: [w2926 w2931] -> w2921
                  frame False {
                    n953 = for {
                      shift-right: [w2929] -> w2926
                      shift-left: w2927 -> [w2930]
                      tunnel: string[] ["READ IR", "FORWARD - IR ASSIST", "READ ULTRASONIC"] ("element") -> [w2928] mode=indexing
                      n954 = Enqueue Element(queue=w2930, element=w2928) -> (queue out=w2929:refnum<queue>)  [unwired: 2 in, 2 out]
                    }
                  }
                  frame True {
                    n955 = for {
                      shift-right: [w2935] -> w2931
                      shift-left: w2933 -> [w2936]
                      tunnel: string[] ["STOP", "RESET ENCODERS", "RESET YAW", ""] -> [w2934] mode=indexing
                      n956 = Enqueue Element(queue=w2936, element=w2934) -> (queue out=w2935:refnum<queue>)  [unwired: 2 in, 2 out]
                    }
                  }
                }
                n957 = Select(t=State_Type_Definitions,_for_0.26g_versions_and_later_2."True Stop" ("Enum"), s=w2914, f=State_Type_Definitions,_for_0.26g_versions_and_later_2."Task A4: Tasl 9 Capture images") -> (s? t:f=w2918:T18)
                n958 = Select(t=w2918, s=w2916, f=State_Type_Definitions,_for_0.26g_versions_and_later_2."Task A3: Task 9 Set Timer" ("Enum")) -> (s? t:f=w2924:T18)
              }
              frame "Exit" {
                n959 = for {
                  shift-right: [w2943] -> w2939
                  shift-left: w2940 -> [w2944]
                  tunnel: string[] ["STOP", "RESET ENCODERS", "RESET YAW", ""] -> [w2942] mode=indexing
                  n960 = Enqueue Element(queue=w2944, element=w2942) -> (queue out=w2943:refnum<queue>)  [unwired: 2 in, 2 out]
                }
              }
            }
          }
          frame "Task A4: Tasl 9 Capture images" {
            # ">>> Motor control cluster >>>"
            # ">>> yStepper command>>>"
            # ">> Item Selection Bias >>"
            n961 = Less?(x=w2948, y=-40.0) -> (x < y?=w2946:bool)
            n962 = Dequeue Element(queue=w2954, timeout in ms (-1)=w2953, error in (no error)=w2952) -> (element=w2956:T10)  [unwired: 3 out]
            n963 = case shown="\"Start Task 1\", Default" w2956 {
              tunnel: w2946 -> [w2962 _]
              tunnel: [w2969 State_Type_Definitions,_for_0.26g_versions_and_later_2."True Stop" ("Enum")] -> w2950
              tunnel: w2951 -> [w2961 _]
              tunnel: w2955 -> [w2968 w2985]
              tunnel: [w2967 w2986] -> w2945
              tunnel: [State_Type_Definitions,_for_0.26g_versions_and_later_2."Idle" ("Enum") State_Type_Definitions,_for_0.26g_versions_and_later_2."Shutdown" ("Enum")] -> w2949
              frame "Start Task 1", Default {
                n964 = case shown="True" w2962 {
                  tunnel: w2968 -> [w2972 w2979]
                  tunnel: [w2973 w2978] -> w2967
                  frame False {
                    n965 = for {
                      tunnel: string[] ["READ ENCODERS", "R-CW"] ("element") -> [w2974] mode=indexing
                      shift-right: [w2976] -> w2973
                      shift-left: w2972 -> [w2975]
                      n966 = Enqueue Element(queue=w2975, element=w2974) -> (queue out=w2976:refnum<queue>)  [unwired: 2 in, 2 out]
                    }
                  }
                  frame True {
                    n967 = for {
                      shift-right: [w2981] -> w2978
                      shift-left: w2979 -> [w2982]
                      tunnel: string[] ["STOP", "RESET ENCODERS", "RESET FLAGS", "RESET YAW", "READ IR", ""] -> [w2980] mode=indexing
                      n968 = Enqueue Element(queue=w2982, element=w2980) -> (queue out=w2981:refnum<queue>)  [unwired: 2 in, 2 out]
                    }
                  }
                }
                n969 = Or(x=w2962, y=w2961) -> (x .or. y?=w2960:bool)
                n970 = Select(t=State_Type_Definitions,_for_0.26g_versions_and_later_2."True Stop" ("Enum"), s=w2961, f=State_Type_Definitions,_for_0.26g_versions_and_later_2."Task A3: Task 9 Set Timer" ("Enum")) -> (s? t:f=w2963:T18)
                n971 = Select(t=w2963, s=w2960, f=State_Type_Definitions,_for_0.26g_versions_and_later_2."Task A4: Tasl 9 Capture images" ("Enum")) -> (s? t:f=w2969:T18)
              }
              frame "Exit" {
                n972 = for {
                  shift-right: [w2989] -> w2986
                  shift-left: w2985 -> [w2990]
                  tunnel: string[] ["STOP", "RESET ENCODERS", "RESET YAW", "ARDUINO MODE 0"] -> [w2988] mode=indexing
                  n973 = Enqueue Element(queue=w2990, element=w2988) -> (queue out=w2989:refnum<queue>)  [unwired: 2 in, 2 out]
                }
              }
            }
          }
        }
        "Object Detection" <- w336
        "Ultrasonic sensors" <- w359
        "Encoder values" <- w348
        "Stepper position values" <- w332
        "NAVX Values" <- w330
        "IR Sensors" <- w322
        "Line sensors" <- w317
        "Time cluster" <- w328
        "Box Colour Detection" <- w310
      }
    }
    "Object recognition mode" <- w234
    "Front Ultrasonic obstruct" <- w231
    "Front IR obstruct" <- w230
    "Table IR obstruct" <- w229
    "Same colour?" <- w224
    n974 = local write "Green LED"(w244) -> ()
  }
  n975 = while {
    stop <- w3901 stop-if-true
    n976 = call "MOTOR CONTROL WITH PID AE.vi"("AE Mode"=MOTOR_CONTROL_WITH_PID_AE_DATA_MODE_TYPE_DEF."Read from AE") -> ("Speed & distance"=→"Speed & distance":T15)  [unwired: 3 in]
    n977 = call "FGV Bool.vi"("Init/Read/Write State"=States_for_Action_Engine."Read") -> ("Output node"=w3901:bool)  [unwired: 2 in, 1 out]
    n978 = Wait (ms)(milliseconds to wait=u32 5) -> ()  [unwired: 1 out]
  }
  n979 = call <vilib>:"DIO Close.vi"("error in (no error)"=w23, "DIO Info In"=w26) -> ()  [unwired: 9 in, 1 out]
  n980 = call <vilib>:"DIO Close.vi"("error in (no error)"=w33, "DIO Info In"=w35) -> ()  [unwired: 9 in, 1 out]
  n981 = call <vilib>:"NavX Close.vi"("error in (no error)"=w10, "NavX Info In"=w9) -> ()  [unwired: 9 in, 1 out]
  n982 = call <vilib>:"DIO Close.vi"("error in (no error)"=w28, "DIO Info In"=w30) -> ()  [unwired: 9 in, 1 out]
  n983 = call <vilib>:"DIO Close.vi"("error in (no error)"=w17, "DIO Info In"=w18) -> ()  [unwired: 9 in, 1 out]
  n984 = call <vilib>:"DIO Close.vi"("error in (no error)"=w12, "DIO Info In"=w13) -> ()  [unwired: 9 in, 1 out]
  n985 = Merge Errors "Merge Errors"(w63, w62) -> (w45:errorcluster)
  n986 = Merge Errors(w49, w45) -> (w44:errorcluster)
  n987 = Destroy User Event(user event=w67, error in=w44) -> ()  [unwired: 1 out]
  n988 = Release Queue(queue=w40, error in (no error)=w44) -> (error out=→"Queue Errors":errorcluster)  [unwired: 1 in, 2 out]
  n989 = Release Queue(queue=w57, error in (no error)=w44) -> ()  [unwired: 1 in, 3 out]
  n990 = Destroy User Event(user event=w66, error in=w44) -> ()  [unwired: 1 out]
  n991 = Unregister For Events(event registration refnum=w58, error in=w44) -> ()  [unwired: 1 out]
